vi "COD主界面（列队使用）.vi"() -> (8 "多列列表框":i32(listbox))   [LabVIEW 2016, in "斯坦道CODMn.lvlib"]
uses:
  <vilib>/Analysis/6fits.llb/Curve Fitting Criteria.ctl
  <vilib>/Utility/miscctls.llb/LVPointTypeDef.ctl
  <vilib>/Utility/config.llb/Read Key (I32).vi
  <vilib>/Utility/config.llb/Read Key (Double).vi
  <vilib>/Utility/config.llb/Read Key (Boolean).vi
  <vilib>/Utility/config.llb/Write Key (I32).vi
  <vilib>/Utility/config.llb/Read Key (String).vi
  <vilib>/Utility/config.llb/Write Key (Double).vi
  <vilib>/Utility/config.llb/Write Key (Boolean).vi
  <vilib>/Utility/config.llb/Write Key (String).vi
  <vilib>/Waveform/WDTFileIO.llb/Read Waveform from File.vi
  <vilib>/ptbypt/NI_PtbyPt.lvlib
  <vilib>/Utility/config.llb/NI_LVConfig.lvlib
  <vilib>/Analysis/NI_AALPro.lvlib
panel:
  in  "零点液自动补测":bool
  in  "跨度液自动补测":bool
  in  "标准液自动补测":bool
  in  "零点液偏差":dbl
  in  "跨度液偏差":dbl
  in  "标准液偏差":dbl
  in  "更换泵管":bool
  out "消解压力kPa":dbl format="%#.2f"
  out "权限等级":string
  in  "布尔":bool
  in  "屏蔽负值":bool
  in  "方程系数 2":cluster{"K":dbl, "b":dbl, "X^2":dbl} {"X^2" format="%#.6g"; "b" format="%#.6g"; "K" format="%#.6g"}
  out "r^2 2":dbl caption="r^2" format="%.8g"
  out "拟合公式 2":string
  in  "跨度值":dbl
  in  "公式切换阈值滴定数(0-9999)":u16
  out "公式系数":dbl[](array[numeric])
  in  "存校准信息":bool
  out "标液校准时间4":timestamp format="%<%Y/%m/%d %H:%M:%S>T"
  out "标液校准时间3":timestamp format="%<%Y/%m/%d %H:%M:%S>T"
  out "标液校准时间2":timestamp format="%<%Y/%m/%d %H:%M:%S>T"
  out "标液校准时间1":timestamp format="%<%Y/%m/%d %H:%M:%S>T"
  out "零点校准时间":timestamp format="%<%Y/%m/%d %H:%M:%S>T"
  in  "远程标样校准":enum16{"标液1", "标液2", "标液3", "标液4"}(ring)
  in  "远程校准量程":enum16{"低量程", "高量程"}(ring)
  in  "温度曲线":bool
  out "温度波形时间":timestamp
  in  "历史波形 2":bool
  out "时间-温度":u16[](array[numeric]) caption="数组"
  in  "关闭 4":bool
  out "时间温度曲线":u16[](graph)
  in  "加标回收量程：":enum32{"H", "L", "AUTO"}(ring)=enum."AUTO"
  in  "定时设置":cluster{"启动":bool, "控制命令":T1, "测量参数":T2}(xcontrol)
  out "氢氧化钠":dbl
  in  "序列号变更":bool
  out "模块版本号":string
  in  "更新程序":bool
  out "进样无液体告警":bool
  out "校准内容显示":string
  out "60分钟超时报警":bool
  in  "仪器参数":bool
  out "CODMn序列号":string
  out "CODMn软件版本：":string
  in  "标样核查量程选择":enum32{"H", "L", "AUTO"}(ring)=enum."AUTO"
  in  "标样浓度":dbl
  in  "零点核查量程选择":enum32{"H", "L", "AUTO"}(ring)=enum."AUTO"
  in  "零点核查浓度":dbl
  out "序列号":string
  in  "采水泵排液时间/s:":i32
  in  "采水泵润洗时间/s:":i32
  in  "采水泵沉淀时间/s:":i32
  in  "采水泵进样时间/s:":i32
  in  "常规版/认证版":enum16{"常规版-酸性", "常规版-碱性", "认证版", "浮台版"}(ring)
  in  "释放串口":bool
  in  "打开串口":bool
  in  "保存参数":dbl[](array[numeric])
  out "报警数字":i16
  out "CODMn工作状态":T3(ring)
  out "ORP-K":string
  out "ORP-B":string
  out "ORP-A":string
  out "稀释倍数解释":string
  in  "跨度量程选择":enum32{"H", "L", "AUTO"}(ring)=enum."AUTO"
  in  "跨度液浓度":dbl
  in  "水样：":dbl
  in  "蒸馏水：":dbl
  in  "标液：":dbl
  in  "零点核查样：":dbl
  in  "加标回收样：":dbl
  in  "草酸钠":dbl
  in  "高锰酸钾":dbl
  in  "硫酸":dbl
  out "量程解释说明":string
  in  "高切低阈值:":dbl
  in  "低切高阈值:":dbl
  in  "水样量程选择:":enum16{"L", "H", "自动切换测一次", "自动切换测两次"}(ring)
  in  "氢氧化钠：":dbl
  in  "标准液浓度":dbl
  in  "温度":dbl
  in  "恒温时间":dbl
  in  "当前量程：":enum16{"L", "H"}(ring)
  in  "CODMn零点核查选择":enum16{"零点核查走纯水管", "零点核查走零漂管"}(ring)
  in  "低量程稀释倍数:":i8=1
  in  "高量程稀释倍数:":i8=2
  out "基本量程(显示)":string
  out "测量模式(显示)":string
  out "数据时间":string
  out "断电排液标记":bool
  out "COM":string
  in  "启用5":bool
  in  "校准5":bool
  in  "泵滴定数5":dbl
  in  "浓度5":dbl
  in  "启用4":bool
  in  "校准4":bool
  in  "泵滴定数4":dbl
  in  "浓度4":dbl
  out "波形时间":timestamp
  in  "历史波形":bool
  out "滴定数-ORP值":u16[](array[numeric]) caption="数组"
  in  "关闭 3":bool
  in  "滴定曲线":bool
  out "ORP滴定曲线":u16[](graph)
  out "空白测试标记":bool
  out "跨度核查标记":bool
  in  "量程选择":enum16{"低量程", "高量程"}(ring)
  in  "手动控制":bool
  in  "选用水样":enum16{"葡萄糖", "草酸钠"}(ring)
  in  "方程系数":cluster{"K":dbl, "b":dbl, "X^2":dbl} {"X^2" format="%#.6g"; "b" format="%#.6g"; "K" format="%#.6g"}
  out "XY图":cluster{"X Values":dbl[], "Y Values":dbl[]}[](graph)
  in  "模型":enum32{"线性", "多项式", "折线"}(ring)
  out "启动时间":timestamp format="%<%Y/%m/%d %H:%M:%S>T"
  out "r^2":dbl format="%.8g"
  out "拟合公式":string
  in  "启用3":bool
  in  "启用2":bool
  in  "启用1":bool
  in  "校准3":bool
  in  "校准2":bool
  in  "校准1":bool
  in  "泵滴定数3":dbl
  in  "泵滴定数2":dbl
  in  "泵滴定数1":dbl
  in  "浓度3":dbl
  in  "浓度2":dbl
  in  "浓度1":dbl
  in  "写入":bool
  out "零点核查标记":bool
  out "排液故障":bool
  out "进水样超量程":bool
  out "标样核查标记":bool
  out "平行样测量":bool
  out "加标回收测量":bool
  out "质控样测量":bool
  out "待机":bool
  out "校标错误":bool
  out "校零错误":bool
  out "测量错误":bool
  out "草酸钠报警":bool
  out "高锰酸钾报警":bool
  out "加热故障":bool
  out "温控器故障":bool
  out "ORP故障":bool
  out "排液标记":bool
  out "故障标记":bool
  out "校标标记":bool
  out "校零标记":bool
  out "通讯状态":bool
  out "水样测量":bool
  in  "读取":bool
  in  "返回":bool
  in  "校准配置":bool
  in  "零点泵计量数 2":dbl
  in  "标度泵计量数 2":dbl
  out "标度滴定值":dbl
  out "零点滴定值":dbl
  in  "保存":bool
  in  "关闭":bool
  out "仪器时间":timestamp format="%<%Y/%m/%d %H:%M:%S>T"
  out "秒":u16
  out "分":u16
  out "COD浓度（mg/L)":dbl format="%.2g"
  out "进样管":dbl
  out "高锰酸钾":dbl
  out "草酸钠":dbl
  out "硫酸":dbl
  out "实时ORP":dbl
  out "消解温度℃":dbl
  out "加热":bool
  out "搅拌":bool
  out "进硫酸":bool
  out "进加标回收样":bool
  out "进零点核查样":bool
  out "进标液":bool
  out "进蒸馏水":bool
  out "进水样":bool
  out "进草酸钠":bool
  out "进高锰酸钾":bool
  in  "启动":bool
  in  "故障清除":bool
  in  "参数配置":bool
  in  "停止":bool
  in  "单步启动":bool
  out "系统时间":timestamp
  in  "时间校准":bool
  out "模式（受控）":u16
  # "测试时长："
  # "注：遇到加热故障和排液故障时仪器不能正常启动，\n必须排查故障并点击报警清除按钮方可运行。"
  # "mg/L"
  # "基本参数设置"
  # "校零校标结果"
  # "泵计量参数设置"
  # "校零结果："
  # "校零滴定值："
  # "高锰酸钾："
  # "加热恒温温度(℃):"
  # "草酸钠："
  # "校标结果："
  # "标度滴定值："
  # "恒温时间(分钟):"
  # "零点泵计量值："
  # "硫酸："
  # "标准液浓度(mg/L):"
  # "标度泵计量值："
  # "跨度核查浓度："
  # "跨度核查量程："
  # "日质控自动补测设置"
  # "标准液偏差±:"
  # "零点核查浓度："
  # "标样浓度："
  # "跨度液偏差%:"
  # "零点核查量程："
  # "标样核查量程："
  # "零点液偏差%:"
  # "跨度值:"
  # "校准配置界面"
  # "测量信号值"
  # "启用"
  # "校准时间"
  # "浓度"
  # "零点"
  # "标液1"
  # "标液2"
  # "标液3"
  # "标液4"
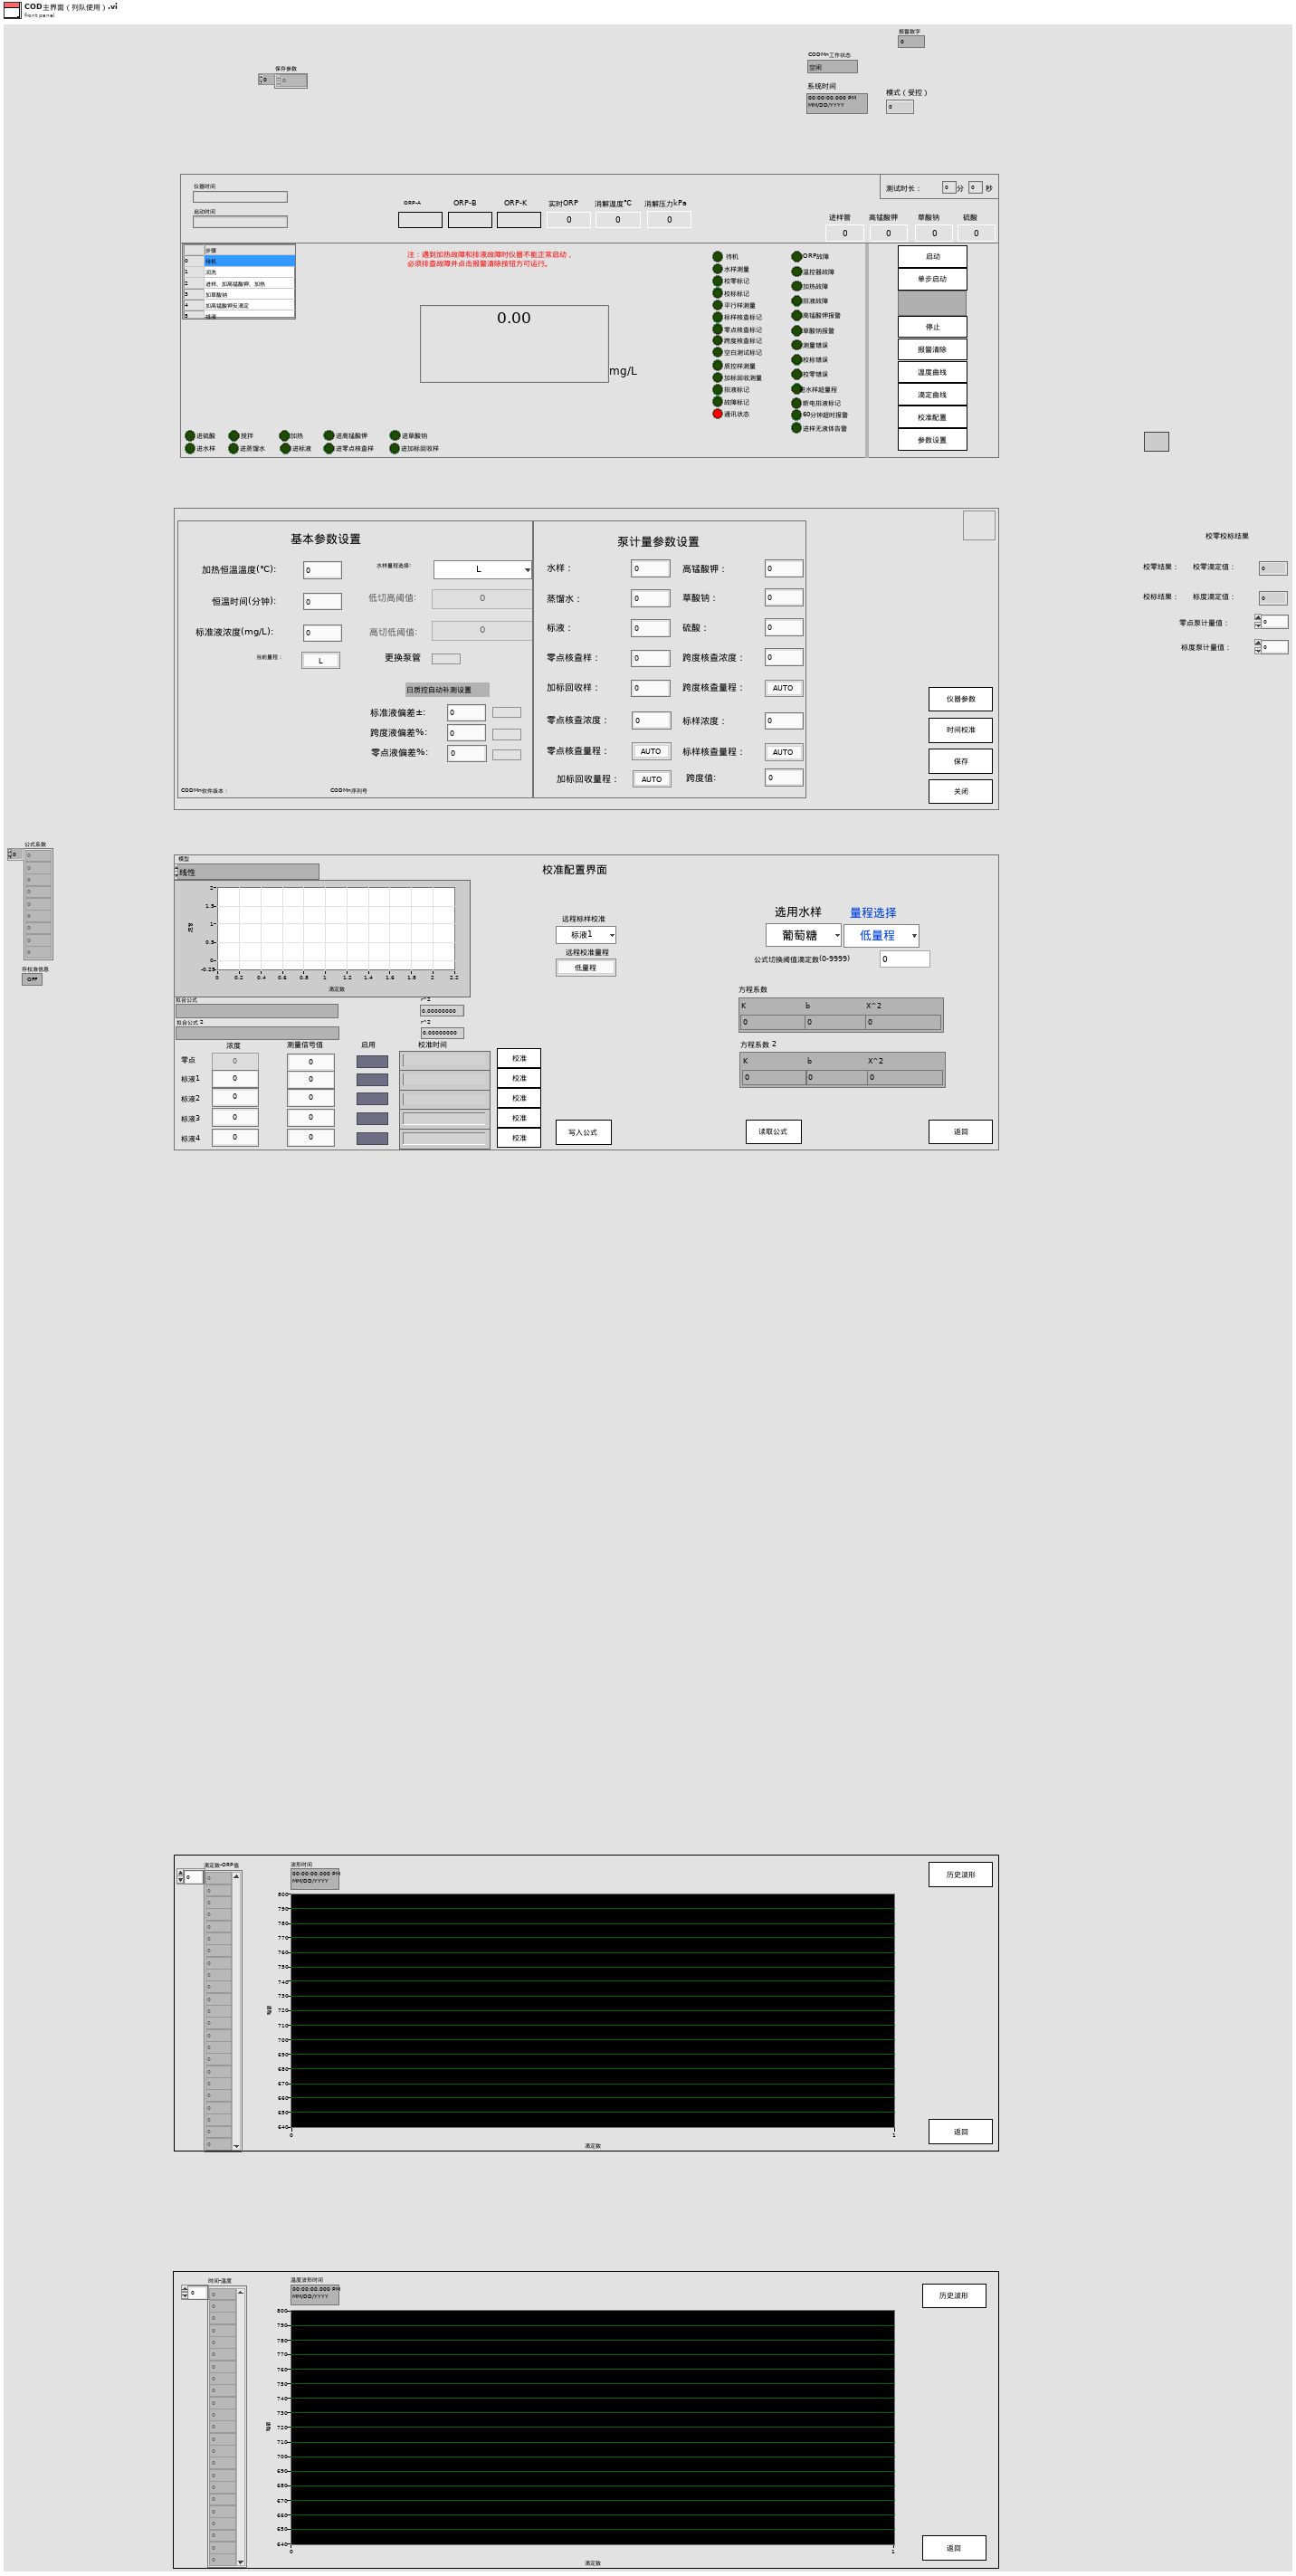
[diagram p1: front panel]
types:
  T1 = typedef "定时设置.xctl/国标控制命令.ctl" = enum16{"启动测量", "标样核查", "零点核查", "跨度核查", "空白测试", "平行样测试", "加标回收", "空白校准", "标样校准", "初始化（清洗）", "停止测试", "仪器重启", "校时", "模式设置", "测量间隔设置"}
  T2 = typedef "定时设置.xctl/测量参数.ctl" = u16
  T3 = enum16{"空闲", "水样测试", "标样核查", "零点核查", "跨度核查", "空白测试", "平行样测试", "质控样", "空白校准", "标样校准", "加标回收"}
  T4 = cluster{"运行模式":enum16{"维护模式", "常规模式", "应急模式", "质控模式"}, "质控频次":enum16{"关闭", "每天", "星期一", "星期二", "星期三", "星期四", "星期五", "星期六", "星期日"}, "空白核查时间":u16, "跨度核查时间":u16, "测量间隔":u16}
  T5 = cluster{"测量量程":dbl, "测量精度":dbl, "测量间隔":dbl, "消解温度":dbl, "消解时长":dbl, "空白校准时间":timestamp, "曲线截距":dbl, "曲线斜率":dbl, "测量检出限":dbl, "测量信号值":dbl, "线性相关系数":dbl, "二次多项式系数":dbl, "标样校准时间":timestamp, "稀释倍数":dbl, "三项式系数":dbl, "空白标定系数":dbl, "量程系数":dbl, "F0/ORPA":dbl, "F1/ORPB":dbl, "F2/ORPK":dbl, "F3":dbl, "F4":dbl, "F5":dbl, "F6":dbl, "F7":dbl, "X0/滴定数":dbl, "量程":dbl}
  T6 = typedef "LVPointTypeDef.ctl" = cluster{"Horizontal":i16, "Vertical":i16}
  T7 = cluster{"Major":u16, "Minor":u16, "Fix":u16, "Build":u16}
  T8 = typedef "NI_LVConfig.lvlib/Config Data RefNum.ctl" = refnum<k1>
  T9 = enum8{"Enabled", "Disabled", "Disabled and Grayed Out"}
  T10 = cluster{"时间":timestamp, "测量模式":string, "数据类型":string, "检测值":sgl, "单位":string, "数据标识":string, "因子编码":string, "标样参考值":sgl, "ORP-A":sgl, "ORP-B":sgl, "ORP-K":sgl, "COD滴定值":sgl, "高锰酸钾滴定数":sgl, "温度":sgl, "量程":sgl, "LastTime":timestamp, "序列号:":string, "跨度值":sgl, "高锰酸钾原始滴定数":sgl}
  T11 = cluster{"因子编码":u32, "单位":u16, "标样参考值":sgl, "水样数据时间":timestamp, "水样实测值":sgl, "水样数据标识":string, "标样数据时间":timestamp, "标样实测值":sgl, "标样数据标识":string, "空白数据时间":timestamp, "空白实测值":sgl, "空白数据标识":string, "零点核查数据时间":timestamp, "零点核查实测值":sgl, "零点核查数据标识":string, "跨度核查数据时间":timestamp, "跨度核查实测值":sgl, "跨度核查数据标识":string, "加标回收数据时间":timestamp, "加标回收实测值":sgl, "加标回收数据标识":string, "平行样数据时间":timestamp, "平行样实测值":sgl, "平行样数据标识":string}
  T12 = cluster{"数组 2[0]":sgl, "数组 2[1]":sgl, "数组 2[2]":sgl, "数组 2[3]":sgl, "数组 2[4]":sgl, "数组 2[5]":sgl, "数组 2[6]":sgl, "数组 2[7]":sgl, "数组 2[8]":sgl, "数组 2[9]":sgl, "数组 2[10]":sgl, "数组 2[11]":sgl, "数组 2[12]":sgl, "数组 2[13]":sgl, "数组 2[14]":sgl, "数组 2[15]":sgl, "数组 2[16]":sgl, "数组 2[17]":sgl, "数组 2[18]":sgl, "数组 2[19]":sgl, "数组 2[20]":sgl, "数组 2[21]":sgl, "数组 2[22]":sgl, "数组 2[23]":sgl, "数组 2[24]":sgl, "数组 2[25]":sgl, "数组 2[26]":sgl, "数组 2[27]":sgl, "数组 2[28]":sgl, "数组 2[29]":sgl, "数组 2[30]":sgl, "数组 2[31]":sgl, "数组 2[32]":sgl, "数组 2[33]":sgl, "数组 2[34]":sgl, "数组 2[35]":sgl, "数组 2[36]":sgl, "数组 2[37]":sgl, "数组 2[38]":sgl, "数组 2[39]":sgl, "数组 2[40]":sgl, "数组 2[41]":sgl}
  T13 = typedef "NI_AALPro.lvlib/Curve Fitting Criteria.ctl" = u16
  T14 = cluster{"ORP故障":bool, "温控器故障":bool, "加热故障":bool, "高锰酸钾报警":bool, "草酸钠报警":bool, "测量错误":bool, "校零错误":bool, "校标错误":bool, " 进水样超量程":bool, "排液阀故障":bool, "60分钟超时报警":bool, "进样无液体报警":bool}
  T15 = cluster{"时间":timestamp, "水样计量数":u16, "蒸馏水计量数":u16, "标液计量数":u16, "零点核查计量数":u16, "加标回收计量数":u16, "硫酸计量数":u16, "高锰酸钾计量数":u16, "草酸钠计量数":u16, "更换泵管":string}
  T16 = typedef "数据库类型.ctl" = enum16{"Access", "SQLite"}
  T17 = cluster{"确定":bool, "测量量程":dbl, "测量精度":dbl, "测量间隔":dbl, "消解温度":dbl, "消解时长":dbl, "空白校准时间":timestamp, "曲线截距":dbl, "曲线斜率":dbl, "测量检出限":dbl, "测量信号值":dbl, "线性相关系数":dbl, "二次多项式系数":dbl, "标样校准时间":timestamp, "稀释倍数":dbl, "三项式系数":dbl, "空白标定系数":dbl, "量程系数":dbl, "F0/ORPA":dbl, "F1/ORPB":dbl, "F2/ORPK":dbl, "F3":dbl, "F4":dbl, "F5":dbl, "F6":dbl, "F7":dbl, "X0/滴定数":dbl, "量程":dbl}
  T18 = cluster{"[0]":string, "[1]":string, "[2]":string}
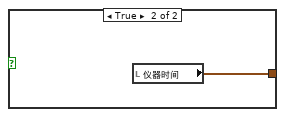
[diagram p6: hidden frame]
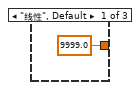
[diagram p10: hidden frame]
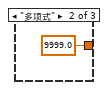
[diagram p11: hidden frame]
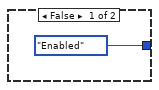
[diagram p12: hidden frame]
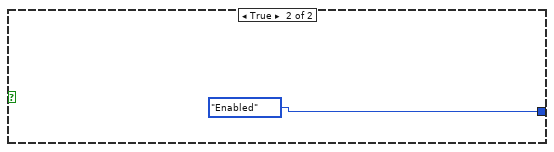
[diagram p13: hidden frame]
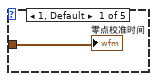
[diagram p18: hidden frame]
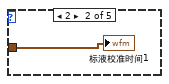
[diagram p19: hidden frame]
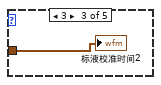
[diagram p20: hidden frame]
diagram:
  n1 = property on="定时设置" class="定时设置 (严格)"("调用模块名称写入"="CODMn" ("引用参数")) -> (error out=w3:errorcluster)  [unwired: 2 in, 1 out]
  n2 = flat-sequence {
    tunnel: w5 -> [_]
    frame #0 {
      n3 = vi-ref "斯坦道CODMn.lvlib:待机状态数据存储写入和切换量程(子VI).vi"() -> (w66:refnum<vi>)
      n4 = vi-ref "斯坦道CODMn.lvlib:日志报警状态存储 (子VI).vi"() -> (w59:refnum<vi>)
      n5 = vi-ref "斯坦道CODMn.lvlib:高锰酸钾-ORP滴定曲线(子VI).vi"() -> (w46:refnum<vi>)
      n6 = property class="VI"(reference=w59, error in=errorcluster {"status"=FALSE, "code"=0, "source"=""} ("错误输出")) -> ("Name"=w58:string)  [unwired: 2 out]
      n7 = property class="VI"(reference=w46, error in=errorcluster {"status"=FALSE, "code"=0, "source"=""} ("错误输出")) -> ("Name"=w47:string)  [unwired: 2 out]
      n8 = property class="VI"(reference=w66, error in=errorcluster {"status"=FALSE, "code"=0, "source"=""} ("错误输出")) -> ("Name"=w65:string)  [unwired: 2 out]
      n9 = Open VI Reference(type specifier VI Refnum (for type only)=refnum<vi> refnum, vi path=w58, options=128 ("选项")) -> (vi reference=w42:refnum<vi>, error out=w56:errorcluster)  [unwired: 3 in]
      n10 = Open VI Reference(type specifier VI Refnum (for type only)=refnum<vi> refnum, vi path=w47, options=128 ("选项")) -> (vi reference=w45:refnum<vi>, error out=w49:errorcluster)  [unwired: 3 in]
      n11 = call-by-ref "?"(reference=w42, error in=w56) -> (reference out=w54:refnum<vi>, error out=w55:errorcluster)  [unwired: 12 in]
      n12 = call-by-ref "?"(reference=w45, error in=w49) -> (reference out=w51:refnum<vi>, error out=w50:errorcluster)  [unwired: 12 in]
      n13 = Open VI Reference(type specifier VI Refnum (for type only)=refnum<vi> refnum, vi path=w65, options=128 ("选项")) -> (vi reference=w40:refnum<vi>, error out=w63:errorcluster)  [unwired: 3 in]
      n14 = Close Reference(reference=w54, error in (no error)=w55) -> ()  [unwired: 1 out]
      n15 = call-by-ref "?"(reference=w40, error in=w63) -> (reference out=w61:refnum<vi>, error out=w62:errorcluster)  [unwired: 12 in]
      n16 = Close Reference(reference=w51, error in (no error)=w50) -> ()  [unwired: 1 out]
      n17 = Close Reference(reference=w61, error in (no error)=w62) -> ()  [unwired: 1 out]
      n18 = vi-ref "斯坦道CODMn.lvlib:时间-温度曲线(子VI).vi"() -> (w28:refnum<vi>)
      n19 = vi-ref "斯坦道CODMn.lvlib:关键参数交互.vi"() -> (w37:refnum<vi>)
      n20 = property class="VI"(reference=w37, error in=errorcluster {"status"=FALSE, "code"=0, "source"=""} ("错误输出")) -> ("Name"=w36:string)  [unwired: 2 out]
      n21 = property class="VI"(reference=w28, error in=errorcluster {"status"=FALSE, "code"=0, "source"=""} ("错误输出")) -> ("Name"=w27:string)  [unwired: 2 out]
      n22 = Open VI Reference(type specifier VI Refnum (for type only)=refnum<vi> refnum, vi path=w36, options=128 ("选项")) -> (vi reference=w38:refnum<vi>, error out=w34:errorcluster)  [unwired: 3 in]
      n23 = call-by-ref "?"(reference=w38, error in=w34, "量程选择"=enum16{"低量程", "高量程"}."低量程", "模型"=enum32{"线性", "多项式", "折线"}."线性") -> (reference out=w32:refnum<vi>, error out=w33:errorcluster)  [unwired: 10 in]
      n24 = Open VI Reference(type specifier VI Refnum (for type only)=refnum<vi> refnum, vi path=w27, options=128 ("选项")) -> (vi reference=w29:refnum<vi>, error out=w25:errorcluster)  [unwired: 3 in]
      n25 = call-by-ref "?"(reference=w29, error in=w25) -> (reference out=w23:refnum<vi>, error out=w24:errorcluster)  [unwired: 12 in]
      n26 = Close Reference(reference=w32, error in (no error)=w33) -> ()  [unwired: 1 out]
      n27 = Close Reference(reference=w23, error in (no error)=w24) -> ()  [unwired: 1 out]
    }
  }
  n28 = call "taskqueue ref.vi"() -> ("队列输出"=w2:refnum<queue>)  [unwired: 10 in, 1 out]
  n29 = while {
    tunnel: w3 -> [_]
    tunnel: w2 -> [w79]
    shift-right: [w71] -> _
    shift-left: 0 -> [w70]
    stop <- FALSE stop-if-true
    n30 = Quotient & Remainder(x=w70, y=30) -> (x-y*floor(x/y)=w68:i32)  [unwired: 1 out]
    n31 = Wait (ms)(milliseconds to wait=u32 500 ("等待时间（毫秒）")) -> ()  [unwired: 1 out]
    n32 = global read "CODMn断电保存全局变量.vi" "运行周期"() -> (w81:T4)
    n33 = local read "通讯状态"() -> (w84:bool)
    n34 = Unbundle By Name("定时设置") -> ("启动"=w74:bool, "控制命令"=w78:T1)
    n35 = Equal To 0?(x=w68) -> (x = 0?=w75:bool)
    n36 = Increment(x=w70) -> (x+1=w73:i32)
    n37 = global read "CODMn断电保存全局变量.vi" "CODMn仪器参数"() -> (w83:T5)
    n38 = case shown="假" w84 {
      tunnel: [w97 w98] -> w67
      frame False {
        n39 = Get Date/Time In Seconds() -> (seconds since 1Jan1904=w97:timestamp)
      }
      frame True {
        n40 = local read "仪器时间"() -> (w98:timestamp)
      }
    }
    n41 = Unbundle By Name(w81) -> ("测量间隔"=w80:u16)
    n42 = And(x=w74, y=w75) -> (x .and. y?=w77:bool)
    n43 = Select(t=w73, s=w74, f=0) -> (s? t:f=w71:i32)
    n44 = Bundle By Name(cluster=w83, "测量间隔"=w80) -> (w82:T5)
    n45 = case shown="真" w77 {
      tunnel: w79 -> [_ w94]
      tunnel: w78 -> [_ w93]
      frame False {
      }
      frame True {
        n46 = Get Queue Status(queue=w94) -> (queue out=w92:refnum<queue>, # elements in queue=w91:i32)  [unwired: 2 in, 6 out]
        n47 = Equal To 0?(x=w91) -> (x = 0?=w90:bool)
        n48 = case shown="真" w90 {
          tunnel: w93 -> [_ w96]
          tunnel: w92 -> [_ w95]
          frame False {
          }
          frame True {
            n49 = Enqueue Element(queue=w95, element=w96) -> ()  [unwired: 2 in, 3 out]
          }
        }
      }
    }
    n50 = global write "CODMn断电保存全局变量.vi" "CODMn仪器参数"(w82) -> ()
    n51 = global read "COD测量模式全局.vi" "CODMn工作状态"() -> (w76:T3)
    n52 = Not Equal?(x=w76, y=T3."空闲") -> (x != y?=w85:bool)
    n53 = property on="定时设置" class="定时设置 (严格)"("仪器状态"=w85, "仪器时间写入"=w67) -> ()  [unwired: 2 in, 2 out]
  }
  n54 = flat-sequence {
    tunnel: [w102] -> w7
    tunnel: [errorcluster {"status"=FALSE, "code"=0, "source"=""} ("错误输出")] -> w5
    tunnel: [w104] -> w6
    frame #0 {
      w126 = "192.168.1.100" ("名称")
      n55 = global write "COD内部交互全局.vi" "量程切换次数"(u8 0 ("量程切换次数")) -> ()
      n56 = global write "COD内部交互全局.vi" "切换量程连续测两次"(FALSE ("切换量程连续测两次")) -> ()
      n57 = global read "COD内部交互全局.vi" "序列号:"() -> (w133:string)
      n58 = property on="窗格" class="Pane"("Origin"=T6 {"Horizontal"=0, "Vertical"=0} ("原点")) -> ()  [unwired: 2 in, 2 out]
      n59 = Empty String/Path?(string/path=w133) -> (empty?=w101:bool)
      n60 = case shown="真" w101 {
        tunnel: w133 -> [w147 _]
        tunnel: [w146 "data\\CODMnSet.ini" ("名称或相对路径")] -> w114
        frame False {
          # "与生产用上位机交互"
          n61 = Concatenate Strings("data\\" ("字符串"), "序列号" ("字符串"), w147, "Set.ini" ("名称或相对路径")) -> (w146:string)
        }
        frame True {
        }
      }
      n62 = String To IP(1:w126) -> (0:w119:u32)
      n63 = IP To String(2:w119) -> (0:w122:string)  [unwired: 1 in]
      n64 = Not Equal?(x=w126, y=w122) -> (x != y?=w127:bool)
      n65 = Concatenate Strings("\\\\" ("字符串"), w122) -> (w121:string)
      n66 = global write "CODMN外部API.vi" "ping"(w127) -> ()
      n67 = String To Path(string=w121) -> (path=w128:path)
      n68 = Build Path(base path=w128, name or relative path=w114) -> (appended path=w123:path)
      n69 = local write "量程选择"(enum16{"低量程", "高量程"}."低量程" ("量程选择")) -> ()
      n70 = local write "选用水样"(enum16{"葡萄糖", "草酸钠"}."葡萄糖" ("选用水样")) -> ()
      n71 = global write "COD内部交互全局.vi" "配置文件ini"(w114) -> ()
      n72 = case shown="真" w127 {
        tunnel: w123 -> [w137 w141]
        tunnel: [w137 w140] -> w124
        tunnel: [FALSE w139] -> w125
        frame False {
        }
        frame True {
          n73 = call <vilib>:"Check if File or Folder Exists.vi"("path"=w141) -> ("file or folder exists?"=w139:bool, "dup path"=w140:path)  [unwired: 8 in, 1 out]
        }
      }
      n74 = control-ref of="本VI"() -> (w113:refnum<vi>)
      n75 = case shown="假" w125 {
        tunnel: w124 -> [_ w145]
        tunnel: [w143 w145] -> w105
        tunnel: w114 -> [w142 _]
        frame False {
          # "本地文件地址"
          n76 = call <vilib>:"Application Directory.vi"() -> ("Application Directory"=w144:path)
          n77 = Build Path(base path=w144, name or relative path=w142) -> (appended path=w143:path)
        }
        frame True {
          # "网络共享地址"
        }
      }
      n78 = property class="VI"(reference=w113) -> ("Library.Version"=w112:T7)  [unwired: 1 in, 2 out]
      n79 = Unbundle By Name(w112) -> ("Major"=w110:u16, "Minor"=w109:u16, "Fix"=w108:u16, "Build"=w107:u16)
      n80 = Format Into String(format string="模块版本号：%d.%d.%d.%d" ("格式字符串"), w110, w109, w108, w107) -> (resulting string=→"模块版本号":string)  [unwired: 2 in, 1 out]
      n81 = global write "CODMN外部API.vi" "配置文件 path"(w105) -> ()
      n82 = call <vilib>:"Open Config Data.vi"("configuration file path"=w105) -> ("error out"=w115:errorcluster, "refnum"=w116:T8)  [unwired: 8 in, 1 out]
      n83 = vi-ref "斯坦道CODMn.lvlib:CODMn断电保存全局变量.vi"() -> (w129:refnum<vi>)
      n84 = call <userlib>:"Read Panel from INI__ogtk.vi"("error in (no error)"=w115, "VI ref"=w129, "refnum"=w116) -> ("error out"=w117:errorcluster, "refnum out"=w118:T8)  [unwired: 7 in]
      n85 = call <vilib>:"Close Config Data.vi"("error in (no error)"=w117, "refnum"=w118) -> ("error out"=w103:errorcluster)  [unwired: 8 in, 1 out]
      n86 = call <vilib>:"Clear Errors.vi"("error in (no error)"=w103) -> ("error out"=w100:errorcluster)  [unwired: 5 in, 1 out]
      n87 = Read from Text File(file (use dialog)=w105, error in=w100) -> (text=w104:string, error out=w102:errorcluster)  [unwired: 2 in, 2 out]
      "稀释倍数解释" <- "稀释倍数解释：\n稀释倍数选择1，表示不稀释\n默认低量程系数倍数1，高量程系数倍数2\n则低量程为0~8，高量程为0~16" ("稀释倍数解释")
    }
  }
  n88 = call "task.vi"() -> ()  [unwired: 12 in]
  n89 = Obtain Queue(name (unnamed)="CODMn" ("名称（未命名）"), element data type=cluster{"命令":string} {"命令"="启用模块"} ("元素")) -> (queue out=w17:refnum<queue>, error out=w16:errorcluster)  [unwired: 3 in, 1 out]
  n90 = while {
    tunnel: [w158] -> _
    shift-right: [w156] -> _
    shift-left: w6 -> [w155]
    tunnel: w7 -> [_]
    stop <- FALSE stop-if-true
    n91 = global read "CODMN外部API.vi" "配置文件 path"() -> (w152:path)
    n92 = Wait (ms)(milliseconds to wait=u32 1000 ("等待时间（毫秒）")) -> ()  [unwired: 1 out]
    n93 = Read from Text File(file (use dialog)=w152) -> (text=w156:string, error out=w153:errorcluster)  [unwired: 3 in, 2 out]
    n94 = Not Equal?(x=w156, y=w155) -> (x != y?=w154:bool)
    n95 = case shown="真" w154 {
      tunnel: [w160 w167] -> w158
      tunnel: w152 -> [_ w161]
      tunnel: w153 -> [w160 _]
      frame False {
      }
      frame True {
        # "文件发生改变进行更新，远端和本地都更新"
        n96 = vi-ref "斯坦道CODMn.lvlib:CODMn断电保存全局变量.vi"() -> (w162:refnum<vi>)
        n97 = call <vilib>:"Open Config Data.vi"("configuration file path"=w161) -> ("error out"=w166:errorcluster, "refnum"=w165:T8)  [unwired: 8 in, 1 out]
        n98 = call <userlib>:"Read Panel from INI__ogtk.vi"("error in (no error)"=w166, "VI ref"=w162, "refnum"=w165) -> ("error out"=w164:errorcluster, "refnum out"=w163:T8)  [unwired: 7 in]
        n99 = call <vilib>:"Close Config Data.vi"("error in (no error)"=w164, "refnum"=w163) -> ("error out"=w167:errorcluster)  [unwired: 8 in, 1 out]
      }
    }
  }
  n100 = vi-ref "CODMn通讯.vi"() -> (w8:refnum<vi>)
  n101 = while {
    stop <- FALSE stop-if-true
    n102 = global read "COD内部交互全局.vi" "待机"() -> (w169:bool)
    n103 = Wait (ms)(milliseconds to wait=u32 1000 ("等待时间（毫秒）")) -> ()  [unwired: 1 out]
    n104 = case shown="假" w169 {
      tunnel: [w186 T9."Enabled" ("禁用")] -> w171
      tunnel: [w185 _] -> w170
      frame False {
        # "运行中"
        n105 = local read "校标标记"() -> (w184:bool)
        n106 = local read "校零标记"() -> (w183:bool)
        n107 = Or(x=w184, y=w183) -> (x .or. y?=w187:bool)
        n108 = case shown="真" w187 {
          tunnel: [T9."Enabled" ("禁用") T9."Disabled and Grayed Out" ("禁用")] -> w186
          tunnel: [_ TRUE] -> w185
          frame False {
          }
          frame True {
          }
        }
      }
      frame True {
      }
    }
    n109 = control-ref of="量程选择"() -> (w177:refnum<vi>)
    n110 = property on="校准内容显示" class="Str"("Visible"=w170) -> ()  [unwired: 2 in, 2 out]
    n111 = control-ref of="选用水样"() -> (w178:refnum<vi>)
    n112 = control-ref of="校准5"() -> (w172:refnum<vi>)
    n113 = control-ref of="校准4"() -> (w173:refnum<vi>)
    n114 = control-ref of="校准3"() -> (w174:refnum<vi>)
    n115 = control-ref of="校准2"() -> (w175:refnum<vi>)
    n116 = control-ref of="校准1"() -> (w176:refnum<vi>)
    n117 = Build Array(w172, w173, w174, w175, w176, w178, w177) -> (w179:refnum<vi>[])
    n118 = for {
      tunnel: w179 -> [w182] mode=indexing
      tunnel: w171 -> [w181]
      n119 = property class="Ctl"(reference=w182, "DisabledEnum"=w181) -> ()  [unwired: 1 in, 2 out]
    }
  }
  n120 = while {
    tunnel: w7 -> [_]
    stop <- FALSE stop-if-true
    # "赋值循环"
    n121 = flat-sequence {
      frame #0 {
        # "测量数据区"
        n122 = global read "COD内部交互全局.vi" "data"() -> (w334:T10)
        n123 = global read "COD测量模式全局.vi" "测量模式文字实时"() -> (w320:string)
        "测量模式(显示)" <- w320
        n124 = global read "CODMn断电保存全局变量.vi" "测量数据区"() -> (w329:T11)
        n125 = Unbundle By Name(w334) -> ("时间"=w333:timestamp, "检测值"=w332:sgl, "数据标识"=w331:string)
        n126 = case shown="\"水样测试\"" w320 {
          tunnel: w329 -> [w335 w340 w345 w350 w355 w360 w365 w370 w375 w380]
          tunnel: [w335 w339 w344 w346 w354 w359 w364 w369 w371 w379] -> w330
          tunnel: w333 -> [_ w338 w343 w349 w353 w358 w363 w368 w374 w378]
          tunnel: w332 -> [_ w337 w342 w348 w352 w357 w362 w367 w373 w377]
          tunnel: w331 -> [_ w336 w341 w347 w351 w356 w361 w366 w372 w376]
          frame "", Default {
          }
          frame "水样测试" {
            n127 = Bundle By Name(cluster=w340, "水样数据时间"=w338, "水样实测值"=w337, "水样数据标识"=w336) -> (w339:T11)
          }
          frame "标样核查" {
            n128 = Bundle By Name(cluster=w345, "标样数据时间"=w343, "标样实测值"=w342, "标样数据标识"=w341) -> (w344:T11)
          }
          frame "跨度核查" {
            n129 = Bundle By Name(cluster=w350, "跨度核查数据时间"=w349, "跨度核查实测值"=w348, "跨度核查数据标识"=w347) -> (w346:T11)
          }
          frame "零点核查" {
            n130 = Bundle By Name(cluster=w355, "零点核查数据时间"=w353, "零点核查实测值"=w352, "零点核查数据标识"=w351) -> (w354:T11)
          }
          frame "空白测试" {
            n131 = Bundle By Name(cluster=w360, "空白数据时间"=w358, "空白实测值"=w357, "空白数据标识"=w356) -> (w359:T11)
          }
          frame "加标回收" {
            n132 = Bundle By Name(cluster=w365, "加标回收数据时间"=w363, "加标回收实测值"=w362, "加标回收数据标识"=w361) -> (w364:T11)
          }
          frame "平行样" {
            n133 = Bundle By Name(cluster=w370, "平行样数据时间"=w368, "平行样实测值"=w367, "平行样数据标识"=w366) -> (w369:T11)
          }
          frame "校零" {
            n134 = Bundle By Name(cluster=w375, "空白数据时间"=w374, "空白实测值"=w373, "空白数据标识"=w372) -> (w371:T11)
          }
          frame "校标" {
            n135 = Bundle By Name(cluster=w380, "标样数据时间"=w378, "标样实测值"=w377, "标样数据标识"=w376) -> (w379:T11)
          }
        }
        n136 = Unbundle By Name(w329) -> ("水样实测值"=w326:sgl)
        n137 = feedback-in #1(w329) -> ()
        n138 = feedback #1(w329) -> (w328:T11)
        n139 = global read "CODMn断电保存全局变量.vi" "水样测试量程"() -> (w322:enum16{"L", "H"})
        n140 = global read "CODMn断电保存全局变量.vi" "测量模式"() -> (w318:string)
        n141 = Unbundle By Name(w328) -> ("水样实测值"=w327:sgl)
        n142 = feedback #2(w322) -> (w323:enum16{"L", "H"})
        n143 = feedback-in #2(w322) -> ()
        n144 = feedback #3(w318) -> (w319:string)
        n145 = feedback-in #3(w318) -> ()
        n146 = Not Equal?(x=w323, y=w322) -> (x != y?=w321:bool)
        n147 = Not Equal?(x=w319, y=w318) -> (x != y?=w317:bool)
        n148 = Not Equal?(x=w326, y=w327) -> (x != y?=w325:bool)
        n149 = global write "CODMn断电保存全局变量.vi" "测量数据区"(w330) -> ()
        n150 = Compound Arithmetic op=OR ("复合运算")(w325, w321, w317) -> (w324:bool)
        n151 = case shown="真" w324 {
          frame False {
          }
          frame True {
            # "水样值发送改变存储本地"
            n152 = call "配置文件保存.vi"() -> ()  [unwired: 12 in]
          }
        }
      }
    }
    n153 = flat-sequence {
      frame #0 {
        # "局部变量给内部交互用全局变量"
        n154 = local read "COD浓度（mg/L)"() -> (w224:dbl)
        n155 = local read "CODMn工作状态"() -> (w227:T3)
        n156 = local read "多列列表框"() -> (w225:i32)
        n157 = local read "标准液浓度"() -> (w223:dbl)
        n158 = local read "消解温度℃"() -> (w218:dbl)
        n159 = local read "高锰酸钾报警"() -> (w221:bool)
        n160 = local read "断电排液标记"() -> (w220:bool)
        n161 = local read "实时ORP"() -> (w217:dbl)
        n162 = local read "故障标记"() -> (w226:bool)
        n163 = local read "高锰酸钾"() -> (w219:dbl)
        n164 = local read "待机"() -> (w222:bool)
        n165 = global write "COD内部交互全局.vi" "实时温度"(w218) -> ()
        n166 = global write "运行时序全局变量.vi" "多列列表框"(w225) -> ()
        n167 = global write "COD内部交互全局.vi" "故障标记"(w226) -> ()
        n168 = global write "COD内部交互全局.vi" "ORP显示"(w217) -> ()
        n169 = global write "COD浓度全局变量.vi" "标准液浓度"(w223) -> ()
        n170 = global write "COD内部交互全局.vi" "高锰酸钾"(w219) -> ()
        n171 = global write "COD内部交互全局.vi" "待机"(w222) -> ()
        n172 = global write "COD测量模式全局.vi" "CODMn工作状态"(w227) -> ()
        n173 = global write "COD内部交互全局.vi" "高锰酸钾报警"(w221) -> ()
        n174 = global write "COD内部交互全局.vi" "断电排液标记"(w220) -> ()
        n175 = global write "COD浓度全局变量.vi" "COD浓度（mg/L)"(w224) -> ()
      }
    }
    n176 = flat-sequence {
      frame #0 {
        # "断电保存全局给局部变量"
        n177 = global read "CODMn断电保存全局变量.vi" "高切低阈值:"() -> (w407:dbl)
        n178 = global read "CODMn断电保存全局变量.vi" "低切高阈值:"() -> (w406:dbl)
        n179 = global read "CODMn断电保存全局变量.vi" "跨度液浓度"() -> (w404:dbl)
        n180 = global read "COD内部交互全局.vi" "波形时间"() -> (→"波形时间":timestamp)
        n181 = global read "CODMn断电保存全局变量.vi" "启动时间"() -> (→"启动时间":timestamp)
        n182 = global read "CODMn断电保存全局变量.vi" "标样浓度"() -> (w402:dbl)
        n183 = global read "CODMn断电保存全局变量.vi" "CODMn跨度量程选择"() -> (w408:enum32{"H", "L", "AUTO"})
        n184 = global read "CODMn断电保存全局变量.vi" "标样核查量程选择"() -> (w399:enum32{"H", "L", "AUTO"})
        n185 = global read "CODMn断电保存全局变量.vi" "零点核查量程选择"() -> (w401:enum32{"H", "L", "AUTO"})
        n186 = global read "CODMn断电保存全局变量.vi" "加标回收量程选择"() -> (w394:enum32{"H", "L", "AUTO"})
        n187 = global read "COD内部交互全局.vi" "滴定数-ORP值"() -> (→"滴定数-ORP值":u16[])
        n188 = global read "CODMn断电保存全局变量.vi" "常规版/认证版"() -> (w403:enum16{"常规版-酸性", "常规版-碱性", "认证版", "浮台版"})
        n189 = global read "CODMn断电保存全局变量.vi" "自动切换量程:"() -> (w405:enum16{"L", "H", "自动切换测一次", "自动切换测两次"})
        n190 = global read "CODMn断电保存全局变量.vi" "零点核查浓度"() -> (w400:dbl)
        n191 = local write "高切低阈值:"(w407) -> ()
        n192 = global read "CODMn断电保存全局变量.vi" "跨度值"() -> (w388:dbl)
        n193 = local write "跨度液浓度"(w404) -> ()
        n194 = local write "低切高阈值:"(w406) -> ()
        n195 = global read "COD内部交互全局.vi" "ORP滴定曲线"() -> (→"ORP滴定曲线":u16[])
        n196 = local write "标样浓度"(w402) -> ()
        n197 = local write "标样核查量程选择"(w399) -> ()
        n198 = local write "水样量程选择:"(w405) -> ()
        n199 = local write "常规版/认证版"(w403) -> ()
        n200 = local write "零点核查浓度"(w400) -> ()
        n201 = local write "零点核查量程选择"(w401) -> ()
        n202 = local write "加标回收量程："(w394) -> ()
        n203 = local write "跨度量程选择"(w408) -> ()
        n204 = local write "跨度值"(w388) -> ()
        n205 = global read "CODMn断电保存全局变量.vi" "标样核查自动补测"() -> (w386:bool)
        n206 = global read "CODMn断电保存全局变量.vi" "零点核查自动补测"() -> (w385:bool)
        n207 = global read "CODMn断电保存全局变量.vi" "跨度核查自动补测"() -> (w384:bool)
        n208 = global read "CODMn断电保存全局变量.vi" "远程校准量程"() -> (w389:enum16{"低量程", "高量程"})
        n209 = global read "CODMn断电保存全局变量.vi" "远程标样校准"() -> (w390:enum16{"标液1", "标液2", "标液3", "标液4"})
        n210 = global read "CODMn断电保存全局变量.vi" "标准液标准偏差"() -> (w381:dbl)
        n211 = global read "CODMn断电保存全局变量.vi" "零点标准液偏差"() -> (w382:dbl)
        n212 = global read "CODMn断电保存全局变量.vi" "跨度标准液偏差"() -> (w383:dbl)
        n213 = global read "CODMn断电保存全局变量.vi" "屏蔽负值"() -> (w387:bool)
        n214 = global read "COD内部交互全局.vi" "温度波形时间"() -> (→"温度波形时间":timestamp)
        n215 = global read "COD内部交互全局.vi" "时间温度曲线"() -> (→"时间温度曲线":u16[])
        n216 = global read "COD内部交互全局.vi" "时间-温度"() -> (→"时间-温度":u16[])
        n217 = local write "远程标样校准"(w390) -> ()
        n218 = local write "远程校准量程"(w389) -> ()
        n219 = local write "标准液自动补测"(w386) -> ()
        n220 = local write "零点液自动补测"(w385) -> ()
        n221 = local write "跨度液自动补测"(w384) -> ()
        n222 = local write "标准液偏差"(w381) -> ()
        n223 = local write "零点液偏差"(w382) -> ()
        n224 = local write "跨度液偏差"(w383) -> ()
        n225 = local write "屏蔽负值"(w387) -> ()
      }
    }
    n226 = flat-sequence {
      frame #0 {
        # "保存参数赋值"
        n227 = Multiply(x="温度", y=10.0) -> (x*y=w202:dbl)
        n228 = Multiply(x="标准液浓度", y=100.0) -> (x*y=w199:dbl)
        n229 = Build Array(w202, "恒温时间", w199, "氢氧化钠：", "当前量程：", "水样：", "蒸馏水：", "标液：", "零点核查样：", "加标回收样：", "高锰酸钾", "草酸钠", "硫酸", "零点泵计量数 2", "标度泵计量数 2", "高量程稀释倍数:", "低量程稀释倍数:", "CODMn零点核查选择") -> (w196:dbl[])
        n230 = local write "保存参数"(w196) -> ()
      }
    }
    n231 = flat-sequence {
      frame #0 {
        # "显示量程说明"
        n232 = global read "COD内部交互全局.vi" "基本量程实时读取"() -> (w412:enum16{"L", "H", "AUTO"})
        n233 = global read "COD内部交互全局.vi" "通讯状态"() -> (→"通讯状态":bool)
        n234 = global read "CODMn断电保存全局变量.vi" "MB通信方式选择"() -> (w415:enum16{"串口", "TCP"})
        n235 = local read "低量程稀释倍数:"() -> (w427:i8)
        n236 = local read "高量程稀释倍数:"() -> (w418:i8)
        n237 = case shown="\"TCP\"" w415 {
          tunnel: [w432 w433] -> w419
          frame "串口", Default {
            n238 = global read "CODMn断电保存全局变量.vi" "VISA resource name"() -> (w432:refnum<visa-resource-name>)
          }
          frame "TCP" {
            n239 = global read "CODMn断电保存全局变量.vi" "IP"() -> (w433:string)
          }
        }
        "COM" <- w419
        n240 = Multiply(x=w427, y=i8 8) -> (x*y=w410:i8)
        n241 = Multiply(x=w418, y=i8 8) -> (x*y=w411:i8)
        n242 = case shown="\"L\", 默认" w412 {
          tunnel: w411 -> [_ w431]
          tunnel: [w430 w431] -> w409
          tunnel: w410 -> [w430 _]
          frame "L", Default {
          }
          frame "H" {
          }
        }
        n243 = Number To Decimal String(number=w410) -> (decimal integer string=w424:string)  [unwired: 1 in]
        n244 = Number To Decimal String(number=w411) -> (decimal integer string=w422:string)  [unwired: 1 in]
        n245 = global read "CODMn断电保存全局变量.vi" "CODMn仪器参数"() -> (w414:T5)
        n246 = Concatenate Strings("L低量程范围:0~" ("量程解释说明"), w424, "(mg/L)\n\nH高量程范围:" ("量程解释说明"), "0" ("字符串"), "~" ("量程解释说明"), w422, "(mg/L)" ("量程解释说明")) -> (→"量程解释说明":string)
        n247 = Bundle By Name(cluster=w414, "测量量程"=w409) -> (w413:T5)
        n248 = global write "CODMn断电保存全局变量.vi" "CODMn仪器参数"(w413) -> ()
      }
    }
    n249 = flat-sequence {
      frame #0 {
        # "参数赋值（只在读取参数时候改变一次）"
        n250 = global read "COD内部交互全局.vi" "读取浮台参数显示"() -> (w229:bool)
        n251 = global read "COD内部交互全局.vi" "读取浮台参数"() -> (w228:u16[])
        n252 = global read "COD内部交互全局.vi" "读取参数显示"() -> (w230:bool)
        n253 = global read "COD内部交互全局.vi" "读取参数"() -> (w231:u16[])
        n254 = case shown="真" w229 {
          tunnel: w228 -> [_ w237]
          frame False {
          }
          frame True {
            n255 = Index Array(array=w237) -> (element #1=w236:u16, element #2=w235:u16, element #3=w234:u16, element #4=w233:u16)  [unwired: 4 in]
            n256 = global write "COD内部交互全局.vi" "读取浮台参数显示"(FALSE ("读取参数显示")) -> ()
            n257 = local write "采水泵进样时间/s:"(w236) -> ()
            n258 = local write "采水泵润洗时间/s:"(w235) -> ()
            n259 = local write "采水泵沉淀时间/s:"(w234) -> ()
            n260 = local write "采水泵排液时间/s:"(w233) -> ()
          }
        }
        n261 = case shown="真" w230 {
          tunnel: w231 -> [_ w259]
          frame False {
          }
          frame True {
            n262 = Index Array(array=w259) -> (element #1=w268:u16, element #2=w238:u16, element #3=w264:u16, element #4=w242:u16, element #5=w267:u16, element #6=w266:u16, element #7=w278:u16, element #8=w277:u16, element #9=w276:u16, element #10=w275:u16, element #11=w274:u16, element #12=w273:u16, element #13=w272:u16, element #14=w271:u16, element #15=w270:u16, element #16=w262:u16, element #17=w261:u16, element #18=w260:u16, element #19=w257:u16, element #20=w256:u16, element #21=w255:u16, element #22=w254:u16, element #23=w253:u16, element #27=w249:u16, element #28=w248:u16, element #29=w247:u16, element #30=w246:u16, element #31=w245:u16)  [unwired: 31 in, 3 out]
            n263 = global write "COD内部交互全局.vi" "读取参数显示"(FALSE ("读取参数显示")) -> ()
            n264 = local write "水样："(w266) -> ()
            n265 = local write "标液："(w277) -> ()
            n266 = local write "硫酸"(w272) -> ()
            n267 = global read "CODMn断电保存全局变量.vi" "CODMn仪器参数"() -> (w241:T5)
            n268 = local write "零点核查样："(w276) -> ()
            n269 = local write "加标回收样："(w275) -> ()
            n270 = local write "当前量程："(w267) -> ()
            n271 = local write "蒸馏水："(w278) -> ()
            n272 = local write "恒温时间"(w238) -> ()
            n273 = local write "高锰酸钾"(w274) -> ()
            n274 = local write "草酸钠"(w273) -> ()
            n275 = local write "零点泵计量数 2"(w271) -> ()
            n276 = local write "标度泵计量数 2"(w270) -> ()
            n277 = local write "高量程稀释倍数:"(w262) -> ()
            n278 = local write "低量程稀释倍数:"(w261) -> ()
            n279 = local write "CODMn零点核查选择"(w260) -> ()
            n280 = Build Array(w257, w256, w255, w254, w253) -> (w252:u16[])
            n281 = Build Array(w249, w248, w247, w246, w245) -> (w244:u16[])
            n282 = Divide(x=w268, y=u16 10) -> (x/y=w239:dbl)
            n283 = Divide(x=w264, y=u16 100) -> (x/y=w263:dbl)
            n284 = local write "氢氧化钠："(w242) -> ()
            n285 = local write "温度"(w239) -> ()
            n286 = local write "标准液浓度"(w263) -> ()
            n287 = call "HexToString.vi"("数组"=w244) -> ("字符串"=w243:string)  [unwired: 10 in]
            "CODMn序列号" <- w243
            "序列号" <- w243
            n288 = call "FATEK_HexToString.vi"("数组"=w252) -> ("STRING"=w251:string[])  [unwired: 10 in]
            n289 = Bundle By Name(cluster=w241, "消解温度"=w239, "消解时长"=w238) -> (w240:T5)
            n290 = Index Array(array=w251) -> (element=→"CODMn软件版本：":string)  [unwired: 1 in]
            n291 = global write "CODMn断电保存全局变量.vi" "CODMn仪器参数"(w240) -> ()
            n292 = global write "COD内部交互全局.vi" "序列号:"(w243) -> ()
          }
        }
      }
    }
    n293 = flat-sequence {
      frame #0 {
        # "权限隐藏和显示功能"
        n294 = global read "CODMN外部API.vi" "权限等级"() -> (w437:enum16{"一级权限", "二级权限", "三级权限", "超级权限"})
        n295 = global read "CODMn断电保存全局变量.vi" "CODMn系统周期测试?"() -> (w440:bool)
        n296 = global read "CODMn断电保存全局变量.vi" "运行周期"() -> (w441:T4)
        n297 = case shown="\"二级权限\"" w437 {
          tunnel: [w460 FALSE w465 w467] -> w434
          tunnel: ["一级权限" "二级权限" "三级权限" "超级权限"] -> w436
          tunnel: [w460 TRUE w465 w467] -> w435
          frame "一级权限", Default {
            w460 = FALSE
          }
          frame "二级权限" {
          }
          frame "三级权限" {
            w465 = TRUE
          }
          frame "超级权限" {
            w467 = TRUE
          }
        }
        "权限等级" <- w436
        n298 = property on="更新程序" class="Bool (严格)"("Visible"=w434) -> ()  [unwired: 2 in, 2 out]
        n299 = property on="释放串口" class="Bool"("Visible"=w435) -> ()  [unwired: 2 in, 2 out]
        n300 = property on="打开串口" class="Bool"("Visible"=w435) -> ()  [unwired: 2 in, 2 out]
        n301 = property on="屏蔽负值" class="Bool (严格)"("Visible"=w434) -> ()  [unwired: 2 in, 2 out]
        n302 = case shown="假" w440 {
          tunnel: w441 -> [_ w472]
          tunnel: [T9."Enabled" ("禁用") w470] -> w439
          frame False {
          }
          frame True {
            n303 = Unbundle By Name(w472) -> ("运行模式"=w471:enum16{"维护模式", "常规模式", "应急模式", "质控模式"})
            n304 = case shown="\"维护模式\", 默认" w471 {
              tunnel: [T9."Enabled" ("禁用") T9."Disabled and Grayed Out" ("禁用") T9."Disabled and Grayed Out" ("禁用") T9."Disabled and Grayed Out" ("禁用")] -> w470
              frame "维护模式", Default {
              }
              frame "常规模式" {
              }
              frame "应急模式" {
              }
              frame "质控模式" {
              }
            }
          }
        }
        n305 = property on="序列号变更" class="Bool"("Visible"=w434) -> ()  [unwired: 2 in, 2 out]
        n306 = property on="常规版/认证版" class="Enum (严格)"("Visible"=w434) -> ()  [unwired: 2 in, 2 out]
        n307 = property on="CODMn零点核查选择" class="Enum (严格)"("Visible"=w434) -> ()  [unwired: 2 in, 2 out]
        n308 = property on="低量程稀释倍数:" class="DigNum (严格)"("Visible"=w434) -> ()  [unwired: 2 in, 2 out]
        n309 = property on="稀释倍数解释" class="Str"("Visible"=w434) -> ()  [unwired: 2 in, 2 out]
        n310 = property on="高量程稀释倍数:" class="DigNum (严格)"("Visible"=w434) -> ()  [unwired: 2 in, 2 out]
        n311 = control-ref of="水样："() -> (w452:refnum<vi>)
        n312 = control-ref of="蒸馏水："() -> (w451:refnum<vi>)
        n313 = control-ref of="标液："() -> (w450:refnum<vi>)
        n314 = control-ref of="零点核查样："() -> (w449:refnum<vi>)
        n315 = control-ref of="加标回收样："() -> (w448:refnum<vi>)
        n316 = local read "水样量程选择:"() -> (w456:enum16{"L", "H", "自动切换测一次", "自动切换测两次"})
        n317 = control-ref of="量程解释说明"() -> (w446:refnum<vi>)
        n318 = control-ref of="氢氧化钠："() -> (w447:refnum<vi>)
        n319 = property on="定时设置" class="定时设置 (严格)"("DisabledEnum"=w439) -> ()  [unwired: 2 in, 2 out]
        n320 = local read "常规版/认证版"() -> (w454:enum16{"常规版-酸性", "常规版-碱性", "认证版", "浮台版"})
        n321 = Not Equal To 0?(x=w456) -> (x != 0?=w455:bool)
        n322 = control-ref of="进样管"() -> (w444:refnum<vi>)
        n323 = case shown="\"认证版\"" w454 {
          tunnel: [T9."Enabled" ("禁用") T9."Enabled" ("禁用") T9."Disabled and Grayed Out" ("禁用") T9."Enabled" ("禁用")] -> _
          tunnel: [i32[] [2] ("禁用项[]") i32[] [2] ("禁用项[]") i32[] [] ("禁用项[]") i32[] [2] ("禁用项[]")] -> _
          tunnel: [w480 w485 T9."Disabled and Grayed Out" ("禁用") w496] -> _
          tunnel: [w479 FALSE FALSE TRUE] -> w453
          tunnel: [w480 w485 T9."Disabled and Grayed Out" ("禁用") w496] -> w443
          tunnel: [w479 TRUE FALSE FALSE] -> w442
          frame "常规版-酸性", Default {
            w479 = FALSE
            w480 = T9."Enabled" ("禁用")
          }
          frame "常规版-碱性" {
            w485 = T9."Enabled" ("禁用")
          }
          frame "认证版" {
            w491 = u16 1 items=["水样测试"=1, "标样核查"=2, "零点核查"=3, "跨度核查"=4, "空白测试"=5, "平行样"=6, "加标回收"=7] ("测量模式(公式)")
            n324 = global write "CODMn断电保存全局变量.vi" "测量模式(公式)"(w491) -> ()
          }
          frame "浮台版" {
            w496 = T9."Enabled" ("禁用")
          }
        }
        n325 = Build Array(w452, w451, w450, w449, w448, w446, w447, w444) -> (w445:refnum<vi>[])
        n326 = Select(t=T9."Enabled" ("禁用"), s=w455, f=T9."Disabled and Grayed Out" ("禁用")) -> (s? t:f=w457:T9)
        n327 = for {
          tunnel: w445 -> [w478] mode=indexing
          tunnel: w443 -> [w477]
          n328 = property class="Ctl"(reference=w478, "DisabledEnum"=w477) -> ()  [unwired: 1 in, 2 out]
        }
        n329 = property on="低切高阈值:" class="DigNum (严格)"("DisabledEnum"=w457) -> ()  [unwired: 2 in, 2 out]
        n330 = property on="高切低阈值:" class="DigNum (严格)"("DisabledEnum"=w457) -> ()  [unwired: 2 in, 2 out]
        n331 = property on="采水泵润洗时间/s:" class="DigNum (严格)"("Visible"=w453) -> ()  [unwired: 2 in, 2 out]
        n332 = property on="采水泵沉淀时间/s:" class="DigNum (严格)"("Visible"=w453) -> ()  [unwired: 2 in, 2 out]
        n333 = property on="采水泵排液时间/s:" class="DigNum (严格)"("Visible"=w453) -> ()  [unwired: 2 in, 2 out]
        n334 = property on="采水泵进样时间/s:" class="DigNum (严格)"("Visible"=w453) -> ()  [unwired: 2 in, 2 out]
        n335 = property on="氢氧化钠：" class="DigNum (严格)"("Visible"=w442) -> ()  [unwired: 2 in, 2 out]
        n336 = property on="氢氧化钠" class="DigNum (严格)"("Visible"=w442) -> ()  [unwired: 2 in, 2 out]
        n337 = property on="公式切换阈值滴定数(0-9999)" class="DigNum (严格)"("Visible"=TRUE) -> ()  [unwired: 2 in, 2 out]
      }
    }
    n338 = flat-sequence {
      frame #0 {
        # "公式读取显示（只在读取公式的时候改变一次）"
        n339 = global read "COD内部交互全局.vi" "读取公式显示"() -> (w279:bool)
        n340 = case shown="真" w279 {
          frame False {
          }
          frame True {
            n341 = global write "COD内部交互全局.vi" "读取公式显示"(FALSE ("读取参数显示")) -> ()
            n342 = global read "COD内部交互全局.vi" "读取公式"() -> (w300:u16[])
            n343 = Array Subset(array=w300, index=10 ("索引"), length=84 ("长度")) -> (w288:u16[])
            n344 = Index Array(array=w288, index #1=24 ("索引")) -> (element #1=w286:u16, element #2=w285:u16)  [unwired: 1 in]
            n345 = call "浮点CDAB转换COD.vi"("数组"=w288) -> ("数组 2"=w297:sgl[])  [unwired: 10 in]
            n346 = Array To Cluster(array=w297) -> (cluster=w299:T12)
            n347 = local read "量程选择"() -> (w290:enum16{"低量程", "高量程"})
            n348 = case shown="\"低量程\", 默认" w290 {
              tunnel: w299 -> [w308 w316]
              tunnel: [w307 w315] -> w293
              tunnel: [w306 w314] -> w292
              tunnel: [w305 w313] -> w291
              tunnel: w286 -> [w304 _]
              tunnel: w285 -> [_ w312]
              tunnel: [w303 w311] -> w282
              tunnel: [w302 w309] -> w281
              tunnel: [w301 w310] -> w280
              frame "低量程", Default {
                n349 = local write "公式切换阈值滴定数(0-9999)"(w304) -> ()
                n350 = Unbundle By Name(w308) -> ("数组 2[0]"=w307:sgl, "数组 2[1]"=w306:sgl, "数组 2[2]"=w305:sgl, "数组 2[3]"=w303:sgl, "数组 2[4]"=w302:sgl, "数组 2[5]"=w301:sgl)
              }
              frame "高量程" {
                n351 = local write "公式切换阈值滴定数(0-9999)"(w312) -> ()
                n352 = Unbundle By Name(w316) -> ("数组 2[6]"=w315:sgl, "数组 2[7]"=w314:sgl, "数组 2[8]"=w313:sgl, "数组 2[9]"=w311:sgl, "数组 2[10]"=w309:sgl, "数组 2[11]"=w310:sgl)
              }
            }
            n353 = Bundle By Name(cluster=cluster{"X":dbl, "b":dbl, "X^2":dbl} {"X"=0.0, "b"=0.0, "X^2"=0.0} ("方程系数"), "X"=w293, "b"=w292, "X^2"=w291) -> (w298:cluster{"X":dbl, "b":dbl, "X^2":dbl})
            n354 = Bundle By Name(cluster=cluster{"X":dbl, "b":dbl, "X^2":dbl} {"X"=0.0, "b"=0.0, "X^2"=0.0} ("方程系数"), "X"=w282, "b"=w281, "X^2"=w280) -> (w283:cluster{"X":dbl, "b":dbl, "X^2":dbl})
            n355 = local write "方程系数 2"(w283) -> ()
            n356 = local write "方程系数"(w298) -> ()
          }
        }
      }
    }
    n357 = Wait (ms)(milliseconds to wait=u32 1000 ("等待时间（毫秒）")) -> ()  [unwired: 1 out]
  }
  n358 = while {
    stop <- FALSE stop-if-true
    w534 = T13 0 items=["最小二乘", "最小绝对残差", "Bisquare"] ("method")
    # "计算线性、多项式公式、远程校准"
    n359 = local read "浓度1"() -> (w516:dbl)
    n360 = local read "浓度2"() -> (w535:dbl)
    n361 = local read "浓度3"() -> (w536:dbl)
    n362 = local read "浓度4"() -> (w530:dbl)
    n363 = local read "浓度5"() -> (w529:dbl)
    n364 = Build Array("泵滴定数1", "泵滴定数2", "泵滴定数3", "泵滴定数4", "泵滴定数5") -> (w501:dbl[])
    n365 = Build Array(w516, w535, w536, w530, w529) -> (w500:dbl[])
    n366 = Build Array("启用1", "启用2", "启用3", "启用4", "启用5") -> (w502:bool[])
    n367 = call "将启用的浓度作为新的浓度数组.vi"("启用布尔数组"=w502, "输入浓度数组"=w500) -> ("启用的浓度数组"=w515:dbl[])  [unwired: 13 in]
    n368 = global read "CODMN外部API.vi" "远程反控校准CODMn"() -> (w514:bool)
    n369 = call "CODMn线性公式.vi"("标液浓度"=w500, "滴定数"=w501, "启用"=w502, "method"=w534, "模型"="模型", "精度"=6) -> ("Polynomial Coefficients 2"=w505:dbl[], "拟合方程"=w522:string, "r^2"=w504:dbl, "拟合方程 2"=w510:string, "r^2 2"=→"r^2 2":dbl, "XY图"=→"XY图":cluster{"X Values":dbl[], "Y Values":dbl[]}[], "Polynomial Coefficients"=w531:dbl[])  [unwired: 7 in]
    "拟合公式" <- w522
    "r^2" <- w504
    "拟合公式 2" <- w510
    n370 = global write "COD内部交互全局.vi" "启用的浓度数组"(w515) -> ()
    n371 = feedback #4(w510) -> (w511:string)
    n372 = feedback-in #4(w510) -> ()
    n373 = feedback #5(w522) -> (w523:string)
    n374 = feedback-in #5(w522) -> ()
    n375 = Not Equal?(x=w510, y=w511) -> (x != y?=w508:bool)
    n376 = call <vilib>:"Boolean Crossing PtByPt.vi"("direction"=enum16{"either", "false-true", "true-false"}."false-true", "input"=w514) -> ("crossing"=w513:bool)  [unwired: 1 in]
    n377 = Not Equal?(x=w522, y=w523) -> (x != y?=w509:bool)
    n378 = Or(x=w509, y=w508) -> (x .or. y?=w507:bool)
    n379 = case shown="真" w507 {
      tunnel: w531 -> [_ w556]
      tunnel: w505 -> [_ w552]
      tunnel: w504 -> [_ w548]
      tunnel: "模型" -> [_ w546]
      tunnel: w502 -> [_ w545]
      tunnel: w501 -> [_ w544]
      tunnel: w500 -> [_ w543]
      frame False {
      }
      frame True {
        # "当公式发生改变时赋值到右侧公式"
        n380 = case shown="\"折线\"" w546 {
          tunnel: [9999.0 ("泵滴定数5") 9999.0 ("泵滴定数5") w561] -> w547
          tunnel: w544 -> [_ _ w567]
          tunnel: w545 -> [_ _ w568]
          tunnel: w543 -> [_ _ w566]
          frame "线性", Default {
          }
          frame "多项式" {
          }
          frame "折线" {
            n381 = call "监测浓度升序排列 (子VI).vi"("标液浓度"=w566, "滴定数"=w567, "启用"=w568) -> ("输出数组"=w562:dbl[][])  [unwired: 8 in]
            n382 = Index Array(array=w562, index (col)=0 ("禁用的索引 (列)")) -> (element=w564:dbl[])  [unwired: 1 in]
            n383 = Index Array(array=w564, index=1 ("索引")) -> (element=w561:dbl)
          }
        }
        n384 = Rotate 1D Array(1:w556, 2:-1 ("n")) -> (0:w557:dbl[])
        n385 = Rotate 1D Array(1:w552, 2:-1 ("n")) -> (0:w554:dbl[])
        n386 = global read "CODMn断电保存全局变量.vi" "CODMn仪器参数"() -> (w550:T5)
        n387 = Array To Cluster(array=w557) -> (cluster=w555:cluster{"[0]":dbl, "[1]":dbl, "[2]":dbl})
        n388 = Array To Cluster(array=w554) -> (cluster=w551:cluster{"[0]":dbl, "[1]":dbl, "[2]":dbl})
        n389 = Bundle By Name(cluster=w550, "线性相关系数"=w548) -> (w549:T5)
        n390 = global write "CODMn断电保存全局变量.vi" "CODMn仪器参数"(w549) -> ()
        n391 = local write "公式切换阈值滴定数(0-9999)"(w547) -> ()
        n392 = local write "方程系数"(w555) -> ()
        n393 = local write "方程系数 2"(w551) -> ()
      }
    }
    n394 = case shown="真" w513 {
      tunnel: w500 -> [_ _]
      frame False {
      }
      frame True {
        n395 = global read "CODMn断电保存全局变量.vi" "远程标样校准"() -> (w541:enum16{"标液1", "标液2", "标液3", "标液4"})
        n396 = local read "远程校准量程"() -> (w539:enum16{"低量程", "高量程"})
        n397 = Increment(x=w541) -> (x+1=w540:enum16{"标液1", "标液2", "标液3", "标液4"})
        n398 = property on="量程选择" class="Enum (严格)"("Val(Sgnl)"=w539) -> ()  [unwired: 2 in, 2 out]
        n399 = Increment(x=w540) -> (x+1=w542:enum16{"标液1", "标液2", "标液3", "标液4"})
        n400 = global write "COD内部交互全局.vi" "当前校准"(w542) -> ()
      }
    }
    n401 = Wait (ms)(milliseconds to wait=u32 1000 ("等待时间（毫秒）")) -> ()  [unwired: 1 out]
  }
  n402 = while {
    tunnel: w17 -> [w578]
    tunnel: w16 -> [w577]
    tunnel: w7 -> [_]
    stop <- FALSE stop-if-true
    # "主循环界面显示"
    n403 = flat-sequence {
      frame #0 {
        # "A，B，K"
        # "CODMn读取状态"
        n404 = global read "CODMn断电保存全局变量.vi" "屏蔽负值"() -> (w715:bool)
        n405 = global read "COD内部交互全局.vi" "ORP、时间"() -> (w717:u16[])
        n406 = To Word Integer(number=w717) -> (16bit integer=w735:i16[])
        n407 = Split 1D Array(array=w735, index=3 ("索引")) -> (first subarray=w719:i16[], second subarray=w734:i16[])
        n408 = Index Array(array=w719) -> (element #1=w723:i16, element #2=w722:i16, element #3=w721:i16)  [unwired: 3 in]
        n409 = Index Array(array=w734) -> (element #1=w714:i16, element #2=w733:i16, element #3=w732:i16, element #4=w731:i16)  [unwired: 4 in]
        n410 = case shown="真" w715 {
          selector: w715 -> [w737 _]
          tunnel: w714 -> [w739 w744]
          tunnel: [w738 w747] -> w713
          tunnel: [w737 w743] -> _
          frame False {
            n411 = To Single Precision Float(number=w739) -> (single precision float=w741:sgl)
            n412 = Divide(x=w741, y=sgl 100.0) -> (x/y=w738:sgl)
          }
          frame True {
            n413 = To Single Precision Float(number=w744) -> (single precision float=w745:sgl)
            n414 = Divide(x=w745, y=sgl 100.0) -> (x/y=w742:sgl)
            n415 = Less Or Equal To 0?(x=w742) -> (x <= 0?=w743:bool)
            n416 = case shown="真" w743 {
              tunnel: [w748 sgl 0.015] -> w747
              tunnel: w742 -> [w748 _]
              frame False {
              }
              frame True {
              }
            }
          }
        }
        "COD浓度（mg/L)" <- w713
        n417 = To Single Precision Float(number=w731) -> (single precision float=w725:sgl)
        n418 = Build Array(w723, w722, w721) -> (w720:i16[])
        n419 = To Single Precision Float(number=w733) -> (single precision float=w730:sgl)
        n420 = To Single Precision Float(number=w732) -> (single precision float=w726:sgl)
        n421 = call "HexToDate.vi"("数组"=w720) -> ("DATE"=w724:timestamp[])  [unwired: 10 in]
        n422 = Number To Decimal String(number=w730) -> (decimal integer string=→"ORP-A":string)  [unwired: 1 in]
        n423 = Number To Decimal String(number=w726) -> (decimal integer string=→"ORP-B":string)  [unwired: 1 in]
        n424 = Number To Decimal String(number=w725) -> (decimal integer string=→"ORP-K":string)  [unwired: 1 in]
        n425 = Index Array(array=w724) -> (element=w718:timestamp)  [unwired: 1 in]
        n426 = Format Date/Time String(seconds (now)=w718) -> (date/time string=→"数据时间":string)  [unwired: 2 in]
      }
    }
    n427 = flat-sequence {
      frame #0 {
        # "测量状态显示"
        n428 = global read "COD内部交互全局.vi" "测量状态"() -> (w629:u16[])
        n429 = To Word Integer(number=w629) -> (16bit integer=w639:i16[])
        n430 = Index Array(array=w639, index #1=0 ("索引"), index #4=3 ("索引"), index #14=13 ("索引"), index #15=14 ("索引"), index #21=20 ("索引"), index #32=31 ("索引")) -> (element #1=w643:i16, element #2=w642:i16, element #3=w641:i16, element #4=w625:i16, element #5=→"模式（受控）":i16, element #6=→"进样管":i16, element #7=→"高锰酸钾":i16, element #8=→"草酸钠":i16, element #9=→"硫酸":i16, element #10=w638:i16, element #11=w658:i16, element #12=w634:i16, element #13=→"报警数字":i16, element #14=w664:i16, element #15=w649:i16, element #16=→"多列列表框":i16, element #20=→"氢氧化钠":i16, element #21=w622:i16, element #33=→"分":i16, element #34=→"秒":i16)  [unwired: 28 in, 14 out]
        "CODMn工作状态" <- w625
        n431 = global write "COD内部交互全局.vi" "基本量程实时读取"(w622) -> ()
        n432 = Build Array(w643, w642, w641) -> (w644:i16[])
        n433 = To Single Precision Float(number=w638) -> (single precision float=→"实时ORP":sgl)
        n434 = Number To Decimal String(number=w622) -> (decimal integer string=→"基本量程(显示)":string)  [unwired: 1 in]
        n435 = Equal?(x=w634, y=u16 1) -> (x = y?=→"排液标记":bool)
        n436 = Equal?(x=w634, y=u16 2) -> (x = y?=→"断电排液标记":bool)
        n437 = Divide(x=w658, y=u16 10) -> (x/y=→"消解温度℃":dbl)
        n438 = Divide(x=w664, y=u16 1000) -> (x/y=→"零点滴定值":dbl)
        n439 = Divide(x=w649, y=u16 1000) -> (x/y=→"标度滴定值":dbl)
        n440 = Equal?(x=w625, y=T3."水样测试" ("CODMn工作状态")) -> (x = y?=w623:bool)
        n441 = call "HexToDate.vi"("数组"=w644) -> ("DATE"=w640:timestamp[])  [unwired: 10 in]
        n442 = case shown="真" w623 {
          tunnel: w622 -> [_ w667]
          frame False {
          }
          frame True {
            n443 = global write "CODMn断电保存全局变量.vi" "水样测试量程"(w667) -> ()
          }
        }
        n444 = Index Array(array=w640) -> (element=→"仪器时间":timestamp)  [unwired: 1 in]
      }
    }
    n445 = flat-sequence {
      frame #0 {
        # "报警状态显示"
        n446 = global read "COD内部交互全局.vi" "报警点位"() -> (w682:bool[])
        n447 = Index Array(array=w682, index #1=0 ("索引")) -> (element #1=w679:bool, element #2=w678:bool, element #3=w677:bool, element #4=w676:bool, element #5=w675:bool, element #6=w674:bool, element #7=w673:bool, element #8=w672:bool, element #9=w671:bool, element #11=w670:bool, element #13=w669:bool, element #14=w668:bool)  [unwired: 13 in, 2 out]
        "ORP故障" <- w679
        "温控器故障" <- w678
        "加热故障" <- w671
        "高锰酸钾报警" <- w673
        "草酸钠报警" <- w672
        "测量错误" <- w677
        "校零错误" <- w676
        "校标错误" <- w675
        "进水样超量程" <- w674
        "排液故障" <- w670
        "60分钟超时报警" <- w669
        "进样无液体告警" <- w668
        n448 = Compound Arithmetic op=OR ("复合运算")(w679, w678, w671, w673, w672, w677, w675, w676, w674, w670, w669) -> (→"故障标记":bool)
        n449 = Bundle By Name(cluster=T14 {"ORP故障"=FALSE, "温控器故障"=FALSE, "加热故障"=FALSE, "高锰酸钾报警"=FALSE, "草酸钠报警"=FALSE, "测量错误"=FALSE, "校零错误"=FALSE, "校标错误"=FALSE, " 进水样超量程"=FALSE, "排液阀故障"=FALSE, "60分钟超时报警"=FALSE, "进样无液体报警"=FALSE} ("报警簇"), "ORP故障"=w679, "温控器故障"=w678, "加热故障"=w671, "高锰酸钾报警"=w673, "草酸钠报警"=w672, "测量错误"=w677, "校零错误"=w676, "校标错误"=w675, "进水样超量程"=w674, "排液阀故障"=w670, "60分钟超时报警"=w669, "进样无液体报警"=w668) -> (w680:T14)
        n450 = global write "COD内部交互全局.vi" "报警簇"(w680) -> ()
      }
    }
    n451 = flat-sequence {
      frame #0 {
        # "CODMn读取状态"
        n452 = global read "COD内部交互全局.vi" "温度"() -> (w712:bool[])
        n453 = global read "COD内部交互全局.vi" "M输出点"() -> (w711:bool[])
        n454 = Index Array(array=w712) -> (element=→"加热":bool)  [unwired: 1 in]
        n455 = Index Array(array=w711) -> (element #1=→"搅拌":bool, element #4=→"进水样":bool, element #5=→"进蒸馏水":bool, element #6=→"进标液":bool, element #7=→"进零点核查样":bool, element #8=→"进加标回收样":bool, element #9=→"进高锰酸钾":bool, element #10=→"进草酸钠":bool, element #11=→"进硫酸":bool)  [unwired: 11 in, 2 out]
      }
    }
    n456 = flat-sequence {
      frame #0 {
        # "工作状态显示"
        n457 = local read "CODMn工作状态"() -> (w588:T3)
        n458 = Not Equal To 0?(x=w588) -> (x != 0?=w587:bool)
        n459 = Equal?(x=w588, y=u16 8) -> (x = y?=→"校零标记":bool)
        n460 = Equal?(x=w588, y=u16 4) -> (x = y?=→"跨度核查标记":bool)
        n461 = Equal?(x=w588, y=u16 0) -> (x = y?=→"待机":bool)
        n462 = Equal?(x=w588, y=u16 3) -> (x = y?=→"零点核查标记":bool)
        n463 = Equal?(x=w588, y=u16 7) -> (x = y?=→"质控样测量":bool)
        n464 = Equal?(x=w588, y=u16 1) -> (x = y?=→"水样测量":bool)
        n465 = Equal?(x=w588, y=u16 2) -> (x = y?=→"标样核查标记":bool)
        n466 = Equal?(x=w588, y=u16 6) -> (x = y?=→"平行样测量":bool)
        n467 = Equal?(x=w588, y=u16 9) -> (x = y?=→"校标标记":bool)
        n468 = Equal?(x=w588, y=u16 5) -> (x = y?=→"空白测试标记":bool)
        n469 = Equal?(x=w588, y=u16 10) -> (x = y?=→"加标回收测量":bool)
        n470 = case shown="真" w587 {
          tunnel: w588 -> [_ w612]
          frame False {
          }
          frame True {
            n471 = case shown="\"水样测试\"" w612 {
              tunnel: [_ u16 0 ("y") u16 1 ("y") u16 2 ("y") u16 3 ("y") u16 4 ("y") u16 6 ("y") _ u16 7 ("y") u16 8 ("y") u16 5 ("y")] -> w611
              frame "空闲", Default {
              }
              frame "水样测试" {
              }
              frame "标样核查" {
              }
              frame "零点核查" {
              }
              frame "跨度核查" {
              }
              frame "空白测试" {
              }
              frame "平行样测试" {
              }
              frame "质控样" {
              }
              frame "空白校准" {
              }
              frame "标样校准" {
              }
              frame "加标回收" {
              }
            }
            n472 = global write "COD内部交互全局.vi" "测量模式数字"(w611) -> ()
          }
        }
      }
    }
    n473 = Get Date/Time In Seconds() -> (seconds since 1Jan1904=→"系统时间":timestamp)
    n474 = First Call?() -> (First Call?: T/F=w576:bool)
    n475 = Wait (ms)(milliseconds to wait=u32 1000 ("等待时间（毫秒）")) -> ()  [unwired: 1 out]
    n476 = case shown="真" w576 {
      tunnel: w578 -> [w686 w697]
      tunnel: w577 -> [w685 w696]
      tunnel: [w686 w688] -> w574
      tunnel: [w685 w687] -> w573
      frame False {
      }
      frame True {
        n477 = Bundle By Name(cluster=cluster{"命令":string} {"命令"=""} ("元素"), "命令"="CODMn读取参数" ("名称（未命名）")) -> (w700:cluster{"命令":string})
        n478 = Enqueue Element(queue=w697, element=w700, timeout in ms (-1)=1000 ("超时毫秒(-1)"), error in (no error)=w696) -> (queue out=w690:refnum<queue>, error out=w689:errorcluster)  [unwired: 1 out]
        n479 = Bundle By Name(cluster=cluster{"命令":string} {"命令"=""} ("元素"), "命令"="CODMn读取公式" ("名称（未命名）")) -> (w691:cluster{"命令":string})
        n480 = Enqueue Element(queue=w690, element=w691, timeout in ms (-1)=1000 ("超时毫秒(-1)"), error in (no error)=w689) -> (queue out=w688:refnum<queue>, error out=w687:errorcluster)  [unwired: 1 out]
      }
    }
    n481 = Get Queue Status(queue=w574, error in (no error)=w573) -> (queue out=w570:refnum<queue>, error out=w569:errorcluster, # elements in queue=w572:i32)  [unwired: 1 in, 5 out]
    n482 = Equal To 0?(x=w572) -> (x = 0?=w571:bool)
    n483 = case shown="真" w571 {
      tunnel: w570 -> [_ w582]
      tunnel: w569 -> [_ w581]
      frame False {
      }
      frame True {
        n484 = Bundle By Name(cluster=cluster{"命令":string} {"命令"=""} ("元素"), "命令"="CODMn读取" ("名称（未命名）")) -> (w584:cluster{"命令":string})
        n485 = Enqueue Element(queue=w582, element=w584, timeout in ms (-1)=1000 ("超时毫秒(-1)"), error in (no error)=w581) -> ()  [unwired: 3 out]
      }
    }
  }
  n486 = while {
    tunnel: w17 -> [w751]
    tunnel: w16 -> [w750]
    stop <- FALSE stop-if-true
    # "主线事件"
    n487 = event shown="[21] \"浓度1\", \"浓度2\", \"浓度3\", \"泵滴定数1\", \"泵滴定数2\", \"泵滴定数3\", \"启用1\", \"启用2\", \"启用3\", \"浓度4\", \"浓度5\", \"泵滴定数4\", \"泵滴定数5\", \"启用4\", \"启用5\", \"标液校准时间1\", \"标液校准时间2\", \"标液校准时间3\", \"标液校准时间4\", \"零点校准时间\": 值改变" {
      selector: _ -> [_ _ _ _ _ _ _ _ _ _ _ _ _ _ _ _ _ _ _ _ _ _ _ _ _ _ _ _ _ _ _]
      dyn-events: _ -> [_ _ _ _ _ _ _ _ _ _ _ _ _ _ _ _ _ _ _ _ _ _ _ _ _ _ _ _ _ _ _]
      timeout: _ -> [_ _ _ _ _ _ _ _ _ _ _ _ _ _ _ _ _ _ _ _ _ _ _ _ _ _ _ _ _ _ _]
      tunnel: w751 -> [_ _ _ _ w829 _ _ _ w892 w1030 w1156 _ _ _ _ _ _ _ w1377 _ _ _ w1640 _ _ _ w1696 w1703 w1725 w1768 _]
      tunnel: w750 -> [_ _ _ _ w828 _ _ _ w891 w1029 w1155 _ _ _ _ _ _ _ w1374 _ _ _ w1639 _ _ _ w1695 w1702 w1724 w1767 _]
      event "单步启动": Value Change {
        n488 = event-data() -> ()  [unwired: 1 in, 6 out]
        n489 = call "CODMn手动控制框.vi"() -> ()  [unwired: 12 in]
      }
      event "启动": Mouse Down {
        n490 = event-data() -> ()  [unwired: 1 in, 8 out]
        n491 = global read "COD内部交互全局.vi" "基本量程实时读取"() -> (w755:enum16{"L", "H", "AUTO"})
        n492 = call "启动测量模式选择对话框.vi"("量程选择"=w755) -> ("标样浓度输出"=w753:dbl, "量程选择输出"=w754:enum16{"L", "H", "AUTO"}, "启动选择输出"=w759:u16)  [unwired: 8 in]
        n493 = Not Equal?(x=w759, y=u16 8) -> (x != y?=w756:bool)
        n494 = Not Equal?(x=w759, y=u16 7) -> (x != y?=w757:bool)
        n495 = And(x=w757, y=w756) -> (x .and. y?=w761:bool)
        n496 = case shown="真" w761 {
          tunnel: w759 -> [_ w776]
          tunnel: w754 -> [_ w767]
          tunnel: w753 -> [_ w766]
          frame False {
            n497 = One Button Dialog(message="请到校准配置里面进行校准操作！" ("消息")) -> ()  [unwired: 1 in, 1 out]
          }
          frame True {
            n498 = Not Equal?(x=w776, y=u16 9) -> (x != y?=w771:bool)
            n499 = case shown="\"H\"" w767 {
              tunnel: [w777 w781 errorcluster {"status"=FALSE, "code"=0, "source"=""} ("error out")] -> w765
              frame "L", Default {
                n500 = call "CODMnMB_api.vi"("STEP"=enum16{"open", "read", "write", "close"}."write", "values"=u16[] [0], "starting address"=u16 4276) -> ("error out"=w777:errorcluster)  [unwired: 6 in, 2 out]
              }
              frame "H" {
                n501 = call "CODMnMB_api.vi"("STEP"=enum16{"open", "read", "write", "close"}."write", "values"=u16[] [1], "starting address"=u16 4276) -> ("error out"=w781:errorcluster)  [unwired: 6 in, 2 out]
              }
              frame "AUTO" {
              }
            }
            n502 = global write "CODMN外部API.vi" "手动启动CODMn"(w771) -> ()
            n503 = call "单步测试一键复位.vi"("Error in"=w765) -> ("error out"=w764:errorcluster)  [unwired: 10 in]
            n504 = call <vilib>:"Clear Errors.vi"("error in (no error)"=w764) -> ("error out"=w763:errorcluster)  [unwired: 5 in, 1 out]
            n505 = case shown="0" w776 {
              tunnel: [u16 4608 ("address") u16 4608 ("address") u16 4608 ("address") u16 4608 ("address") u16 4608 ("address") u16 4608 ("address") u16 4608 ("address") u16 4608 ("address") u16 4608 ("address") u16 4608 ("address")] -> w769
              tunnel: [u16 1 ("address") u16 2 ("address") u16 3 ("address") u16 4 ("address") u16 5 ("address") u16 7 ("address") u16 6 ("address") u16 8 ("address") u16 9 ("address") u16 0 ("address")] -> w773
              tunnel: w766 -> [_ w789 _ _ _ _ _ _ _ _]
              frame 0 {
              }
              frame 1 {
                n506 = property on="标样浓度" class="DigNum (严格)"("Val(Sgnl)"=w789) -> ()  [unwired: 2 in, 2 out]
              }
              frame 2 {
              }
              frame 3 {
              }
              frame 4 {
              }
              frame 5 {
              }
              frame 6 {
              }
              frame 7 {
              }
              frame 8 {
              }
              frame 9, Default {
              }
            }
            n507 = Insert Into Array(array=u16[] [] ("values"), index=0 ("索引"), new element=w773) -> (w768:u16[])
            n508 = call "CODMnMB_api.vi"("STEP"=enum16{"open", "read", "write", "close"}."write", "Error in"=w763, "values"=w768, "starting address"=w769) -> ()  [unwired: 5 in, 3 out]
          }
        }
      }
      event "停止": Value Change {
        n509 = event-data() -> ()  [unwired: 1 in, 6 out]
        n510 = Two Button Dialog(message="确认是否停止？" ("消息"), 1:"否" ("F按钮名称（“取消”）"), 2:"是" ("T按钮名称（“确定”）")) -> (T button?=w809:bool)
        n511 = case shown="真" w809 {
          frame False {
          }
          frame True {
            n512 = Obtain Notifier(name (unnamed)="CODMn" ("名称（未命名）"), notification data type=FALSE) -> (notifier out=w815:refnum<notifier>, error out=w813:errorcluster)  [unwired: 2 in, 1 out]
            n513 = Send Notification(notification=TRUE ("通知"), notifier=w815, error in (no error)=w813) -> (notifier out=w812:refnum<notifier>, error out=w811:errorcluster)
            n514 = Release Notifier(notifier=w812, error in (no error)=w811) -> ()  [unwired: 1 in, 3 out]
            n515 = call "CODMnMB_api.vi"("STEP"=enum16{"open", "read", "write", "close"}."write", "values"=u16[] [11], "starting address"=u16 4608) -> ()  [unwired: 6 in, 3 out]
          }
        }
      }
      event "手动控制": Value Change {
        n516 = event-data() -> ()  [unwired: 1 in, 6 out]
        n517 = call "数字密码键盘.vi"() -> ("NewNumber"=w821:u32)  [unwired: 1 in]
        n518 = Equal?(x=w821, y=8.0) -> (x = y?=w822:bool)
        n519 = case shown="假" w822 {
          frame False {
            n520 = call "窗口弹出对话框(子VI).vi"("消息"="密码错误") -> ()  [unwired: 10 in, 1 out]
          }
          frame True {
          }
        }
      }
      event "参数配置": Value Change {
        (unwired) u16 20 ("number of holding registers")
        (unwired) u16 4272 ("starting address")
        n521 = event-data() -> ()  [unwired: 1 in, 6 out]
        n522 = global read "CODMN外部API.vi" "ping"() -> (w827:bool)
        n523 = property on="窗格" class="Pane"("Origin"=T6 {"Horizontal"=0, "Vertical"=650} ("原点")) -> ()  [unwired: 2 in, 2 out]
        n524 = case shown="假" w827 {
          tunnel: [w839 w842] -> w826
          frame False {
            n525 = global read "COD内部交互全局.vi" "配置文件ini"() -> (w841:string)
            n526 = call <vilib>:"Application Directory.vi"() -> ("Application Directory"=w840:path)
            n527 = Build Path(base path=w840, name or relative path=w841) -> (appended path=w839:path)
          }
          frame True {
            n528 = global read "CODMN外部API.vi" "配置文件 path"() -> (w842:path)
          }
        }
        n529 = Bundle By Name(cluster=cluster{"命令":string} {"命令"=""} ("元素"), "命令"="CODMn读取参数" ("名称（未命名）")) -> (w830:cluster{"命令":string})
        n530 = call <vilib>:"Open Config Data.vi"("configuration file path"=w826) -> ("error out"=w836:errorcluster, "refnum"=w833:T8)  [unwired: 8 in, 1 out]
        n531 = Enqueue Element(queue=w829, element=w830, error in (no error)=w828) -> ()  [unwired: 1 in, 3 out]
        n532 = vi-ref "斯坦道CODMn.lvlib:CODMn断电保存全局变量.vi"() -> (w834:refnum<vi>)
        n533 = call <userlib>:"Read Panel from INI__ogtk.vi"("error in (no error)"=w836, "VI ref"=w834, "refnum"=w833) -> ("error out"=w837:errorcluster, "refnum out"=w835:T8)  [unwired: 7 in]
        n534 = call <vilib>:"Close Config Data.vi"("error in (no error)"=w837, "refnum"=w835) -> ("error out"=w825:errorcluster)  [unwired: 8 in, 1 out]
        n535 = call <vilib>:"Clear Errors.vi"("error in (no error)"=w825) -> ()  [unwired: 5 in, 2 out]
      }
      event "布尔": Value Change {
        n536 = event-data() -> ("CtlRef"=w843:refnum<vi>, "NewVal"=w844:bool)  [unwired: 1 in, 4 out]
        n537 = case shown="真" w844 {
          tunnel: w843 -> [_ w847]
          frame False {
            n538 = global write "CODMN外部API.vi" "权限等级"(enum16{"一级权限", "二级权限", "三级权限", "超级权限"}."一级权限" ("权限等级")) -> ()
          }
          frame True {
            n539 = global read "CODMN外部API.vi" "权限等级"() -> (w850:enum16{"一级权限", "二级权限", "三级权限", "超级权限"})
            n540 = global read "CODMN外部API.vi" "权限密码"() -> (w848:u32[])
            n541 = call "密码权限设置.vi"("权限输入"=w850, "权限密码"=w848) -> ("权限输出"=w849:enum16{"一级权限", "二级权限", "三级权限", "超级权限"})  [unwired: 9 in]
            n542 = property class="Bool (严格)"(reference=w847, "Value"=FALSE ("值")) -> ()  [unwired: 1 in, 2 out]
            n543 = global write "CODMN外部API.vi" "权限等级"(w849) -> ()
          }
        }
      }
      event "保存": Mouse Down {
        n544 = event-data() -> ()  [unwired: 1 in, 8 out]
        n545 = local read "通讯状态"() -> (w851:bool)
        n546 = Two Button Dialog(message="确定保存参数，保存参数将会替换原有参数！" ("消息")) -> (T button?=w853:bool)  [unwired: 2 in]
        n547 = case shown="真" w853 {
          tunnel: w851 -> [_ w854]
          frame False {
          }
          frame True {
            n548 = case shown="真" w854 {
              frame False {
                n549 = One Button Dialog(message="保存失败，当前无通讯！" ("消息")) -> ()  [unwired: 1 in, 1 out]
              }
              frame True {
                n550 = One Button Dialog(message="参数保存成功！" ("消息")) -> ()  [unwired: 1 in, 1 out]
                n551 = Build Array("采水泵进样时间/s:", "采水泵润洗时间/s:", "采水泵沉淀时间/s:", "采水泵排液时间/s:") -> (w875:i32[])
                n552 = call "CODMnMB_api.vi"("STEP"=enum16{"open", "read", "write", "close"}."write", "values"="保存参数", "starting address"=u16 4272) -> ("error out"=w881:errorcluster)  [unwired: 6 in, 2 out]
                n553 = local read "加标回收样："() -> (w865:dbl)
                n554 = local read "零点核查样："() -> (w866:dbl)
                n555 = Get Date/Time In Seconds() -> (seconds since 1Jan1904=w871:timestamp)
                n556 = local read "高锰酸钾"() -> (w863:dbl)
                n557 = local read "蒸馏水："() -> (w868:dbl)
                n558 = local read "草酸钠"() -> (w862:dbl)
                n559 = call "CODMnMB_api.vi"("STEP"=enum16{"open", "read", "write", "close"}."write", "Error in"=w881, "values"=w875, "starting address"=u16 5596) -> ("error out"=w870:errorcluster)  [unwired: 5 in, 2 out]
                n560 = local read "硫酸"() -> (w864:dbl)
                n561 = local read "水样："() -> (w869:dbl)
                n562 = local read "标液："() -> (w867:dbl)
                n563 = case shown="真" "更换泵管" {
                  tunnel: ["false" "true"] -> w857
                  frame False {
                  }
                  frame True {
                  }
                }
                n564 = call <vilib>:"Clear Errors.vi"("error in (no error)"=w870) -> ("error out"=w856:errorcluster)  [unwired: 5 in, 1 out]
                n565 = Bundle By Name(cluster=T15 {"时间"=timestamp(0 s since 1904-01-01), "水样计量数"=0, "蒸馏水计量数"=0, "标液计量数"=0, "零点核查计量数"=0, "加标回收计量数"=0, "硫酸计量数"=0, "高锰酸钾计量数"=0, "草酸钠计量数"=0, "更换泵管"=""} ("data"), "时间"=w871, "水样计量数"=w869, "蒸馏水计量数"=w868, "标液计量数"=w867, "零点核查计量数"=w866, "加标回收计量数"=w865, "硫酸计量数"=w864, "高锰酸钾计量数"=w863, "草酸钠计量数"=w862, "更换泵管"=w857) -> (w858:T15)
                n566 = global read "CODMn断电保存全局变量.vi" "数据库类型"() -> (w873:T16)
                n567 = global read "CODMn断电保存全局变量.vi" "Password"() -> (w872:string)
                n568 = call "PLC版CODMn泵校准数据插入.vi"("data"=w858, "Password"=w872, "错误输入（无错误）"=w856, "数据库类型"=w873) -> ("错误输出"=w861:errorcluster)  [unwired: 6 in]
                n569 = flat-sequence {
                  tunnel: w861 -> [_]
                  frame #0 {
                    n570 = local write "更换泵管"(FALSE ("更换泵管")) -> ()
                  }
                }
              }
            }
          }
        }
      }
      event "常规版/认证版", "屏蔽负值": Value Change {
        n571 = event-data() -> ()  [unwired: 1 in, 6 out]
        n572 = flat-sequence {
          frame #0 {
            n573 = global write "CODMn断电保存全局变量.vi" "常规版/认证版"("常规版/认证版") -> ()
            n574 = global write "CODMn断电保存全局变量.vi" "屏蔽负值"("屏蔽负值") -> ()
          }
          frame #1 {
            n575 = call "配置文件保存.vi"() -> ()  [unwired: 12 in]
          }
        }
      }
      event "校准配置": Value Change {
        w905 = "量程选择" ("section")
        n576 = event-data() -> ()  [unwired: 1 in, 6 out]
        n577 = global read "CODMN外部API.vi" "ping"() -> (w909:bool)
        n578 = property on="窗格" class="Pane"("Origin"=T6 {"Horizontal"=0, "Vertical"=1300} ("原点")) -> ()  [unwired: 2 in, 2 out]
        n579 = case shown="假" w909 {
          tunnel: [w987 w990] -> w908
          frame False {
            n580 = global read "COD内部交互全局.vi" "配置文件ini"() -> (w989:string)
            n581 = call <vilib>:"Application Directory.vi"() -> ("Application Directory"=w988:path)
            n582 = Build Path(base path=w988, name or relative path=w989) -> (appended path=w987:path)
          }
          frame True {
            n583 = global read "CODMN外部API.vi" "配置文件 path"() -> (w990:path)
          }
        }
        n584 = Bundle By Name(cluster=cluster{"命令":string} {"命令"=""} ("元素"), "命令"="CODMn读取公式" ("名称（未命名）")) -> (w893:cluster{"命令":string})
        n585 = Enqueue Element(queue=w892, element=w893, error in (no error)=w891) -> ()  [unwired: 1 in, 3 out]
        n586 = call <vilib>:"Open Config Data.vi"("configuration file path"=w908) -> ("error out"=w926:errorcluster, "refnum"=w927:T8)  [unwired: 8 in, 1 out]
        n587 = call-poly <vilib>:"Read Key.vi"("section"="CODMn模型选择" ("key"), "error in (no error)"=w926, "key"="线性和多项式", "refnum"=w927) -> ("error out"=w923:errorcluster, "value"=w925:i32, "refnum out"=w924:T8)  [unwired: 4 in, 1 out]
        n588 = local write "模型"(w925) -> ()
        n589 = call-poly <vilib>:"Read Key.vi"("section"="标线选择", "error in (no error)"=w923, "key"="选用水样", "refnum"=w924) -> ("error out"=w906:errorcluster, "value"=w910:i32, "refnum out"=w907:T8)  [unwired: 4 in, 1 out]
        n590 = local write "选用水样"(w910) -> ()
        n591 = case shown="0, 默认" w910 {
          tunnel: ["葡萄糖标线" ("section") "草酸钠标线" ("section")] -> w932
          frame 0, Default {
          }
          frame 1 {
          }
        }
        n592 = call-poly <vilib>:"Read Key.vi"("section"=w905, "error in (no error)"=w906, "key"=w905, "refnum"=w907) -> ("error out"=w903:errorcluster, "value"=w902:i32, "refnum out"=w904:T8)  [unwired: 4 in, 1 out]
        n593 = local write "量程选择"(w902) -> ()
        n594 = case shown="2" w902 {
          tunnel: ["低量程" "高量程" "0-2量程"] -> w931
          frame 0, Default {
          }
          frame 1 {
          }
          frame 2 {
          }
        }
        n595 = Concatenate Strings(w932, w931) -> (w930:string)
        n596 = call-poly <vilib>:"Read Key.vi"("section"=w930, "error in (no error)"=w903, "key"="浓度1", "refnum"=w904) -> ("error out"=w957:errorcluster, "value"=w955:dbl, "refnum out"=w956:T8)  [unwired: 4 in, 1 out]
        n597 = local write "浓度1"(w955) -> ()
        n598 = call-poly <vilib>:"Read Key.vi"("section"=w930, "error in (no error)"=w957, "key"="浓度2", "refnum"=w956) -> ("error out"=w971:errorcluster, "value"=w958:dbl, "refnum out"=w970:T8)  [unwired: 4 in, 1 out]
        n599 = local write "浓度2"(w958) -> ()
        n600 = call-poly <vilib>:"Read Key.vi"("section"=w930, "error in (no error)"=w971, "key"="浓度3", "refnum"=w970) -> ("error out"=w972:errorcluster, "value"=w960:dbl, "refnum out"=w969:T8)  [unwired: 4 in, 1 out]
        n601 = local write "浓度3"(w960) -> ()
        n602 = call-poly <vilib>:"Read Key.vi"("section"=w930, "error in (no error)"=w972, "key"="泵滴定数1", "refnum"=w969) -> ("error out"=w973:errorcluster, "value"=w962:dbl, "refnum out"=w968:T8)  [unwired: 4 in, 1 out]
        n603 = local write "泵滴定数1"(w962) -> ()
        n604 = call-poly <vilib>:"Read Key.vi"("section"=w930, "error in (no error)"=w973, "key"="泵滴定数2", "refnum"=w968) -> ("error out"=w967:errorcluster, "value"=w965:dbl, "refnum out"=w974:T8)  [unwired: 4 in, 1 out]
        n605 = local write "泵滴定数2"(w965) -> ()
        n606 = call-poly <vilib>:"Read Key.vi"("section"=w930, "error in (no error)"=w967, "key"="泵滴定数3", "refnum"=w974) -> ("error out"=w979:errorcluster, "value"=w978:dbl, "refnum out"=w975:T8)  [unwired: 4 in, 1 out]
        n607 = local write "泵滴定数3"(w978) -> ()
        n608 = call-poly <vilib>:"Read Key.vi"("section"=w930, "error in (no error)"=w979, "key"="浓度4", "refnum"=w975) -> ("error out"=w980:errorcluster, "value"=w916:dbl, "refnum out"=w976:T8)  [unwired: 4 in, 1 out]
        n609 = local write "浓度4"(w916) -> ()
        n610 = call-poly <vilib>:"Read Key.vi"("section"=w930, "error in (no error)"=w980, "key"="浓度5", "refnum"=w976) -> ("error out"=w921:errorcluster, "value"=w915:dbl, "refnum out"=w922:T8)  [unwired: 4 in, 1 out]
        n611 = local write "浓度5"(w915) -> ()
        n612 = call-poly <vilib>:"Read Key.vi"("section"=w930, "error in (no error)"=w921, "key"="泵滴定数4", "refnum"=w922) -> ("error out"=w981:errorcluster, "value"=w914:dbl, "refnum out"=w977:T8)  [unwired: 4 in, 1 out]
        n613 = local write "泵滴定数4"(w914) -> ()
        n614 = call-poly <vilib>:"Read Key.vi"("section"=w930, "error in (no error)"=w981, "key"="泵滴定数5", "refnum"=w977) -> ("error out"=w919:errorcluster, "value"=w913:dbl, "refnum out"=w920:T8)  [unwired: 4 in, 1 out]
        n615 = local write "泵滴定数5"(w913) -> ()
        n616 = call-poly <vilib>:"Read Key.vi"("section"=w930, "error in (no error)"=w919, "key"="当前选用的校准", "refnum"=w920) -> ("error out"=w951:errorcluster, "refnum out"=w952:T8)  [unwired: 4 in, 2 out]
        n617 = call-poly <vilib>:"Read Key.vi"("section"=w930, "error in (no error)"=w951, "key"="启用1", "refnum"=w952) -> ("error out"=w948:errorcluster, "value"=w937:bool, "refnum out"=w949:T8)  [unwired: 4 in, 1 out]
        n618 = local write "启用1"(w937) -> ()
        n619 = call-poly <vilib>:"Read Key.vi"("section"=w930, "error in (no error)"=w948, "key"="启用2", "refnum"=w949) -> ("error out"=w946:errorcluster, "value"=w936:bool, "refnum out"=w947:T8)  [unwired: 4 in, 1 out]
        n620 = local write "启用2"(w936) -> ()
        n621 = call-poly <vilib>:"Read Key.vi"("section"=w930, "error in (no error)"=w946, "key"="启用3", "refnum"=w947) -> ("error out"=w944:errorcluster, "value"=w935:bool, "refnum out"=w945:T8)  [unwired: 4 in, 1 out]
        n622 = local write "启用3"(w935) -> ()
        n623 = call-poly <vilib>:"Read Key.vi"("section"=w930, "error in (no error)"=w944, "key"="启用4", "refnum"=w945) -> ("error out"=w942:errorcluster, "value"=w912:bool, "refnum out"=w943:T8)  [unwired: 4 in, 1 out]
        n624 = local write "启用4"(w912) -> ()
        n625 = call-poly <vilib>:"Read Key.vi"("section"=w930, "error in (no error)"=w942, "key"="启用5", "refnum"=w943) -> ("error out"=w917:errorcluster, "value"=w911:bool, "refnum out"=w918:T8)  [unwired: 4 in, 1 out]
        n626 = local write "启用5"(w911) -> ()
        n627 = call <vilib>:"Close Config Data.vi"("error in (no error)"=w917, "refnum"=w918) -> ("error out"=w896:errorcluster, "file path"=w897:path)  [unwired: 8 in]
        n628 = Open/Create/Replace File(file path (use dialog)=w897, error in=w896) -> (refnum out=w899:refnum<file>, error out=w898:errorcluster)  [unwired: 4 in, 1 out]
        n629 = Flush File(refnum=w899, error in=w898) -> (refnum out=w900:refnum<file>, error out=w901:errorcluster)
        n630 = Close File(refnum=w900, error in=w901) -> ()  [unwired: 2 out]
      }
      event "选用水样": Value Change {
        (unwired) "浓度6" ("key")
        n631 = event-data() -> ()  [unwired: 1 in, 6 out]
        n632 = local read "量程选择"() -> (w1059:enum16{"低量程", "高量程"})
        n633 = property on="窗格" class="Pane"("Origin"=T6 {"Horizontal"=0, "Vertical"=1300} ("原点")) -> ()  [unwired: 2 in, 2 out]
        n634 = case shown="\"葡萄糖\", 默认" "选用水样" {
          tunnel: ["葡萄糖标线" ("section") "草酸钠标线" ("section")] -> w1061
          frame "葡萄糖", Default {
          }
          frame "草酸钠" {
          }
        }
        n635 = global read "CODMN外部API.vi" "ping"() -> (w1048:bool)
        n636 = case shown="\"高量程\"" w1059 {
          tunnel: ["低量程" "高量程"] -> w1060
          frame "低量程", Default {
          }
          frame "高量程" {
          }
        }
        n637 = case shown="假" w1048 {
          tunnel: [w1114 w1117] -> w1047
          frame False {
            n638 = global read "COD内部交互全局.vi" "配置文件ini"() -> (w1116:string)
            n639 = call <vilib>:"Application Directory.vi"() -> ("Application Directory"=w1115:path)
            n640 = Build Path(base path=w1115, name or relative path=w1116) -> (appended path=w1114:path)
          }
          frame True {
            n641 = global read "CODMN外部API.vi" "配置文件 path"() -> (w1117:path)
          }
        }
        n642 = Concatenate Strings(w1061, w1060) -> (w1014:string)
        n643 = call <vilib>:"Open Config Data.vi"("configuration file path"=w1047) -> ("error out"=w1043:errorcluster, "refnum"=w1044:T8)  [unwired: 8 in, 1 out]
        n644 = Bundle By Name(cluster=cluster{"命令":string} {"命令"=""} ("元素"), "命令"="CODMn读取公式" ("名称（未命名）")) -> (w1031:cluster{"命令":string})
        n645 = call-poly <vilib>:"Write Key.vi"("section"="标线选择", "error in (no error)"=w1043, "value"="选用水样", "key"="选用水样", "refnum"=w1044) -> ("error out"=w1040:errorcluster, "refnum out"=w1041:T8)  [unwired: 4 in, 1 out]
        n646 = call-poly <vilib>:"Read Key.vi"("section"=w1014, "error in (no error)"=w1040, "key"="浓度1", "refnum"=w1041) -> ("error out"=w1084:errorcluster, "value"=w1082:dbl, "refnum out"=w1083:T8)  [unwired: 4 in, 1 out]
        n647 = Enqueue Element(queue=w1030, element=w1031, error in (no error)=w1029) -> ()  [unwired: 1 in, 3 out]
        n648 = local write "浓度1"(w1082) -> ()
        n649 = call-poly <vilib>:"Read Key.vi"("section"=w1014, "error in (no error)"=w1084, "key"="浓度2", "refnum"=w1083) -> ("error out"=w1098:errorcluster, "value"=w1085:dbl, "refnum out"=w1097:T8)  [unwired: 4 in, 1 out]
        n650 = local write "浓度2"(w1085) -> ()
        n651 = call-poly <vilib>:"Read Key.vi"("section"=w1014, "error in (no error)"=w1098, "key"="浓度3", "refnum"=w1097) -> ("error out"=w1099:errorcluster, "value"=w1087:dbl, "refnum out"=w1096:T8)  [unwired: 4 in, 1 out]
        n652 = local write "浓度3"(w1087) -> ()
        n653 = call-poly <vilib>:"Read Key.vi"("section"=w1014, "error in (no error)"=w1099, "key"="泵滴定数1", "refnum"=w1096) -> ("error out"=w1100:errorcluster, "value"=w1089:dbl, "refnum out"=w1095:T8)  [unwired: 4 in, 1 out]
        n654 = local write "泵滴定数1"(w1089) -> ()
        n655 = call-poly <vilib>:"Read Key.vi"("section"=w1014, "error in (no error)"=w1100, "key"="泵滴定数2", "refnum"=w1095) -> ("error out"=w1094:errorcluster, "value"=w1092:dbl, "refnum out"=w1101:T8)  [unwired: 4 in, 1 out]
        n656 = local write "泵滴定数2"(w1092) -> ()
        n657 = call-poly <vilib>:"Read Key.vi"("section"=w1014, "error in (no error)"=w1094, "key"="泵滴定数3", "refnum"=w1101) -> ("error out"=w1106:errorcluster, "value"=w1105:dbl, "refnum out"=w1102:T8)  [unwired: 4 in, 1 out]
        n658 = local write "泵滴定数3"(w1105) -> ()
        n659 = call-poly <vilib>:"Read Key.vi"("section"=w1014, "error in (no error)"=w1106, "key"="浓度4", "refnum"=w1102) -> ("error out"=w1107:errorcluster, "value"=w1054:dbl, "refnum out"=w1103:T8)  [unwired: 4 in, 1 out]
        n660 = local write "浓度4"(w1054) -> ()
        n661 = call-poly <vilib>:"Read Key.vi"("section"=w1014, "error in (no error)"=w1107, "key"="浓度5", "refnum"=w1103) -> ("error out"=w1057:errorcluster, "value"=w1053:dbl, "refnum out"=w1058:T8)  [unwired: 4 in, 1 out]
        n662 = local write "浓度5"(w1053) -> ()
        n663 = call-poly <vilib>:"Read Key.vi"("section"=w1014, "error in (no error)"=w1057, "key"="泵滴定数4", "refnum"=w1058) -> ("error out"=w1108:errorcluster, "value"=w1052:dbl, "refnum out"=w1104:T8)  [unwired: 4 in, 1 out]
        n664 = local write "泵滴定数4"(w1052) -> ()
        n665 = call-poly <vilib>:"Read Key.vi"("section"=w1014, "error in (no error)"=w1108, "key"="泵滴定数5", "refnum"=w1104) -> ("error out"=w1055:errorcluster, "value"=w1051:dbl, "refnum out"=w1056:T8)  [unwired: 4 in, 1 out]
        n666 = local write "泵滴定数5"(w1051) -> ()
        n667 = call-poly <vilib>:"Read Key.vi"("section"=w1014, "error in (no error)"=w1055, "key"="当前选用的校准", "refnum"=w1056) -> ("error out"=w1078:errorcluster, "refnum out"=w1079:T8)  [unwired: 4 in, 2 out]
        n668 = call-poly <vilib>:"Read Key.vi"("section"=w1014, "error in (no error)"=w1078, "key"="启用1", "refnum"=w1079) -> ("error out"=w1075:errorcluster, "value"=w1064:bool, "refnum out"=w1076:T8)  [unwired: 4 in, 1 out]
        n669 = local write "启用1"(w1064) -> ()
        n670 = call-poly <vilib>:"Read Key.vi"("section"=w1014, "error in (no error)"=w1075, "key"="启用2", "refnum"=w1076) -> ("error out"=w1073:errorcluster, "value"=w1063:bool, "refnum out"=w1074:T8)  [unwired: 4 in, 1 out]
        n671 = local write "启用2"(w1063) -> ()
        n672 = call-poly <vilib>:"Read Key.vi"("section"=w1014, "error in (no error)"=w1073, "key"="启用3", "refnum"=w1074) -> ("error out"=w1071:errorcluster, "value"=w1062:bool, "refnum out"=w1072:T8)  [unwired: 4 in, 1 out]
        n673 = local write "启用3"(w1062) -> ()
        n674 = call-poly <vilib>:"Read Key.vi"("section"=w1014, "error in (no error)"=w1071, "key"="启用4", "refnum"=w1072) -> ("error out"=w1069:errorcluster, "value"=w1050:bool, "refnum out"=w1070:T8)  [unwired: 4 in, 1 out]
        n675 = local write "启用4"(w1050) -> ()
        n676 = call-poly <vilib>:"Read Key.vi"("section"=w1014, "error in (no error)"=w1069, "key"="启用5", "refnum"=w1070) -> ("error out"=w1011:errorcluster, "value"=w1049:bool, "refnum out"=w1015:T8)  [unwired: 4 in, 1 out]
        n677 = call-poly <vilib>:"Read Key.vi"("section"=w1014, "error in (no error)"=w1011, "key"="零点校准时间", "refnum"=w1015) -> ("error out"=w1027:errorcluster, "value"=w996:string, "refnum out"=w1026:T8)  [unwired: 4 in, 1 out]
        n678 = Unflatten From String(type=timestamp(0 s since 1904-01-01), binary string=w996) -> (value=w997:timestamp)  [unwired: 3 in, 2 out]
        n679 = call-poly <vilib>:"Read Key.vi"("section"=w1014, "error in (no error)"=w1027, "key"="标液1校准时间", "refnum"=w1026) -> ("error out"=w1022:errorcluster, "value"=w999:string, "refnum out"=w1019:T8)  [unwired: 4 in, 1 out]
        n680 = local write "零点校准时间"(w997) -> ()
        n681 = Unflatten From String(type=timestamp(0 s since 1904-01-01), binary string=w999) -> (value=w998:timestamp)  [unwired: 3 in, 2 out]
        n682 = call-poly <vilib>:"Read Key.vi"("section"=w1014, "error in (no error)"=w1022, "key"="标液2校准时间", "refnum"=w1019) -> ("error out"=w1023:errorcluster, "value"=w1002:string, "refnum out"=w1017:T8)  [unwired: 4 in, 1 out]
        n683 = local write "标液校准时间1"(w998) -> ()
        n684 = local write "启用5"(w1049) -> ()
        n685 = Unflatten From String(type=timestamp(0 s since 1904-01-01), binary string=w1002) -> (value=w1001:timestamp)  [unwired: 3 in, 2 out]
        n686 = call-poly <vilib>:"Read Key.vi"("section"=w1014, "error in (no error)"=w1023, "key"="标液3校准时间", "refnum"=w1017) -> ("error out"=w1024:errorcluster, "value"=w1005:string, "refnum out"=w1025:T8)  [unwired: 4 in, 1 out]
        n687 = local write "标液校准时间2"(w1001) -> ()
        n688 = Unflatten From String(type=timestamp(0 s since 1904-01-01), binary string=w1005) -> (value=w1004:timestamp)  [unwired: 3 in, 2 out]
        n689 = call-poly <vilib>:"Read Key.vi"("section"=w1014, "error in (no error)"=w1024, "key"="标液4校准时间", "refnum"=w1025) -> ("error out"=w1012:errorcluster, "value"=w1008:string, "refnum out"=w1013:T8)  [unwired: 4 in, 1 out]
        n690 = call <vilib>:"Close Config Data.vi"("error in (no error)"=w1012, "refnum"=w1013) -> ("error out"=w1034:errorcluster, "file path"=w1035:path)  [unwired: 8 in]
        n691 = Open/Create/Replace File(file path (use dialog)=w1035, error in=w1034) -> (refnum out=w1037:refnum<file>, error out=w1036:errorcluster)  [unwired: 4 in, 1 out]
        n692 = Flush File(refnum=w1037, error in=w1036) -> (refnum out=w1038:refnum<file>, error out=w1039:errorcluster)
        n693 = Close File(refnum=w1038, error in=w1039) -> ()  [unwired: 2 out]
        n694 = local write "标液校准时间3"(w1004) -> ()
        n695 = Unflatten From String(type=timestamp(0 s since 1904-01-01), binary string=w1008) -> (value=w1007:timestamp)  [unwired: 3 in, 2 out]
        n696 = local write "标液校准时间4"(w1007) -> ()
      }
      event "量程选择": Value Change {
        w1171 = "量程选择" ("section")
        n697 = event-data() -> ()  [unwired: 1 in, 6 out]
        n698 = local read "选用水样"() -> (w1186:enum16{"葡萄糖", "草酸钠"})
        n699 = property on="窗格" class="Pane"("Origin"=T6 {"Horizontal"=0, "Vertical"=1300} ("原点")) -> ()  [unwired: 2 in, 2 out]
        n700 = Bundle By Name(cluster=cluster{"命令":string} {"命令"=""} ("元素"), "命令"="CODMn读取公式" ("名称（未命名）")) -> (w1157:cluster{"命令":string})
        n701 = case shown="\"葡萄糖\", 默认" w1186 {
          tunnel: ["葡萄糖标线" ("section") "草酸钠标线" ("section")] -> w1185
          frame "葡萄糖", Default {
          }
          frame "草酸钠" {
          }
        }
        n702 = global read "CODMN外部API.vi" "ping"() -> (w1173:bool)
        n703 = case shown="\"高量程\"" "量程选择" {
          tunnel: ["低量程" "高量程"] -> w1184
          frame "低量程", Default {
          }
          frame "高量程" {
          }
        }
        n704 = Enqueue Element(queue=w1156, element=w1157, error in (no error)=w1155) -> ()  [unwired: 1 in, 3 out]
        n705 = case shown="假" w1173 {
          tunnel: [w1239 w1242] -> w1172
          frame False {
            n706 = global read "COD内部交互全局.vi" "配置文件ini"() -> (w1241:string)
            n707 = call <vilib>:"Application Directory.vi"() -> ("Application Directory"=w1240:path)
            n708 = Build Path(base path=w1240, name or relative path=w1241) -> (appended path=w1239:path)
          }
          frame True {
            n709 = global read "CODMN外部API.vi" "配置文件 path"() -> (w1242:path)
          }
        }
        n710 = Concatenate Strings(w1185, w1184) -> (w1122:string)
        n711 = call <vilib>:"Open Config Data.vi"("configuration file path"=w1172) -> ("error out"=w1170:errorcluster, "refnum"=w1169:T8)  [unwired: 8 in, 1 out]
        n712 = call-poly <vilib>:"Write Key.vi"("section"=w1171, "error in (no error)"=w1170, "value"="量程选择", "key"=w1171, "refnum"=w1169) -> ("error out"=w1166:errorcluster, "refnum out"=w1168:T8)  [unwired: 4 in, 1 out]
        n713 = call-poly <vilib>:"Read Key.vi"("section"=w1122, "error in (no error)"=w1166, "key"="浓度1", "refnum"=w1168) -> ("error out"=w1209:errorcluster, "value"=w1207:dbl, "refnum out"=w1208:T8)  [unwired: 4 in, 1 out]
        n714 = local write "浓度1"(w1207) -> ()
        n715 = call-poly <vilib>:"Read Key.vi"("section"=w1122, "error in (no error)"=w1209, "key"="浓度2", "refnum"=w1208) -> ("error out"=w1223:errorcluster, "value"=w1210:dbl, "refnum out"=w1222:T8)  [unwired: 4 in, 1 out]
        n716 = local write "浓度2"(w1210) -> ()
        n717 = call-poly <vilib>:"Read Key.vi"("section"=w1122, "error in (no error)"=w1223, "key"="浓度3", "refnum"=w1222) -> ("error out"=w1224:errorcluster, "value"=w1212:dbl, "refnum out"=w1221:T8)  [unwired: 4 in, 1 out]
        n718 = local write "浓度3"(w1212) -> ()
        n719 = call-poly <vilib>:"Read Key.vi"("section"=w1122, "error in (no error)"=w1224, "key"="泵滴定数1", "refnum"=w1221) -> ("error out"=w1225:errorcluster, "value"=w1214:dbl, "refnum out"=w1220:T8)  [unwired: 4 in, 1 out]
        n720 = local write "泵滴定数1"(w1214) -> ()
        n721 = call-poly <vilib>:"Read Key.vi"("section"=w1122, "error in (no error)"=w1225, "key"="泵滴定数2", "refnum"=w1220) -> ("error out"=w1219:errorcluster, "value"=w1217:dbl, "refnum out"=w1226:T8)  [unwired: 4 in, 1 out]
        n722 = local write "泵滴定数2"(w1217) -> ()
        n723 = call-poly <vilib>:"Read Key.vi"("section"=w1122, "error in (no error)"=w1219, "key"="泵滴定数3", "refnum"=w1226) -> ("error out"=w1231:errorcluster, "value"=w1230:dbl, "refnum out"=w1227:T8)  [unwired: 4 in, 1 out]
        n724 = local write "泵滴定数3"(w1230) -> ()
        n725 = call-poly <vilib>:"Read Key.vi"("section"=w1122, "error in (no error)"=w1231, "key"="浓度4", "refnum"=w1227) -> ("error out"=w1232:errorcluster, "value"=w1177:dbl, "refnum out"=w1228:T8)  [unwired: 4 in, 1 out]
        n726 = local write "浓度4"(w1177) -> ()
        n727 = call-poly <vilib>:"Read Key.vi"("section"=w1122, "error in (no error)"=w1232, "key"="浓度5", "refnum"=w1228) -> ("error out"=w1182:errorcluster, "value"=w1176:dbl, "refnum out"=w1183:T8)  [unwired: 4 in, 1 out]
        n728 = local write "浓度5"(w1176) -> ()
        n729 = call-poly <vilib>:"Read Key.vi"("section"=w1122, "error in (no error)"=w1182, "key"="泵滴定数4", "refnum"=w1183) -> ("error out"=w1233:errorcluster, "value"=w1175:dbl, "refnum out"=w1229:T8)  [unwired: 4 in, 1 out]
        n730 = local write "泵滴定数4"(w1175) -> ()
        n731 = call-poly <vilib>:"Read Key.vi"("section"=w1122, "error in (no error)"=w1233, "key"="泵滴定数5", "refnum"=w1229) -> ("error out"=w1180:errorcluster, "value"=w1174:dbl, "refnum out"=w1181:T8)  [unwired: 4 in, 1 out]
        n732 = local write "泵滴定数5"(w1174) -> ()
        n733 = call-poly <vilib>:"Read Key.vi"("section"=w1122, "error in (no error)"=w1180, "key"="当前选用的校准", "refnum"=w1181) -> ("error out"=w1203:errorcluster, "refnum out"=w1204:T8)  [unwired: 4 in, 2 out]
        n734 = call-poly <vilib>:"Read Key.vi"("section"=w1122, "error in (no error)"=w1203, "key"="启用1", "refnum"=w1204) -> ("error out"=w1200:errorcluster, "value"=w1189:bool, "refnum out"=w1201:T8)  [unwired: 4 in, 1 out]
        n735 = local write "启用1"(w1189) -> ()
        n736 = call-poly <vilib>:"Read Key.vi"("section"=w1122, "error in (no error)"=w1200, "key"="启用2", "refnum"=w1201) -> ("error out"=w1198:errorcluster, "value"=w1188:bool, "refnum out"=w1199:T8)  [unwired: 4 in, 1 out]
        n737 = local write "启用2"(w1188) -> ()
        n738 = call-poly <vilib>:"Read Key.vi"("section"=w1122, "error in (no error)"=w1198, "key"="启用3", "refnum"=w1199) -> ("error out"=w1196:errorcluster, "value"=w1187:bool, "refnum out"=w1197:T8)  [unwired: 4 in, 1 out]
        n739 = local write "启用3"(w1187) -> ()
        n740 = call-poly <vilib>:"Read Key.vi"("section"=w1122, "error in (no error)"=w1196, "key"="启用4", "refnum"=w1197) -> ("error out"=w1194:errorcluster, "value"=w1179:bool, "refnum out"=w1195:T8)  [unwired: 4 in, 1 out]
        n741 = local write "启用4"(w1179) -> ()
        n742 = call-poly <vilib>:"Read Key.vi"("section"=w1122, "error in (no error)"=w1194, "key"="启用5", "refnum"=w1195) -> ("error out"=w1124:errorcluster, "value"=w1178:bool, "refnum out"=w1123:T8)  [unwired: 4 in, 1 out]
        n743 = call-poly <vilib>:"Read Key.vi"("section"=w1122, "error in (no error)"=w1124, "key"="零点校准时间", "refnum"=w1123) -> ("error out"=w1153:errorcluster, "value"=w1127:string, "refnum out"=w1152:T8)  [unwired: 4 in, 1 out]
        n744 = Unflatten From String(type=timestamp(0 s since 1904-01-01), binary string=w1127) -> (value=w1128:timestamp)  [unwired: 3 in, 2 out]
        n745 = call-poly <vilib>:"Read Key.vi"("section"=w1122, "error in (no error)"=w1153, "key"="标液1校准时间", "refnum"=w1152) -> ("error out"=w1148:errorcluster, "value"=w1130:string, "refnum out"=w1145:T8)  [unwired: 4 in, 1 out]
        n746 = local write "零点校准时间"(w1128) -> ()
        n747 = Unflatten From String(type=timestamp(0 s since 1904-01-01), binary string=w1130) -> (value=w1129:timestamp)  [unwired: 3 in, 2 out]
        n748 = call-poly <vilib>:"Read Key.vi"("section"=w1122, "error in (no error)"=w1148, "key"="标液2校准时间", "refnum"=w1145) -> ("error out"=w1149:errorcluster, "value"=w1133:string, "refnum out"=w1143:T8)  [unwired: 4 in, 1 out]
        n749 = local write "标液校准时间1"(w1129) -> ()
        n750 = local write "启用5"(w1178) -> ()
        n751 = Unflatten From String(type=timestamp(0 s since 1904-01-01), binary string=w1133) -> (value=w1132:timestamp)  [unwired: 3 in, 2 out]
        n752 = call-poly <vilib>:"Read Key.vi"("section"=w1122, "error in (no error)"=w1149, "key"="标液3校准时间", "refnum"=w1143) -> ("error out"=w1150:errorcluster, "value"=w1136:string, "refnum out"=w1151:T8)  [unwired: 4 in, 1 out]
        n753 = local write "标液校准时间2"(w1132) -> ()
        n754 = Unflatten From String(type=timestamp(0 s since 1904-01-01), binary string=w1136) -> (value=w1135:timestamp)  [unwired: 3 in, 2 out]
        n755 = call-poly <vilib>:"Read Key.vi"("section"=w1122, "error in (no error)"=w1150, "key"="标液4校准时间", "refnum"=w1151) -> ("error out"=w1125:errorcluster, "value"=w1139:string, "refnum out"=w1126:T8)  [unwired: 4 in, 1 out]
        n756 = call <vilib>:"Close Config Data.vi"("error in (no error)"=w1125, "refnum"=w1126) -> ("error out"=w1160:errorcluster, "file path"=w1161:path)  [unwired: 8 in]
        n757 = Open/Create/Replace File(file path (use dialog)=w1161, error in=w1160) -> (refnum out=w1163:refnum<file>, error out=w1162:errorcluster)  [unwired: 4 in, 1 out]
        n758 = Flush File(refnum=w1163, error in=w1162) -> (refnum out=w1164:refnum<file>, error out=w1165:errorcluster)
        n759 = Close File(refnum=w1164, error in=w1165) -> ()  [unwired: 2 out]
        n760 = local write "标液校准时间3"(w1135) -> ()
        n761 = Unflatten From String(type=timestamp(0 s since 1904-01-01), binary string=w1139) -> (value=w1138:timestamp)  [unwired: 3 in, 2 out]
        n762 = local write "标液校准时间4"(w1138) -> ()
      }
      event "返回": Value Change {
        w1268 = "CODMn" ("section")
        n763 = event-data() -> ()  [unwired: 1 in, 6 out]
        n764 = property on="窗格" class="Pane"("Origin"=T6 {"Horizontal"=0, "Vertical"=0} ("原点")) -> ()  [unwired: 2 in, 2 out]
        n765 = global read "CODMN外部API.vi" "ping"() -> (w1254:bool)
        n766 = case shown="假" w1254 {
          tunnel: [w1319 w1322] -> w1253
          frame False {
            n767 = global read "COD内部交互全局.vi" "配置文件ini"() -> (w1321:string)
            n768 = call <vilib>:"Application Directory.vi"() -> ("Application Directory"=w1320:path)
            n769 = Build Path(base path=w1320, name or relative path=w1321) -> (appended path=w1319:path)
          }
          frame True {
            n770 = global read "CODMN外部API.vi" "配置文件 path"() -> (w1322:path)
          }
        }
        n771 = call <vilib>:"Open Config Data.vi"("configuration file path"=w1253) -> ("error out"=w1317:errorcluster, "refnum"=w1318:T8)  [unwired: 8 in, 1 out]
        n772 = local read "浓度1"() -> (w1315:dbl)
        n773 = call-poly <vilib>:"Write Key.vi"("section"=w1268, "error in (no error)"=w1317, "value"=w1315, "key"="浓度1", "refnum"=w1318) -> ("error out"=w1314:errorcluster, "refnum out"=w1313:T8)  [unwired: 4 in, 1 out]
        n774 = local read "浓度2"() -> (w1299:dbl)
        n775 = call-poly <vilib>:"Write Key.vi"("section"=w1268, "error in (no error)"=w1314, "value"=w1299, "key"="浓度2", "refnum"=w1313) -> ("error out"=w1312:errorcluster, "refnum out"=w1311:T8)  [unwired: 4 in, 1 out]
        n776 = local read "浓度3"() -> (w1295:dbl)
        n777 = local read "泵滴定数1"() -> (w1293:dbl)
        n778 = call-poly <vilib>:"Write Key.vi"("section"=w1268, "error in (no error)"=w1312, "value"=w1295, "key"="浓度3", "refnum"=w1311) -> ("error out"=w1310:errorcluster, "refnum out"=w1309:T8)  [unwired: 4 in, 1 out]
        n779 = local read "泵滴定数2"() -> (w1291:dbl)
        n780 = call-poly <vilib>:"Write Key.vi"("section"=w1268, "error in (no error)"=w1310, "value"=w1293, "key"="泵滴定数1", "refnum"=w1309) -> ("error out"=w1308:errorcluster, "refnum out"=w1307:T8)  [unwired: 4 in, 1 out]
        n781 = local read "泵滴定数3"() -> (w1289:dbl)
        n782 = call-poly <vilib>:"Write Key.vi"("section"=w1268, "error in (no error)"=w1308, "value"=w1291, "key"="泵滴定数2", "refnum"=w1307) -> ("error out"=w1306:errorcluster, "refnum out"=w1305:T8)  [unwired: 4 in, 1 out]
        n783 = call-poly <vilib>:"Write Key.vi"("section"=w1268, "error in (no error)"=w1306, "value"=w1289, "key"="泵滴定数3", "refnum"=w1305) -> ("error out"=w1304:errorcluster, "refnum out"=w1303:T8)  [unwired: 4 in, 1 out]
        n784 = local read "浓度4"() -> (w1256:dbl)
        n785 = call-poly <vilib>:"Write Key.vi"("section"=w1268, "error in (no error)"=w1304, "value"=w1256, "key"="浓度4", "refnum"=w1303) -> ("error out"=w1297:errorcluster, "refnum out"=w1298:T8)  [unwired: 4 in, 1 out]
        n786 = local read "浓度5"() -> (w1255:dbl)
        n787 = local read "泵滴定数4"() -> (w1257:dbl)
        n788 = call-poly <vilib>:"Write Key.vi"("section"=w1268, "error in (no error)"=w1297, "value"=w1255, "key"="浓度5", "refnum"=w1298) -> ("error out"=w1265:errorcluster, "refnum out"=w1266:T8)  [unwired: 4 in, 1 out]
        n789 = local read "泵滴定数5"() -> (w1258:dbl)
        n790 = call-poly <vilib>:"Write Key.vi"("section"=w1268, "error in (no error)"=w1265, "value"=w1257, "key"="泵滴定数4", "refnum"=w1266) -> ("error out"=w1302:errorcluster, "refnum out"=w1301:T8)  [unwired: 4 in, 1 out]
        n791 = call-poly <vilib>:"Write Key.vi"("section"=w1268, "error in (no error)"=w1302, "value"=w1258, "key"="泵滴定数5", "refnum"=w1301) -> ("error out"=w1263:errorcluster, "refnum out"=w1264:T8)  [unwired: 4 in, 1 out]
        n792 = local read "启用1"() -> (w1277:bool)
        n793 = call-poly <vilib>:"Write Key.vi"("section"=w1268, "error in (no error)"=w1263, "value"=w1277, "key"="启用1", "refnum"=w1264) -> ("error out"=w1273:errorcluster, "refnum out"=w1276:T8)  [unwired: 4 in, 1 out]
        n794 = local read "启用2"() -> (w1274:bool)
        n795 = call-poly <vilib>:"Write Key.vi"("section"=w1268, "error in (no error)"=w1273, "value"=w1274, "key"="启用2", "refnum"=w1276) -> ("error out"=w1284:errorcluster, "refnum out"=w1283:T8)  [unwired: 4 in, 1 out]
        n796 = local read "启用3"() -> (w1272:bool)
        n797 = call-poly <vilib>:"Write Key.vi"("section"=w1268, "error in (no error)"=w1284, "value"=w1272, "key"="启用3", "refnum"=w1283) -> ("error out"=w1282:errorcluster, "refnum out"=w1281:T8)  [unwired: 4 in, 1 out]
        n798 = local read "启用4"() -> (w1260:bool)
        n799 = call-poly <vilib>:"Write Key.vi"("section"=w1268, "error in (no error)"=w1282, "value"=w1260, "key"="启用4", "refnum"=w1281) -> ("error out"=w1280:errorcluster, "refnum out"=w1279:T8)  [unwired: 4 in, 1 out]
        n800 = local read "启用5"() -> (w1259:bool)
        n801 = call-poly <vilib>:"Write Key.vi"("section"=w1268, "error in (no error)"=w1280, "value"=w1259, "key"="启用5", "refnum"=w1279) -> ("error out"=w1261:errorcluster, "refnum out"=w1262:T8)  [unwired: 4 in, 1 out]
        n802 = call <vilib>:"Close Config Data.vi"("error in (no error)"=w1261, "refnum"=w1262) -> ("error out"=w1247:errorcluster, "file path"=w1248:path)  [unwired: 8 in]
        n803 = Open/Create/Replace File(file path (use dialog)=w1248, error in=w1247) -> (refnum out=w1250:refnum<file>, error out=w1249:errorcluster)  [unwired: 4 in, 1 out]
        n804 = Flush File(refnum=w1250, error in=w1249) -> (refnum out=w1251:refnum<file>, error out=w1252:errorcluster)
        n805 = Close File(refnum=w1251, error in=w1252) -> ()  [unwired: 2 out]
      }
      event "关闭", "关闭 3", "关闭 4": Value Change {
        n806 = event-data() -> ()  [unwired: 1 in, 6 out]
        n807 = property on="窗格" class="Pane"("Origin"=T6 {"Horizontal"=0, "Vertical"=0} ("原点")) -> ()  [unwired: 2 in, 2 out]
      }
      event Application Instance Close {
        n808 = event-data() -> ()  [unwired: 1 in, 4 out]
      }
      event "时间校准": Value Change {
        n809 = event-data() -> ()  [unwired: 1 in, 6 out]
        n810 = Get Date/Time In Seconds() -> (seconds since 1Jan1904=w1332:timestamp)
        n811 = Build Array(w1332) -> (w1331:timestamp[])
        n812 = call "DateToHex.vi"("DATE"=w1331) -> ("数组"=w1329:u16[])  [unwired: 10 in]
        n813 = Insert Into Array(array=u16[] [1] ("values"), index=1 ("索引"), new element=w1329) -> (w1325:u16[])
        n814 = call "CODMnMB_api.vi"("STEP"=enum16{"open", "read", "write", "close"}."write", "values"=w1325, "starting address"=u16 4612) -> ("error out"=w1324:errorcluster)  [unwired: 6 in, 2 out]
        n815 = call <vilib>:"Clear Errors.vi"("error in (no error)"=w1324) -> ()  [unwired: 5 in, 2 out]
      }
      event "故障清除": Value Change {
        n816 = event-data() -> ()  [unwired: 1 in, 6 out]
        n817 = call "CODMnMB_api.vi"("STEP"=enum16{"open", "read", "write", "close"}."write", "values"=u16[] [1], "starting address"=u16 4611) -> ()  [unwired: 6 in, 3 out]
      }
      event "仪器参数": Value Change {
        n818 = event-data() -> ()  [unwired: 1 in, 6 out]
        n819 = global read "CODMn断电保存全局变量.vi" "CODMn仪器参数"() -> (w1336:T5)
        n820 = call "仪器参数设置.vi"("氨氮仪器参数"=w1336) -> ("仪器参数设置输出"=w1337:T17)  [unwired: 10 in]
        n821 = Unbundle By Name(w1337) -> ("确定"=w1338:bool)
        n822 = case shown="真" w1338 {
          tunnel: w1337 -> [_ w1340]
          tunnel: w1336 -> [_ w1339]
          frame False {
          }
          frame True {
            n823 = flat-sequence {
              tunnel: w1340 -> [w1359]
              tunnel: w1339 -> [w1358]
              frame #0 {
                n824 = Unbundle By Name(w1359) -> ("测量量程"=w1357:dbl, "测量精度"=w1356:dbl, "测量间隔"=w1342:dbl, "消解温度"=w1355:dbl, "消解时长"=w1354:dbl, "空白校准时间"=w1353:timestamp, "曲线截距"=w1352:dbl, "曲线斜率"=w1351:dbl, "测量检出限"=w1350:dbl, "测量信号值"=w1349:dbl, "线性相关系数"=w1348:dbl, "二次多项式系数"=w1347:dbl, "标样校准时间"=w1346:timestamp, "稀释倍数"=w1345:dbl)
                n825 = Bundle By Name(cluster=w1358, "测量量程"=w1357, "测量精度"=w1356, "测量间隔"=w1342, "消解温度"=w1355, "消解时长"=w1354, "空白校准时间"=w1353, "曲线截距"=w1352, "曲线斜率"=w1351, "测量检出限"=w1350, "测量信号值"=w1349, "线性相关系数"=w1348, "二次多项式系数"=w1347, "标样校准时间"=w1346, "稀释倍数"=w1345) -> (w1344:T5)
                n826 = global read "CODMn断电保存全局变量.vi" "运行周期"() -> (w1343:T4)
                n827 = global write "CODMn断电保存全局变量.vi" "CODMn仪器参数"(w1344) -> ()
                n828 = Bundle By Name(cluster=w1343, "测量间隔"=w1342) -> (w1341:T4)
                n829 = global write "CODMn断电保存全局变量.vi" "运行周期"(w1341) -> ()
              }
              frame #1 {
                n830 = call "配置文件保存.vi"() -> ()  [unwired: 12 in]
              }
            }
          }
        }
      }
      event "跨度量程选择", "跨度液浓度", "零点核查量程选择", "零点核查浓度", "标样浓度", "标样核查量程选择", "加标回收量程：", "跨度值", "标准液偏差", "跨度液偏差", "零点液偏差", "标准液自动补测", "跨度液自动补测", "零点液自动补测": Value Change {
        n831 = event-data() -> ()  [unwired: 1 in, 6 out]
        n832 = flat-sequence {
          frame #0 {
            n833 = global write "CODMn断电保存全局变量.vi" "标样浓度"("标样浓度") -> ()
            n834 = global write "CODMn断电保存全局变量.vi" "零点核查浓度"("零点核查浓度") -> ()
            n835 = global write "CODMn断电保存全局变量.vi" "跨度液浓度"("跨度液浓度") -> ()
            n836 = global write "CODMn断电保存全局变量.vi" "CODMn跨度量程选择"("跨度量程选择") -> ()
            n837 = global write "CODMn断电保存全局变量.vi" "加标回收量程选择"("加标回收量程：") -> ()
            n838 = global write "CODMn断电保存全局变量.vi" "跨度值"("跨度值") -> ()
            n839 = global write "CODMn断电保存全局变量.vi" "标样核查量程选择"("标样核查量程选择") -> ()
            n840 = global write "CODMn断电保存全局变量.vi" "零点核查量程选择"("零点核查量程选择") -> ()
            n841 = global write "CODMn断电保存全局变量.vi" "零点核查自动补测"("零点液自动补测") -> ()
            n842 = global write "CODMn断电保存全局变量.vi" "跨度核查自动补测"("跨度液自动补测") -> ()
            n843 = global write "CODMn断电保存全局变量.vi" "标样核查自动补测"("标准液自动补测") -> ()
            n844 = global write "CODMn断电保存全局变量.vi" "标准液标准偏差"("标准液偏差") -> ()
            n845 = global write "CODMn断电保存全局变量.vi" "跨度标准液偏差"("跨度液偏差") -> ()
            n846 = global write "CODMn断电保存全局变量.vi" "零点标准液偏差"("零点液偏差") -> ()
          }
          frame #1 {
            n847 = call "配置文件保存.vi"() -> ()  [unwired: 12 in]
          }
        }
      }
      event "校准1", "校准2", "校准3", "校准4", "校准5": Value Change {
        n848 = event-data() -> ()  [unwired: 1 in, 6 out]
        n849 = flat-sequence {
          tunnel: w1377 -> [w1386]
          tunnel: [w1386] -> w1379
          tunnel: w1374 -> [w1385]
          tunnel: [w1385] -> w1376
          tunnel: w1379 -> [w1421]
          tunnel: [w1421] -> w1378
          tunnel: w1376 -> [w1420]
          tunnel: [w1420] -> w1375
          tunnel: w1378 -> [w1448]
          tunnel: w1375 -> [w1447]
          frame #0 {
            n850 = Build Array("校准1", "校准2", "校准3", "校准4", "校准5") -> (w1389:bool[])
            n851 = for {
              tunnel: w1389 -> [w1403] mode=indexing
              tunnel: [w1395] -> w1380
              i -> [w1396]
              n852 = case shown="4" w1396 {
                tunnel: ["浓度1" "浓度2" "浓度3" "浓度4" "浓度5"] -> w1399
                frame 0, Default {
                }
                frame 1 {
                }
                frame 2 {
                }
                frame 3 {
                }
                frame 4 {
                }
              }
              n853 = Multiply(x=w1399, y=100.0) -> (x*y=w1397:dbl)
              n854 = Insert Into Array(array=u16[] [] ("values"), index=0 ("索引"), new element=w1397) -> (w1400:u16[])
              n855 = case shown="真" w1403 {
                tunnel: w1400 -> [_ w1412]
                tunnel: w1396 -> [_ w1414]
                tunnel: [_ w1409] -> w1395
                frame False {
                }
                frame True {
                  n856 = Increment(x=w1414) -> (x+1=w1410:i32)
                  n857 = global write "COD内部交互全局.vi" "当前校准"(w1410) -> ()
                  n858 = call "CODMnMB_api.vi"("STEP"=enum16{"open", "read", "write", "close"}."write", "values"=w1412, "starting address"=u16 4274) -> ("error out"=w1409:errorcluster)  [unwired: 6 in, 2 out]
                }
              }
            }
            n859 = local read "量程选择"() -> (w1382:enum16{"低量程", "高量程"})
            n860 = case shown="\"高量程\"" w1382 {
              tunnel: [u16[] [0] ("values") u16[] [1] ("values")] -> w1381
              frame "低量程", Default {
              }
              frame "高量程" {
              }
            }
            n861 = call "CODMnMB_api.vi"("STEP"=enum16{"open", "read", "write", "close"}."write", "Error in"=w1380, "values"=w1381, "starting address"=u16 4276) -> ()  [unwired: 5 in, 3 out]
          }
          frame #1 {
            n862 = global read "COD内部交互全局.vi" "当前校准"() -> (w1422:i32)
            n863 = case shown="5" w1422 {
              tunnel: [w1430 w1431 w1432 w1433 w1434] -> w1418
              frame 1, Default {
                n864 = local read "浓度1"() -> (w1430:dbl)
              }
              frame 2 {
                n865 = local read "浓度2"() -> (w1431:dbl)
              }
              frame 3 {
                n866 = local read "浓度3"() -> (w1432:dbl)
              }
              frame 4 {
                n867 = local read "浓度4"() -> (w1433:dbl)
              }
              frame 5 {
                n868 = local read "浓度5"() -> (w1434:dbl)
              }
            }
            n869 = Number To Decimal String(number=w1418) -> (decimal integer string=w1417:string)  [unwired: 1 in]
            n870 = Concatenate Strings("仪器校准中!\n当前校准浓度为:", w1417, "mg/L" ("字符串")) -> (w1415:string)
            n871 = Not Equal To 0?(x=w1418) -> (x != 0?=w1426:bool)
            n872 = global write "COD内部交互全局.vi" "校准内容显示"(w1415) -> ()
            n873 = case shown="真" w1426 {
              tunnel: [u16 8 ("address") u16 9 ("address")] -> w1429
              tunnel: ["校零" ("测量模式") "校标" ("测量模式")] -> _
              frame False {
              }
              frame True {
              }
            }
            n874 = Insert Into Array(array=u16[] [] ("values"), index=0 ("索引"), new element=w1429) -> (w1423:u16[])
            n875 = call "CODMnMB_api.vi"("STEP"=enum16{"open", "read", "write", "close"}."write", "values"=w1423, "starting address"=u16 4608 ("address")) -> ()  [unwired: 6 in, 3 out]
          }
          frame #2 {
            n876 = local read "选用水样"() -> (w1456:enum16{"葡萄糖", "草酸钠"})
            n877 = global read "CODMN外部API.vi" "ping"() -> (w1446:bool)
            n878 = case shown="假" w1446 {
              tunnel: [w1464 w1467] -> w1445
              frame False {
                n879 = global read "COD内部交互全局.vi" "配置文件ini"() -> (w1466:string)
                n880 = call <vilib>:"Application Directory.vi"() -> ("Application Directory"=w1465:path)
                n881 = Build Path(base path=w1465, name or relative path=w1466) -> (appended path=w1464:path)
              }
              frame True {
                n882 = global read "CODMN外部API.vi" "配置文件 path"() -> (w1467:path)
              }
            }
            n883 = local read "量程选择"() -> (w1455:enum16{"低量程", "高量程"})
            n884 = case shown="\"葡萄糖\", 默认" w1456 {
              tunnel: ["葡萄糖标线" ("section") "草酸钠标线" ("section")] -> w1457
              frame "葡萄糖", Default {
              }
              frame "草酸钠" {
              }
            }
            n885 = Bundle By Name(cluster=cluster{"命令":string} {"命令"=""} ("元素"), "命令"="CODMn读取参数" ("名称（未命名）")) -> (w1452:cluster{"命令":string})
            n886 = case shown="\"低量程\", 默认" w1455 {
              tunnel: ["低量程" "高量程"] -> w1458
              frame "低量程", Default {
              }
              frame "高量程" {
              }
            }
            n887 = global read "COD内部交互全局.vi" "当前校准"() -> (w1453:i32)
            n888 = Enqueue Element(queue=w1448, element=w1452, timeout in ms (-1)=1000 ("超时毫秒(-1)"), error in (no error)=w1447) -> ()  [unwired: 3 out]
            n889 = Concatenate Strings(w1457, w1458) -> (w1454:string)
            n890 = call <vilib>:"Open Config Data.vi"("configuration file path"=w1445) -> ("error out"=w1462:errorcluster, "refnum"=w1463:T8)  [unwired: 8 in, 1 out]
            n891 = call-poly <vilib>:"Write Key.vi"("section"=w1454, "error in (no error)"=w1462, "value"=w1453, "key"="当前选用的校准" ("section"), "refnum"=w1463) -> ("error out"=w1459:errorcluster, "refnum out"=w1460:T8)  [unwired: 4 in, 1 out]
            n892 = call <vilib>:"Close Config Data.vi"("error in (no error)"=w1459, "refnum"=w1460) -> ("error out"=w1439:errorcluster, "file path"=w1440:path)  [unwired: 8 in]
            n893 = Open/Create/Replace File(file path (use dialog)=w1440, error in=w1439) -> (refnum out=w1442:refnum<file>, error out=w1441:errorcluster)  [unwired: 4 in, 1 out]
            n894 = Flush File(refnum=w1442, error in=w1441) -> (refnum out=w1443:refnum<file>, error out=w1444:errorcluster)
            n895 = Close File(refnum=w1443, error in=w1444) -> ()  [unwired: 2 out]
          }
        }
      }
      event "水样量程选择:", "低切高阈值:", "高切低阈值:": Value Change {
        n896 = event-data() -> ()  [unwired: 1 in, 6 out]
        n897 = flat-sequence {
          frame #0 {
            n898 = global write "CODMn断电保存全局变量.vi" "高切低阈值:"("高切低阈值:") -> ()
            n899 = global write "CODMn断电保存全局变量.vi" "自动切换量程:"("水样量程选择:") -> ()
            n900 = global write "CODMn断电保存全局变量.vi" "低切高阈值:"("低切高阈值:") -> ()
          }
          frame #1 {
            n901 = call "配置文件保存.vi"() -> ()  [unwired: 12 in]
          }
        }
      }
      event "模型": Value Change {
        n902 = event-data() -> ()  [unwired: 1 in, 6 out]
        n903 = global read "CODMN外部API.vi" "ping"() -> (w1482:bool)
        n904 = case shown="假" w1482 {
          tunnel: [w1490 w1493] -> w1481
          frame False {
            n905 = global read "COD内部交互全局.vi" "配置文件ini"() -> (w1492:string)
            n906 = call <vilib>:"Application Directory.vi"() -> ("Application Directory"=w1491:path)
            n907 = Build Path(base path=w1491, name or relative path=w1492) -> (appended path=w1490:path)
          }
          frame True {
            n908 = global read "CODMN外部API.vi" "配置文件 path"() -> (w1493:path)
          }
        }
        n909 = call <vilib>:"Open Config Data.vi"("configuration file path"=w1481) -> ("error out"=w1488:errorcluster, "refnum"=w1489:T8)  [unwired: 8 in, 1 out]
        n910 = local read "模型"() -> (w1483:enum32{"线性", "多项式", "折线"})
        n911 = call-poly <vilib>:"Write Key.vi"("section"="CODMn模型选择" ("key"), "error in (no error)"=w1488, "value"=w1483, "key"="线性和多项式", "refnum"=w1489) -> ("error out"=w1484:errorcluster, "refnum out"=w1485:T8)  [unwired: 4 in, 1 out]
        n912 = call <vilib>:"Close Config Data.vi"("error in (no error)"=w1484, "refnum"=w1485) -> ("error out"=w1475:errorcluster, "file path"=w1476:path)  [unwired: 8 in]
        n913 = Open/Create/Replace File(file path (use dialog)=w1476, error in=w1475) -> (refnum out=w1478:refnum<file>, error out=w1477:errorcluster)  [unwired: 4 in, 1 out]
        n914 = Flush File(refnum=w1478, error in=w1477) -> (refnum out=w1479:refnum<file>, error out=w1480:errorcluster)
        n915 = Close File(refnum=w1479, error in=w1480) -> ()  [unwired: 2 out]
      }
      event "浓度1", "浓度2", "浓度3", "泵滴定数1", "泵滴定数2", "泵滴定数3", "启用1", "启用2", "启用3", "浓度4", "浓度5", "泵滴定数4", "泵滴定数5", "启用4", "启用5", "标液校准时间1", "标液校准时间2", "标液校准时间3", "标液校准时间4", "零点校准时间": Value Change {
        n916 = event-data() -> ()  [unwired: 1 in, 6 out]
        n917 = local read "选用水样"() -> (w1546:enum16{"葡萄糖", "草酸钠"})
        n918 = local read "量程选择"() -> (w1545:enum16{"低量程", "高量程"})
        n919 = case shown="\"葡萄糖\", 默认" w1546 {
          tunnel: ["葡萄糖标线" ("section") "草酸钠标线" ("section")] -> w1550
          frame "葡萄糖", Default {
          }
          frame "草酸钠" {
          }
        }
        n920 = case shown="\"高量程\"" w1545 {
          tunnel: ["低量程" "高量程"] -> w1544
          frame "低量程", Default {
          }
          frame "高量程" {
          }
        }
        n921 = global read "CODMN外部API.vi" "ping"() -> (w1531:bool)
        n922 = case shown="假" w1531 {
          tunnel: [w1628 w1631] -> w1530
          frame False {
            n923 = global read "COD内部交互全局.vi" "配置文件ini"() -> (w1630:string)
            n924 = call <vilib>:"Application Directory.vi"() -> ("Application Directory"=w1629:path)
            n925 = Build Path(base path=w1629, name or relative path=w1630) -> (appended path=w1628:path)
          }
          frame True {
            n926 = global read "CODMN外部API.vi" "配置文件 path"() -> (w1631:path)
          }
        }
        n927 = Concatenate Strings(w1550, w1544) -> (w1508:string)
        n928 = call <vilib>:"Open Config Data.vi"("configuration file path"=w1530) -> ("error out"=w1599:errorcluster, "refnum"=w1600:T8)  [unwired: 8 in, 1 out]
        n929 = local read "模型"() -> (w1495:enum32{"线性", "多项式", "折线"})
        n930 = case shown="\"折线\"" w1495 {
          tunnel: [9999.0 ("泵滴定数5") 9999.0 ("泵滴定数5") w1603] -> w1494
          frame "线性", Default {
          }
          frame "多项式" {
          }
          frame "折线" {
            n931 = local read "泵滴定数5"() -> (w1610:dbl)
            n932 = local read "泵滴定数3"() -> (w1612:dbl)
            n933 = local read "泵滴定数2"() -> (w1613:dbl)
            n934 = local read "泵滴定数4"() -> (w1611:dbl)
            n935 = local read "泵滴定数1"() -> (w1614:dbl)
            n936 = Build Array(w1614, w1613, w1612, w1611, w1610) -> (w1609:dbl[])
            n937 = local read "启用5"() -> (w1615:bool)
            n938 = local read "启用1"() -> (w1619:bool)
            n939 = local read "启用2"() -> (w1618:bool)
            n940 = local read "启用3"() -> (w1617:bool)
            n941 = local read "启用4"() -> (w1616:bool)
            n942 = Build Array(w1619, w1618, w1617, w1616, w1615) -> (w1608:bool[])
            n943 = for {
              tunnel: w1609 -> [w1622] mode=indexing
              tunnel: w1608 -> [w1623] mode=indexing
              shift-right: [w1621] -> w1606
              shift-left: dbl[] [] -> [w1620]
              n944 = case shown="假" w1623 {
                tunnel: w1622 -> [_ w1627]
                tunnel: w1620 -> [w1624 w1626]
                tunnel: [w1624 w1625] -> w1621
                frame False {
                }
                frame True {
                  n945 = Build Array (concatenate)(w1626, w1627) -> (w1625:dbl[])
                }
              }
            }
            n946 = Sort 1D Array(array=w1606) -> (sorted array=w1605:dbl[])
            n947 = Index Array(array=w1605, index=1 ("索引")) -> (element=w1603:dbl)
          }
        }
        n948 = local read "浓度1"() -> (w1597:dbl)
        n949 = call-poly <vilib>:"Write Key.vi"("section"=w1508, "error in (no error)"=w1599, "value"=w1597, "key"="浓度1", "refnum"=w1600) -> ("error out"=w1596:errorcluster, "refnum out"=w1595:T8)  [unwired: 4 in, 1 out]
        n950 = local read "浓度2"() -> (w1581:dbl)
        n951 = call-poly <vilib>:"Write Key.vi"("section"=w1508, "error in (no error)"=w1596, "value"=w1581, "key"="浓度2", "refnum"=w1595) -> ("error out"=w1594:errorcluster, "refnum out"=w1593:T8)  [unwired: 4 in, 1 out]
        n952 = local read "浓度3"() -> (w1577:dbl)
        n953 = local read "泵滴定数1"() -> (w1575:dbl)
        n954 = call-poly <vilib>:"Write Key.vi"("section"=w1508, "error in (no error)"=w1594, "value"=w1577, "key"="浓度3", "refnum"=w1593) -> ("error out"=w1592:errorcluster, "refnum out"=w1591:T8)  [unwired: 4 in, 1 out]
        n955 = local read "泵滴定数2"() -> (w1573:dbl)
        n956 = call-poly <vilib>:"Write Key.vi"("section"=w1508, "error in (no error)"=w1592, "value"=w1575, "key"="泵滴定数1", "refnum"=w1591) -> ("error out"=w1590:errorcluster, "refnum out"=w1589:T8)  [unwired: 4 in, 1 out]
        n957 = local read "泵滴定数3"() -> (w1571:dbl)
        n958 = call-poly <vilib>:"Write Key.vi"("section"=w1508, "error in (no error)"=w1590, "value"=w1573, "key"="泵滴定数2", "refnum"=w1589) -> ("error out"=w1588:errorcluster, "refnum out"=w1587:T8)  [unwired: 4 in, 1 out]
        n959 = call-poly <vilib>:"Write Key.vi"("section"=w1508, "error in (no error)"=w1588, "value"=w1571, "key"="泵滴定数3", "refnum"=w1587) -> ("error out"=w1586:errorcluster, "refnum out"=w1585:T8)  [unwired: 4 in, 1 out]
        n960 = local read "浓度4"() -> (w1543:dbl)
        n961 = local write "公式切换阈值滴定数(0-9999)"(w1494) -> ()
        n962 = call-poly <vilib>:"Write Key.vi"("section"=w1508, "error in (no error)"=w1586, "value"=w1543, "key"="浓度4", "refnum"=w1585) -> ("error out"=w1579:errorcluster, "refnum out"=w1580:T8)  [unwired: 4 in, 1 out]
        n963 = local read "浓度5"() -> (w1542:dbl)
        n964 = local read "泵滴定数4"() -> (w1539:dbl)
        n965 = call-poly <vilib>:"Write Key.vi"("section"=w1508, "error in (no error)"=w1579, "value"=w1542, "key"="浓度5", "refnum"=w1580) -> ("error out"=w1540:errorcluster, "refnum out"=w1541:T8)  [unwired: 4 in, 1 out]
        n966 = local read "泵滴定数5"() -> (w1538:dbl)
        n967 = call-poly <vilib>:"Write Key.vi"("section"=w1508, "error in (no error)"=w1540, "value"=w1539, "key"="泵滴定数4", "refnum"=w1541) -> ("error out"=w1584:errorcluster, "refnum out"=w1583:T8)  [unwired: 4 in, 1 out]
        n968 = local read "零点校准时间"() -> (w1505:timestamp)
        n969 = call-poly <vilib>:"Write Key.vi"("section"=w1508, "error in (no error)"=w1584, "value"=w1538, "key"="泵滴定数5", "refnum"=w1583) -> ("error out"=w1536:errorcluster, "refnum out"=w1537:T8)  [unwired: 4 in, 1 out]
        n970 = local read "启用1"() -> (w1559:bool)
        n971 = local read "标液校准时间1"() -> (w1503:timestamp)
        n972 = Flatten To String(anything=w1505) -> (data string=w1504:string)  [unwired: 3 in, 2 out]
        n973 = call-poly <vilib>:"Write Key.vi"("section"=w1508, "error in (no error)"=w1536, "value"=w1559, "key"="启用1", "refnum"=w1537) -> ("error out"=w1555:errorcluster, "refnum out"=w1558:T8)  [unwired: 4 in, 1 out]
        n974 = Flatten To String(anything=w1503) -> (data string=w1502:string)  [unwired: 3 in, 2 out]
        n975 = local read "启用2"() -> (w1556:bool)
        n976 = local read "标液校准时间2"() -> (w1500:timestamp)
        n977 = call-poly <vilib>:"Write Key.vi"("section"=w1508, "error in (no error)"=w1555, "value"=w1556, "key"="启用2", "refnum"=w1558) -> ("error out"=w1566:errorcluster, "refnum out"=w1565:T8)  [unwired: 4 in, 1 out]
        n978 = Flatten To String(anything=w1500) -> (data string=w1501:string)  [unwired: 3 in, 2 out]
        n979 = local read "启用3"() -> (w1554:bool)
        n980 = local read "标液校准时间3"() -> (w1497:timestamp)
        n981 = call-poly <vilib>:"Write Key.vi"("section"=w1508, "error in (no error)"=w1566, "value"=w1554, "key"="启用3", "refnum"=w1565) -> ("error out"=w1564:errorcluster, "refnum out"=w1563:T8)  [unwired: 4 in, 1 out]
        n982 = local read "启用4"() -> (w1532:bool)
        n983 = Flatten To String(anything=w1497) -> (data string=w1496:string)  [unwired: 3 in, 2 out]
        n984 = call-poly <vilib>:"Write Key.vi"("section"=w1508, "error in (no error)"=w1564, "value"=w1532, "key"="启用4", "refnum"=w1563) -> ("error out"=w1562:errorcluster, "refnum out"=w1561:T8)  [unwired: 4 in, 1 out]
        n985 = local read "标液校准时间4"() -> (w1499:timestamp)
        n986 = local read "启用5"() -> (w1533:bool)
        n987 = Flatten To String(anything=w1499) -> (data string=w1498:string)  [unwired: 3 in, 2 out]
        n988 = local read "选用水样"() -> (w1549:enum16{"葡萄糖", "草酸钠"})
        n989 = call-poly <vilib>:"Write Key.vi"("section"=w1508, "error in (no error)"=w1562, "value"=w1533, "key"="启用5", "refnum"=w1561) -> ("error out"=w1534:errorcluster, "refnum out"=w1535:T8)  [unwired: 4 in, 1 out]
        n990 = call-poly <vilib>:"Write Key.vi"("section"="标线选择", "error in (no error)"=w1534, "value"=w1549, "key"="选用水样", "refnum"=w1535) -> ("error out"=w1514:errorcluster, "refnum out"=w1515:T8)  [unwired: 4 in, 1 out]
        n991 = call-poly <vilib>:"Write Key.vi"("section"=w1508, "error in (no error)"=w1514, "value"=w1504, "key"="零点校准时间", "refnum"=w1515) -> ("error out"=w1522:errorcluster, "refnum out"=w1521:T8)  [unwired: 4 in, 1 out]
        n992 = call-poly <vilib>:"Write Key.vi"("section"=w1508, "error in (no error)"=w1522, "value"=w1502, "key"="标液1校准时间", "refnum"=w1521) -> ("error out"=w1517:errorcluster, "refnum out"=w1510:T8)  [unwired: 4 in, 1 out]
        n993 = call-poly <vilib>:"Write Key.vi"("section"=w1508, "error in (no error)"=w1517, "value"=w1501, "key"="标液2校准时间", "refnum"=w1510) -> ("error out"=w1518:errorcluster, "refnum out"=w1507:T8)  [unwired: 4 in, 1 out]
        n994 = call-poly <vilib>:"Write Key.vi"("section"=w1508, "error in (no error)"=w1518, "value"=w1496, "key"="标液3校准时间", "refnum"=w1507) -> ("error out"=w1519:errorcluster, "refnum out"=w1520:T8)  [unwired: 4 in, 1 out]
        n995 = call-poly <vilib>:"Write Key.vi"("section"=w1508, "error in (no error)"=w1519, "value"=w1498, "key"="标液4校准时间", "refnum"=w1520) -> ("error out"=w1512:errorcluster, "refnum out"=w1513:T8)  [unwired: 4 in, 1 out]
        n996 = call <vilib>:"Close Config Data.vi"("error in (no error)"=w1512, "refnum"=w1513) -> ("error out"=w1524:errorcluster, "file path"=w1525:path)  [unwired: 8 in]
        n997 = Open/Create/Replace File(file path (use dialog)=w1525, error in=w1524) -> (refnum out=w1527:refnum<file>, error out=w1526:errorcluster)  [unwired: 4 in, 1 out]
        n998 = Flush File(refnum=w1527, error in=w1526) -> (refnum out=w1528:refnum<file>, error out=w1529:errorcluster)
        n999 = Close File(refnum=w1528, error in=w1529) -> ()  [unwired: 2 out]
      }
      event "读取": Value Change {
        (unwired) u16 94 ("number of holding registers")
        (unwired) u16 4616 ("starting address")
        n1000 = event-data() -> ()  [unwired: 1 in, 6 out]
        n1001 = Bundle By Name(cluster=cluster{"命令":string} {"命令"=""} ("元素"), "命令"="CODMn读取公式" ("名称（未命名）")) -> (w1636:cluster{"命令":string})
        n1002 = Enqueue Element(queue=w1640, element=w1636, error in (no error)=w1639) -> ()  [unwired: 1 in, 3 out]
      }
      event "写入": Mouse Down {
        n1003 = event-data() -> ()  [unwired: 1 in, 8 out]
        n1004 = Two Button Dialog(message="即将将左侧拟合公式写入仪器当前量程\n请选择是否写入？" ("消息"), 2:"确定" ("T按钮名称（“确定”）")) -> (T button?=w1641:bool)  [unwired: 1 in]
        n1005 = case shown="真" w1641 {
          frame True {
            n1006 = local read "量程选择"() -> (w1647:enum16{"低量程", "高量程"})
            n1007 = local read "公式切换阈值滴定数(0-9999)"() -> (w1646:u16)
            n1008 = Cluster To Array(cluster="方程系数") -> (array=w1650:dbl[])
            "公式系数" <- w1650
            n1009 = local read "模型"() -> (w1648:enum32{"线性", "多项式", "折线"})
            n1010 = call "公式写入.vi"("公式 2"="方程系数 2", "公式切换阈值滴定数(0-9999)"=w1646, "公式"="方程系数", "量程选择"=w1647, "模型"=w1648) -> ("error out"=w1649:errorcluster)  [unwired: 6 in]
            n1011 = Index Array(array=w1650) -> (element #1=w1653:dbl, element #2=w1651:dbl, element #3=w1652:dbl)  [unwired: 3 in]
            n1012 = case shown="无错误" w1649 {
              tunnel: ["写入成功！" "写入失败！"] -> w1654
              tunnel: w1651 -> [w1660 _]
              tunnel: w1653 -> [w1661 _]
              tunnel: w1652 -> [w1662 _]
              tunnel: w1647 -> [_ _]
              frame No Error {
                n1013 = Number To Fractional String(number=w1660) -> (F-format string=w1664:string)  [unwired: 3 in]
                n1014 = Number To Fractional String(number=w1661) -> (F-format string=w1665:string)  [unwired: 3 in]
                n1015 = Number To Fractional String(number=w1662) -> (F-format string=w1663:string)  [unwired: 3 in]
                n1016 = property on="模型" class="Enum (严格)"() -> ("RingText.Text"=w1658:string)  [unwired: 2 in, 2 out]
                n1017 = property on="量程选择" class="Enum (严格)"() -> ("RingText.Text"=w1671:string)  [unwired: 2 in, 2 out]
                n1018 = Concatenate Strings("变更后:" ("table输入"), "K:" ("字符串"), w1665, "B:" ("字符串"), w1664, "X^2:" ("字符串"), w1663) -> (w1657:string)
                n1019 = Concatenate Strings(w1658, w1671, "公式改变" ("日志信息")) -> (w1655:string)
                n1020 = local write "存校准信息"(TRUE ("存校准信息")) -> ()
                n1021 = call "CODMn日志存储 (子VI).vi"("流程参数"=w1657, "参数"="CODMn" ("table输入"), "日志信息"=w1655) -> ()  [unwired: 9 in]
              }
              frame Error {
              }
            }
            n1022 = One Button Dialog(message=w1654) -> ()  [unwired: 1 in, 1 out]
          }
          frame False {
          }
        }
      }
      event "滴定曲线", "温度曲线": Value Change {
        n1023 = event-data() -> ("CtlRef"=w1675:refnum<vi>)  [unwired: 1 in, 5 out]
        n1024 = property class="Bool"(reference=w1675) -> ("Label.Text"=w1674:string)  [unwired: 1 in, 2 out]
        n1025 = case shown="\"温度曲线\", 默认" w1674 {
          tunnel: [T6 {"Horizontal"=0, "Vertical"=4000} ("原点") T6 {"Horizontal"=0, "Vertical"=3200} ("原点")] -> w1676
          frame "温度曲线", Default {
          }
          frame "滴定曲线" {
          }
        }
        n1026 = property on="窗格" class="Pane"("Origin"=w1676) -> ()  [unwired: 2 in, 2 out]
      }
      event "历史波形", "历史波形 2": Value Change {
        n1027 = event-data() -> ("CtlRef"=w1680:refnum<vi>)  [unwired: 1 in, 5 out]
        n1028 = property class="Bool (严格)"(reference=w1680) -> ("Label.Text"=w1679:string)  [unwired: 1 in, 2 out]
        n1029 = case shown="\"历史波形2\"" w1679 {
          frame "历史波形2" {
            n1030 = call-poly <vilib>:"Read Waveforms from File.vi"() -> ("error out"=w1681:errorcluster, "first waveform in record"=w1682:waveform(dbl))  [unwired: 6 in, 2 out]
            n1031 = case shown="无错误" w1681 {
              tunnel: w1682 -> [w1685 _]
              frame No Error {
                n1032 = Unbundle By Name(w1685) -> ("t0"=w1683:timestamp, "Y"=w1684:dbl[])  [unwired: 2 out]
                n1033 = global write "COD内部交互全局.vi" "温度波形时间"(w1683) -> ()
                n1034 = global write "COD内部交互全局.vi" "时间温度曲线"(w1684) -> ()
                n1035 = global write "COD内部交互全局.vi" "时间-温度"(w1684) -> ()
              }
              frame Error {
                n1036 = One Button Dialog(message="打开失败" ("消息")) -> ()  [unwired: 1 in, 1 out]
              }
            }
          }
          frame "历史波形", Default {
            n1037 = call-poly <vilib>:"Read Waveforms from File.vi"() -> ("error out"=w1687:errorcluster, "first waveform in record"=w1688:waveform(dbl))  [unwired: 6 in, 2 out]
            n1038 = case shown="无错误" w1687 {
              tunnel: w1688 -> [w1691 _]
              frame No Error {
                n1039 = Unbundle By Name(w1691) -> ("t0"=w1689:timestamp, "Y"=w1690:dbl[])  [unwired: 2 out]
                n1040 = global write "COD内部交互全局.vi" "波形时间"(w1689) -> ()
                n1041 = global write "COD内部交互全局.vi" "ORP滴定曲线"(w1690) -> ()
                n1042 = global write "COD内部交互全局.vi" "滴定数-ORP值"(w1690) -> ()
              }
              frame Error {
                n1043 = One Button Dialog(message="打开失败" ("消息")) -> ()  [unwired: 1 in, 1 out]
              }
            }
          }
        }
      }
      event "释放串口": Value Change {
        n1044 = event-data() -> ()  [unwired: 1 in, 6 out]
        n1045 = Two Button Dialog(message="确认是否释放串口，释放串口将导致通信失败！" ("消息")) -> (T button?=w1693:bool)  [unwired: 2 in]
        n1046 = case shown="真" w1693 {
          tunnel: w1696 -> [_ w1698]
          tunnel: w1695 -> [_ w1697]
          frame False {
          }
          frame True {
            n1047 = Bundle By Name(cluster=cluster{"命令":string} {"命令"=""} ("元素"), "命令"="停用模块" ("名称（未命名）")) -> (w1699:cluster{"命令":string})
            n1048 = Enqueue Element(queue=w1698, element=w1699, error in (no error)=w1697) -> ()  [unwired: 1 in, 3 out]
          }
        }
      }
      event "打开串口": Value Change {
        n1049 = event-data() -> ()  [unwired: 1 in, 6 out]
        n1050 = flat-sequence {
          tunnel: w1703 -> [w1711]
          tunnel: w1702 -> [w1710]
          frame #0 {
            n1051 = global read "CODMn断电保存全局变量.vi" "VISA resource name"() -> (w1714:refnum<visa-resource-name>)
            n1052 = global read "CODMn断电保存全局变量.vi" "MB通信方式选择"() -> (w1707:enum16{"串口", "TCP"})
            n1053 = global read "CODMn断电保存全局变量.vi" "PORT"() -> (w1705:string)
            n1054 = global read "CODMn断电保存全局变量.vi" "IP"() -> (w1706:string)
            n1055 = call "串口配置.vi"("PORT"=w1705, "IP"=w1706, "MB通信方式选择"=w1707, "请选择串口:"=w1714) -> ("PORT 2"=w1708:string, "IP 2"=w1709:string, "确认 2"=w1712:bool, "VISA资源名称 2"=w1713:refnum<visa-resource-name>, "MB通信方式选择 2"=w1704:enum16{"串口", "TCP"})  [unwired: 3 in]
            n1056 = case shown="真" w1712 {
              tunnel: w1713 -> [_ w1723]
              tunnel: w1711 -> [_ w1719]
              tunnel: w1710 -> [_ w1718]
              tunnel: w1709 -> [_ w1717]
              tunnel: w1708 -> [_ w1716]
              tunnel: w1704 -> [_ w1715]
              frame False {
              }
              frame True {
                n1057 = global write "CODMn断电保存全局变量.vi" "IP"(w1717) -> ()
                n1058 = global write "CODMn断电保存全局变量.vi" "PORT"(w1716) -> ()
                n1059 = global write "CODMn断电保存全局变量.vi" "VISA resource name"(w1723) -> ()
                n1060 = global write "CODMn断电保存全局变量.vi" "MB通信方式选择"(w1715) -> ()
                n1061 = Bundle By Name(cluster=cluster{"命令":string} {"命令"=""} ("元素"), "命令"="启用模块" ("名称（未命名）")) -> (w1720:cluster{"命令":string})
                n1062 = Enqueue Element(queue=w1719, element=w1720, error in (no error)=w1718) -> ()  [unwired: 1 in, 3 out]
              }
            }
          }
          frame #1 {
            n1063 = call "配置文件保存.vi"() -> ()  [unwired: 12 in]
          }
        }
      }
      event "更新程序": Value Change {
        n1064 = event-data() -> ("CtlRef"=w1726:refnum<vi>, "NewVal"=w1727:bool)  [unwired: 1 in, 4 out]
        n1065 = case shown="真" w1727 {
          tunnel: w1726 -> [_ w1736]
          tunnel: w1725 -> [w1729 w1735]
          tunnel: w1724 -> [w1728 w1734]
          frame False {
            n1066 = Bundle By Name(cluster=cluster{"命令":string} {"命令"=""} ("元素"), "命令"="启用模块" ("名称（未命名）")) -> (w1730:cluster{"命令":string})
            n1067 = Enqueue Element(queue=w1729, element=w1730, error in (no error)=w1728) -> ()  [unwired: 1 in, 3 out]
          }
          frame True {
            n1068 = Two Button Dialog(message="警告，非专业人士请勿进行此操作！！！\n请确认是否继续？" ("消息")) -> (T button?=w1738:bool)  [unwired: 2 in]
            n1069 = case shown="真" w1738 {
              tunnel: w1736 -> [w1754 _]
              tunnel: w1735 -> [_ w1762]
              tunnel: w1734 -> [_ w1761]
              tunnel: [errorcluster {"status"=TRUE, "code"=0, "source"=""} ("error out") w1755] -> w1733
              frame False {
                n1070 = property class="Bool (严格)"(reference=w1754, "Value"=FALSE ("释放串口")) -> ()  [unwired: 1 in, 2 out]
              }
              frame True {
                n1071 = Bundle By Name(cluster=cluster{"命令":string} {"命令"=""} ("元素"), "命令"="CODMn程序更新" ("名称（未命名）")) -> (w1765:cluster{"命令":string})
                n1072 = Enqueue Element(queue=w1762, element=w1765, error in (no error)=w1761) -> (queue out=w1760:refnum<queue>, error out=w1759:errorcluster)  [unwired: 1 in, 1 out]
                n1073 = Bundle By Name(cluster=cluster{"命令":string} {"命令"=""} ("元素"), "命令"="停用模块" ("名称（未命名）")) -> (w1756:cluster{"命令":string})
                n1074 = Enqueue Element(queue=w1760, element=w1756, error in (no error)=w1759) -> (error out=w1755:errorcluster)  [unwired: 1 in, 2 out]
              }
            }
            n1075 = case shown="无错误" w1733 {
              frame No Error {
                n1076 = call "文件对话框"("start path"=path "D:/SRC") -> ("selected path"=w1741:path, "cancelled"=w1739:bool)  [unwired: 11 in, 2 out]
                n1077 = case shown="假" w1739 {
                  tunnel: w1741 -> [w1746 _]
                  frame False {
                    n1078 = Path To String(path=w1746) -> (string=w1743:string)
                    n1079 = Format Into String(format string="  - \"%s\"" ("格式字符串"), initial string="\"C:\\Program Files\\Fatek\\WinProladder\\WProlad.exe\"" ("command line"), w1743) -> (resulting string=w1744:string)  [unwired: 1 in, 1 out]
                    n1080 = call <vilib>:"System Exec.vi"("command line"=w1744) -> ("error out"=w1747:errorcluster)  [unwired: 7 in, 3 out]
                    n1081 = case shown="错误" w1747 {
                      tunnel: w1743 -> [_ w1750]
                      frame No Error {
                      }
                      frame Error {
                        n1082 = Format Into String(format string="  - \"%s\"" ("格式字符串"), initial string="\"C:\\Program Files (x86)\\Fatek\\WinProladder\\WProlad.exe\"" ("command line"), w1750) -> (resulting string=w1748:string)  [unwired: 1 in, 1 out]
                        n1083 = call <vilib>:"System Exec.vi"("command line"=w1748) -> ()  [unwired: 7 in, 4 out]
                      }
                    }
                  }
                  frame True {
                  }
                }
              }
              frame Error {
              }
            }
          }
        }
      }
      event "序列号变更": Value Change {
        n1084 = event-data() -> ()  [unwired: 1 in, 6 out]
        n1085 = local read "CODMn序列号"() -> (w1769:string)
        n1086 = call "序列号写入.vi"("序列号:"=w1769) -> ("确认 2"=w1766:bool, "序列号输出"=w1770:string)  [unwired: 9 in]
        n1087 = case shown="真" w1766 {
          tunnel: w1770 -> [_ w1776]
          tunnel: w1768 -> [_ w1772]
          tunnel: w1767 -> [_ w1771]
          frame False {
          }
          frame True {
            n1088 = global write "COD内部交互全局.vi" "序列号:"(w1776) -> ()
            n1089 = Bundle By Name(cluster=cluster{"命令":string} {"命令"=""} ("元素"), "命令"="CODMn序列号写入" ("名称（未命名）")) -> (w1773:cluster{"命令":string})
            n1090 = Enqueue Element(queue=w1772, element=w1773, error in (no error)=w1771) -> ()  [unwired: 1 in, 3 out]
          }
        }
      }
      event Timeout {
        n1091 = event-data() -> ()  [unwired: 1 in, 3 out]
      }
    }
  }
  n1092 = while {
    stop <- FALSE stop-if-true
    # "数字键盘输入"
    n1093 = event shown="[22] \"跨度液浓度\", \"零点核查浓度\", \"标样浓度\", \"标准液偏差\", \"跨度液偏差\", \"零点液偏差\": 鼠标按下" {
      selector: _ -> [_ _ _ _ _ _ _ _ _ _ _ _ _ _ _ _ _ _ _ _ _ _ _ _ _ _ _ _ _ _ _]
      dyn-events: _ -> [_ _ _ _ _ _ _ _ _ _ _ _ _ _ _ _ _ _ _ _ _ _ _ _ _ _ _ _ _ _ _]
      timeout: _ -> [_ _ _ _ _ _ _ _ _ _ _ _ _ _ _ _ _ _ _ _ _ _ _ _ _ _ _ _ _ _ _]
      event Timeout {
        n1094 = event-data() -> ()  [unwired: 1 in, 3 out]
      }
      event "温度": Mouse Down {
        n1095 = event-data() -> ()  [unwired: 1 in, 8 out]
        n1096 = local read "温度"() -> (w1779:dbl)
        n1097 = call "数字键盘.vi"("OldNumber"=w1779) -> ("NewNumber"=w1778:sgl)
        n1098 = local write "温度"(w1778) -> ()
      }
      event "恒温时间": Mouse Down {
        n1099 = event-data() -> ()  [unwired: 1 in, 8 out]
        n1100 = local read "恒温时间"() -> (w1780:dbl)
        n1101 = call "数字键盘.vi"("OldNumber"=w1780) -> ("NewNumber"=w1781:sgl)
        n1102 = local write "恒温时间"(w1781) -> ()
      }
      event "标准液浓度": Mouse Down {
        n1103 = event-data() -> ()  [unwired: 1 in, 8 out]
        n1104 = local read "标准液浓度"() -> (w1783:dbl)
        n1105 = call "数字键盘.vi"("OldNumber"=w1783) -> ("NewNumber"=w1782:sgl)
        n1106 = local write "标准液浓度"(w1782) -> ()
      }
      event "氢氧化钠：": Mouse Down {
        n1107 = event-data() -> ()  [unwired: 1 in, 8 out]
        n1108 = local read "氢氧化钠："() -> (w1784:dbl)
        n1109 = call "数字键盘.vi"("OldNumber"=w1784) -> ("NewNumber"=w1785:sgl)
        n1110 = local write "氢氧化钠："(w1785) -> ()
      }
      event "水样：": Mouse Down {
        n1111 = event-data() -> ()  [unwired: 1 in, 8 out]
        n1112 = local read "水样："() -> (w1786:dbl)
        n1113 = call "数字键盘.vi"("OldNumber"=w1786) -> ("NewNumber"=w1787:sgl)
        n1114 = local write "水样："(w1787) -> ()
      }
      event "蒸馏水：": Mouse Down {
        n1115 = event-data() -> ()  [unwired: 1 in, 8 out]
        n1116 = local read "蒸馏水："() -> (w1788:dbl)
        n1117 = call "数字键盘.vi"("OldNumber"=w1788) -> ("NewNumber"=w1789:sgl)
        n1118 = local write "蒸馏水："(w1789) -> ()
      }
      event "标液：": Mouse Down {
        n1119 = event-data() -> ()  [unwired: 1 in, 8 out]
        n1120 = local read "标液："() -> (w1790:dbl)
        n1121 = call "数字键盘.vi"("OldNumber"=w1790) -> ("NewNumber"=w1791:sgl)
        n1122 = local write "标液："(w1791) -> ()
      }
      event "零点核查样：": Mouse Down {
        n1123 = event-data() -> ()  [unwired: 1 in, 8 out]
        n1124 = local read "零点核查样："() -> (w1792:dbl)
        n1125 = call "数字键盘.vi"("OldNumber"=w1792) -> ("NewNumber"=w1793:sgl)
        n1126 = local write "零点核查样："(w1793) -> ()
      }
      event "加标回收样：": Mouse Down {
        n1127 = event-data() -> ()  [unwired: 1 in, 8 out]
        n1128 = local read "加标回收样："() -> (w1794:dbl)
        n1129 = call "数字键盘.vi"("OldNumber"=w1794) -> ("NewNumber"=w1795:sgl)
        n1130 = local write "加标回收样："(w1795) -> ()
      }
      event "草酸钠": Mouse Down {
        n1131 = event-data() -> ()  [unwired: 1 in, 8 out]
        n1132 = local read "草酸钠"() -> (w1796:dbl)
        n1133 = call "数字键盘.vi"("OldNumber"=w1796) -> ("NewNumber"=w1797:sgl)
        n1134 = local write "草酸钠"(w1797) -> ()
      }
      event "高锰酸钾": Mouse Down {
        n1135 = event-data() -> ()  [unwired: 1 in, 8 out]
        n1136 = local read "高锰酸钾"() -> (w1798:dbl)
        n1137 = call "数字键盘.vi"("OldNumber"=w1798) -> ("NewNumber"=w1799:sgl)
        n1138 = local write "高锰酸钾"(w1799) -> ()
      }
      event "硫酸": Mouse Down {
        n1139 = event-data() -> ()  [unwired: 1 in, 8 out]
        n1140 = local read "硫酸"() -> (w1800:dbl)
        n1141 = call "数字键盘.vi"("OldNumber"=w1800) -> ("NewNumber"=w1801:sgl)
        n1142 = local write "硫酸"(w1801) -> ()
      }
      event "零点泵计量数 2": Mouse Down {
        n1143 = event-data() -> ()  [unwired: 1 in, 8 out]
        n1144 = local read "零点泵计量数 2"() -> (w1802:dbl)
        n1145 = call "数字键盘.vi"("OldNumber"=w1802) -> ("NewNumber"=w1803:sgl)
        n1146 = local write "零点泵计量数 2"(w1803) -> ()
      }
      event "标度泵计量数 2": Mouse Down {
        n1147 = event-data() -> ()  [unwired: 1 in, 8 out]
        n1148 = local read "标度泵计量数 2"() -> (w1804:dbl)
        n1149 = call "数字键盘.vi"("OldNumber"=w1804) -> ("NewNumber"=w1805:sgl)
        n1150 = local write "标度泵计量数 2"(w1805) -> ()
      }
      event "高量程稀释倍数:": Mouse Down {
        n1151 = event-data() -> ()  [unwired: 1 in, 8 out]
        n1152 = local read "高量程稀释倍数:"() -> (w1807:i8)
        n1153 = call "数字键盘.vi"("OldNumber"=w1807) -> ("NewNumber"=w1806:sgl)
        n1154 = local write "高量程稀释倍数:"(w1806) -> ()
      }
      event "低量程稀释倍数:": Mouse Down {
        n1155 = event-data() -> ()  [unwired: 1 in, 8 out]
        n1156 = local read "低量程稀释倍数:"() -> (w1809:i8)
        n1157 = call "数字键盘.vi"("OldNumber"=w1809) -> ("NewNumber"=w1808:sgl)
        n1158 = local write "低量程稀释倍数:"(w1808) -> ()
      }
      event "浓度1": Mouse Down {
        n1159 = event-data() -> ()  [unwired: 1 in, 8 out]
        n1160 = local read "浓度1"() -> (w1811:dbl)
        n1161 = call "数字键盘.vi"("OldNumber"=w1811) -> ("NewNumber"=w1810:sgl)
        n1162 = property on="浓度1" class="DigNum (严格)"("Val(Sgnl)"=w1810) -> ()  [unwired: 2 in, 2 out]
      }
      event "浓度2": Mouse Down {
        n1163 = event-data() -> ()  [unwired: 1 in, 8 out]
        n1164 = local read "浓度2"() -> (w1813:dbl)
        n1165 = call "数字键盘.vi"("OldNumber"=w1813) -> ("NewNumber"=w1812:sgl)
        n1166 = property on="浓度2" class="DigNum (严格)"("Val(Sgnl)"=w1812) -> ()  [unwired: 2 in, 2 out]
      }
      event "浓度3": Mouse Down {
        n1167 = event-data() -> ()  [unwired: 1 in, 8 out]
        n1168 = local read "浓度3"() -> (w1815:dbl)
        n1169 = call "数字键盘.vi"("OldNumber"=w1815) -> ("NewNumber"=w1814:sgl)
        n1170 = property on="浓度3" class="DigNum (严格)"("Val(Sgnl)"=w1814) -> ()  [unwired: 2 in, 2 out]
      }
      event "浓度4": Mouse Down {
        n1171 = event-data() -> ()  [unwired: 1 in, 8 out]
        n1172 = local read "浓度4"() -> (w1817:dbl)
        n1173 = call "数字键盘.vi"("OldNumber"=w1817) -> ("NewNumber"=w1816:sgl)
        n1174 = property on="浓度4" class="DigNum (严格)"("Val(Sgnl)"=w1816) -> ()  [unwired: 2 in, 2 out]
      }
      event "浓度5": Mouse Down {
        n1175 = event-data() -> ()  [unwired: 1 in, 8 out]
        n1176 = local read "浓度5"() -> (w1819:dbl)
        n1177 = call "数字键盘.vi"("OldNumber"=w1819) -> ("NewNumber"=w1818:sgl)
        n1178 = property on="浓度5" class="DigNum (严格)"("Val(Sgnl)"=w1818) -> ()  [unwired: 2 in, 2 out]
      }
      event "跨度液浓度", "零点核查浓度", "标样浓度", "标准液偏差", "跨度液偏差", "零点液偏差": Mouse Down {
        n1179 = event-data() -> ("CtlRef"=w1823:refnum<vi>)  [unwired: 1 in, 7 out]
        n1180 = property class="DigNum (严格)"(reference=w1823) -> (reference out=w1820:refnum<vi>, "Value"=w1822:dbl)  [unwired: 1 in, 1 out]
        n1181 = call "数字键盘.vi"("OldNumber"=w1822) -> ("NewNumber"=w1821:sgl)
        n1182 = property class="DigNum (严格)"(reference=w1820, "Val(Sgnl)"=w1821) -> ()  [unwired: 1 in, 2 out]
      }
      event "泵滴定数1": Mouse Down {
        n1183 = event-data() -> ()  [unwired: 1 in, 8 out]
        n1184 = local read "泵滴定数1"() -> (w1825:dbl)
        n1185 = call "数字键盘.vi"("OldNumber"=w1825) -> ("NewNumber"=w1824:sgl)
        n1186 = property on="泵滴定数1" class="DigNum (严格)"("Val(Sgnl)"=w1824) -> ()  [unwired: 2 in, 2 out]
      }
      event "泵滴定数2": Mouse Down {
        n1187 = event-data() -> ()  [unwired: 1 in, 8 out]
        n1188 = local read "泵滴定数2"() -> (w1827:dbl)
        n1189 = call "数字键盘.vi"("OldNumber"=w1827) -> ("NewNumber"=w1826:sgl)
        n1190 = property on="泵滴定数2" class="DigNum (严格)"("Val(Sgnl)"=w1826) -> ()  [unwired: 2 in, 2 out]
      }
      event "泵滴定数3": Mouse Down {
        n1191 = event-data() -> ()  [unwired: 1 in, 8 out]
        n1192 = local read "泵滴定数3"() -> (w1829:dbl)
        n1193 = call "数字键盘.vi"("OldNumber"=w1829) -> ("NewNumber"=w1828:sgl)
        n1194 = property on="泵滴定数3" class="DigNum (严格)"("Val(Sgnl)"=w1828) -> ()  [unwired: 2 in, 2 out]
      }
      event "泵滴定数4": Mouse Down {
        n1195 = event-data() -> ()  [unwired: 1 in, 8 out]
        n1196 = local read "泵滴定数4"() -> (w1831:dbl)
        n1197 = call "数字键盘.vi"("OldNumber"=w1831) -> ("NewNumber"=w1830:sgl)
        n1198 = property on="泵滴定数4" class="DigNum (严格)"("Val(Sgnl)"=w1830) -> ()  [unwired: 2 in, 2 out]
      }
      event "泵滴定数5": Mouse Down {
        n1199 = event-data() -> ()  [unwired: 1 in, 8 out]
        n1200 = local read "泵滴定数5"() -> (w1833:dbl)
        n1201 = call "数字键盘.vi"("OldNumber"=w1833) -> ("NewNumber"=w1832:sgl)
        n1202 = property on="泵滴定数5" class="DigNum (严格)"("Val(Sgnl)"=w1832) -> ()  [unwired: 2 in, 2 out]
      }
      event "低切高阈值:", "高切低阈值:": Mouse Down {
        n1203 = event-data() -> ("CtlRef"=w1837:refnum<vi>)  [unwired: 1 in, 7 out]
        n1204 = property class="DigNum (严格)"(reference=w1837) -> (reference out=w1836:refnum<vi>, "Value"=w1835:dbl)  [unwired: 1 in, 1 out]
        n1205 = call "数字键盘.vi"("OldNumber"=w1835) -> ("NewNumber"=w1834:sgl)
        n1206 = property class="DigNum (严格)"(reference=w1836, "Val(Sgnl)"=w1834) -> ()  [unwired: 1 in, 2 out]
      }
      event "公式切换阈值滴定数(0-9999)": Mouse Down {
        n1207 = event-data() -> ("CtlRef"=w1838:refnum<vi>)  [unwired: 1 in, 7 out]
        n1208 = property class="DigNum (严格)"(reference=w1838) -> (reference out=w1841:refnum<vi>, "Value"=w1840:u16)  [unwired: 1 in, 1 out]
        n1209 = call "数字键盘.vi"("OldNumber"=w1840) -> ("NewNumber"=w1839:sgl)
        n1210 = property class="DigNum (严格)"(reference=w1841, "Value"=w1839) -> ()  [unwired: 1 in, 2 out]
      }
      event "远程校准量程", "远程标样校准": Value Change {
        n1211 = event-data() -> ()  [unwired: 1 in, 6 out]
        n1212 = flat-sequence {
          frame #0 {
            n1213 = global write "CODMn断电保存全局变量.vi" "远程校准量程"("远程校准量程") -> ()
            n1214 = global write "CODMn断电保存全局变量.vi" "远程标样校准"("远程标样校准") -> ()
          }
          frame #1 {
            n1215 = call "配置文件保存.vi"() -> ()  [unwired: 12 in]
          }
        }
      }
    }
  }
  n1216 = while {
    stop <- FALSE stop-if-true
    # "滚动显示"
    n1217 = global read "COD内部交互全局.vi" "待机"() -> (w1844:bool)
    n1218 = case shown="假" w1844 {
      frame False {
        # "运行中"
        n1219 = global read "COD内部交互全局.vi" "校准内容显示"() -> (w1847:string)
        n1220 = while {
          shift-right: [w1849] -> _
          shift-left: w1847 -> [w1854]
          stop <- w1848 stop-if-true
          (unwired) "仪器校准中!\n当前校准浓度为:3mg/L" ("校准内容显示")
          n1221 = Wait (ms)(milliseconds to wait=u32 500 ("等待时间（毫秒）")) -> ()  [unwired: 1 out]
          n1222 = Spreadsheet String To Array(delimiter (Tab)="\n" ("分隔符(Tab)"), format string="" ("格式字符串"), spreadsheet string=w1854, array type (2D Dbl)=string[] []) -> (array=w1857:string[])
          n1223 = for {
            tunnel: w1857 -> [w1865] mode=indexing
            tunnel: [w1863] -> _ mode=indexing
            shift-right: [w1861] -> w1852
            shift-left: "" ("格式字符串") -> [w1862]
            n1224 = call "字符串移位显示.vi"("字符框大小"=36, "字符串输入"=w1865) -> ("移位后字符串"=w1863:string)  [unwired: 8 in, 1 out]
            n1225 = Concatenate Strings(w1862, w1863, "\n" ("分隔符(Tab)")) -> (w1861:string)
          }
          n1226 = String Length(string=w1852) -> (length=w1851:i32)
          n1227 = Decrement(x=w1851) -> (x-1=w1850:i32)
          n1228 = String Subset(string=w1852, length (rest)=w1850) -> (substring=w1849:string)  [unwired: 1 in]
          "校准内容显示" <- w1849
          n1229 = global read "COD内部交互全局.vi" "待机"() -> (w1848:bool)
        }
      }
      frame True {
      }
    }
    n1230 = Wait (ms)(milliseconds to wait=u32 1000 ("等待时间（毫秒）")) -> ()  [unwired: 1 out]
  }
  n1231 = property class="VI"(reference=w8, error in=w5) -> ("Name"=w9:string)  [unwired: 2 out]
  n1232 = while {
    stop <- FALSE stop-if-true
    # "相差60秒自动校时"
    n1233 = global read "运行时序全局变量.vi" "多列列表框"() -> (w1869:i32)
    n1234 = local read "仪器时间"() -> (w1876:timestamp)
    n1235 = local read "系统时间"() -> (w1877:timestamp)
    n1236 = local read "消解温度℃"() -> (w1866:dbl)
    n1237 = Wait (ms)(milliseconds to wait=u32 1000 ("等待时间（毫秒）")) -> ()  [unwired: 1 out]
    n1238 = Build Array(w1876) -> (w1875:timestamp[])
    n1239 = Build Array(w1877) -> (w1894:timestamp[])
    n1240 = Equal?(x=w1869, y=u16 5) -> (x = y?=w1871:bool)
    n1241 = call "消解压力计算.vi"("当前消解温度"=w1866) -> ("消解压力"=→"消解压力kPa":dbl)  [unwired: 10 in]
    n1242 = call <vilib>:"Boolean Crossing PtByPt.vi"("direction"=enum16{"either", "false-true", "true-false"}."false-true", "input"=w1871) -> ("crossing"=w1868:bool)  [unwired: 1 in]
    n1243 = call "DateToHex.vi"("DATE"=w1875) -> ("数组"=w1888:u16[])  [unwired: 10 in]
    n1244 = call "DateToHex.vi"("DATE"=w1894) -> ("数组"=w1893:u16[])  [unwired: 10 in]
    n1245 = case shown="真" w1868 {
      frame False {
      }
      frame True {
        # "校准结束后自动更新曲线泵滴定数"
        n1246 = global read "COD测量模式全局.vi" "测量模式文字实时"() -> (w1895:string)
        n1247 = global read "COD测量模式全局.vi" "测量模式文字实时"() -> (w1900:string)
        n1248 = global read "CODMN外部API.vi" "远程反控校准CODMn"() -> (w1899:bool)
        n1249 = global read "COD内部交互全局.vi" "高锰酸钾"() -> (w1903:dbl)
        n1250 = Equal?(x=w1895, y="校零") -> (x = y?=w1896:bool)
        n1251 = Equal?(x=w1900, y="校标") -> (x = y?=w1902:bool)
        n1252 = Or(x=w1896, y=w1902) -> (x .or. y?=w1898:bool)
        n1253 = case shown="真" w1898 {
          tunnel: w1903 -> [_ w1908]
          tunnel: w1895 -> [_ w1907]
          frame False {
          }
          frame True {
            w1916 = "量程选择" ("section")
            n1254 = global read "COD内部交互全局.vi" "数据存储时间戳"() -> (w1905:timestamp)
            n1255 = global read "CODMN外部API.vi" "ping"() -> (w1927:bool)
            n1256 = case shown="\"校零\"" w1907 {
              tunnel: ["标样校准时间：" "空白校准时间："] -> _
              frame "校标", Default {
              }
              frame "校零" {
              }
            }
            n1257 = case shown="假" w1927 {
              tunnel: [w1936 w1939] -> w1928
              frame False {
                n1258 = global read "COD内部交互全局.vi" "配置文件ini"() -> (w1938:string)
                n1259 = call <vilib>:"Application Directory.vi"() -> ("Application Directory"=w1937:path)
                n1260 = Build Path(base path=w1937, name or relative path=w1938) -> (appended path=w1936:path)
              }
              frame True {
                n1261 = global read "CODMN外部API.vi" "配置文件 path"() -> (w1939:path)
              }
            }
            n1262 = Format Date/Time String(time format string (%c)="%Y/%m/%d %H:%M:%S" ("时间格式字符串(%c)"), seconds (now)=w1905) -> ()  [unwired: 1 in, 1 out]
            n1263 = call <vilib>:"Open Config Data.vi"("configuration file path"=w1928) -> ("error out"=w1915:errorcluster, "refnum"=w1914:T8)  [unwired: 8 in, 1 out]
            n1264 = call-poly <vilib>:"Read Key.vi"("section"="标线选择", "error in (no error)"=w1915, "key"="选用水样", "refnum"=w1914) -> ("error out"=w1917:errorcluster, "value"=w1910:i32, "refnum out"=w1918:T8)  [unwired: 4 in, 1 out]
            n1265 = local write "选用水样"(w1910) -> ()
            n1266 = call-poly <vilib>:"Read Key.vi"("section"=w1916, "error in (no error)"=w1917, "key"=w1916, "refnum"=w1918) -> ("error out"=w1911:errorcluster, "value"=w1913:i32, "refnum out"=w1912:T8)  [unwired: 4 in, 1 out]
            n1267 = case shown="1" w1910 {
              tunnel: ["葡萄糖标线" ("section") "草酸钠标线" ("section")] -> w1925
              frame 0, Default {
              }
              frame 1 {
              }
            }
            n1268 = local write "量程选择"(w1913) -> ()
            n1269 = case shown="2" w1913 {
              tunnel: ["低量程" "高量程" "0-2量程"] -> w1924
              frame 0, Default {
              }
              frame 1 {
              }
              frame 2 {
              }
            }
            n1270 = Concatenate Strings(w1925, w1924) -> (w1926:string)
            n1271 = call-poly <vilib>:"Read Key.vi"("section"=w1926, "error in (no error)"=w1911, "key"="当前选用的校准" ("section"), "refnum"=w1912) -> ("error out"=w1923:errorcluster, "value"=w1906:i32, "refnum out"=w1922:T8)  [unwired: 4 in, 1 out]
            n1272 = case shown="5" w1906 {
              tunnel: w1905 -> [w1929 w1930 w1931 w1932 w1933]
              frame 1, Default {
                "零点校准时间" <- w1929
              }
              frame 2 {
                "标液校准时间1" <- w1930
              }
              frame 3 {
                "标液校准时间2" <- w1931
              }
              frame 4 {
                "标液校准时间3" <- w1932
              }
              frame 5 {
                "标液校准时间4" <- w1933
              }
            }
            n1273 = call <vilib>:"Close Config Data.vi"("error in (no error)"=w1923, "refnum"=w1922) -> ()  [unwired: 8 in, 2 out]
            n1274 = global write "COD内部交互全局.vi" "当前校准"(w1906) -> ()
            n1275 = case shown="5" w1906 {
              tunnel: w1908 -> [w1945 w1946 w1947 w1948 w1949]
              frame 1, Default {
                n1276 = property on="泵滴定数1" class="DigNum (严格)"("Val(Sgnl)"=w1945) -> ()  [unwired: 2 in, 2 out]
              }
              frame 2 {
                n1277 = property on="泵滴定数2" class="DigNum (严格)"("Val(Sgnl)"=w1946) -> ()  [unwired: 2 in, 2 out]
              }
              frame 3 {
                n1278 = property on="泵滴定数3" class="DigNum (严格)"("Val(Sgnl)"=w1947) -> ()  [unwired: 2 in, 2 out]
              }
              frame 4 {
                n1279 = property on="泵滴定数4" class="DigNum (严格)"("Val(Sgnl)"=w1948) -> ()  [unwired: 2 in, 2 out]
              }
              frame 5 {
                n1280 = property on="泵滴定数5" class="DigNum (严格)"("Val(Sgnl)"=w1949) -> ()  [unwired: 2 in, 2 out]
              }
            }
          }
        }
        n1281 = case shown="真" w1899 {
          frame False {
          }
          frame True {
            # "校准完自动写入公式"
            n1282 = global write "CODMN外部API.vi" "远程反控校准CODMn"(FALSE ("远程反控校准CODMn")) -> ()
          }
        }
      }
    }
    n1283 = Index Array(array=w1888, index=2 ("索引")) -> (element=w1890:u16)
    n1284 = Index Array(array=w1893, index=2 ("索引")) -> (element=w1891:u16)
    n1285 = Split Number(x=w1890) -> (hi(x)=w1884:u8)  [unwired: 1 out]
    n1286 = Split Number(x=w1891) -> (hi(x)=w1887:u8)  [unwired: 1 out]
    n1287 = To Byte Integer(number=w1884) -> (8bit integer=w1883:i8)
    n1288 = To Byte Integer(number=w1887) -> (8bit integer=w1886:i8)
    n1289 = Subtract(x=w1883, y=w1886) -> (x-y=w1885:i8)
    n1290 = Absolute Value(x=w1885) -> (abs(x)=w1882:i8)
    n1291 = local read "通讯状态"() -> (w1879:bool)
    n1292 = Greater Or Equal?(x=w1882, y=i8 5) -> (x >= y?=w1880:bool)
    n1293 = And(x=w1880, y=w1879) -> (x .and. y?=w1878:bool)
    n1294 = case shown="真" w1878 {
      frame False {
      }
      frame True {
        # "相差60秒时间自动校准"
        n1295 = flat-sequence {
          frame #0 {
            n1296 = property on="时间校准" class="Bool (严格)"("Val(Sgnl)"=TRUE ("值(信号)")) -> ()  [unwired: 2 in, 2 out]
          }
          frame #1 {
            n1297 = Wait (ms)(milliseconds to wait=u32 500 ("等待时间（毫秒）")) -> ()  [unwired: 1 out]
          }
          frame #2 {
            n1298 = property on="时间校准" class="Bool (严格)"("Val(Sgnl)"=FALSE ("值(信号)")) -> ()  [unwired: 2 in, 2 out]
          }
        }
      }
    }
  }
  n1299 = Open VI Reference(type specifier VI Refnum (for type only)=refnum<vi> refnum, vi path=w9, options=128 ("选项")) -> (vi reference=w11:refnum<vi>, error out=w13:errorcluster)  [unwired: 3 in]
  n1300 = call-by-ref "?"(reference=w11, error in=w13) -> (reference out=w15:refnum<vi>, error out=w14:errorcluster)  [unwired: 12 in]
  n1301 = Close Reference(reference=w15, error in (no error)=w14) -> ()  [unwired: 1 out]
  n1302 = while {
    stop <- FALSE stop-if-true
    n1303 = Wait (ms)(milliseconds to wait=u32 1000 ("等待时间（毫秒）")) -> ()  [unwired: 1 out]
    n1304 = case shown="真" "存校准信息" {
      frame False {
      }
      frame True {
        n1305 = local read "公式系数"() -> (w1958:dbl[])
        n1306 = local read "泵滴定数2"() -> (w1980:dbl)
        n1307 = local read "泵滴定数4"() -> (w1978:dbl)
        n1308 = local read "泵滴定数3"() -> (w1979:dbl)
        n1309 = local read "泵滴定数5"() -> (w1977:dbl)
        n1310 = local read "泵滴定数1"() -> (w1981:dbl)
        n1311 = local read "浓度1"() -> (w1987:dbl)
        n1312 = local read "浓度2"() -> (w1983:dbl)
        n1313 = local read "浓度3"() -> (w1984:dbl)
        n1314 = local read "浓度4"() -> (w1985:dbl)
        n1315 = local read "浓度5"() -> (w1986:dbl)
        n1316 = local read "标液校准时间1"() -> (w1966:timestamp)
        n1317 = local read "标液校准时间2"() -> (w1965:timestamp)
        n1318 = local read "标液校准时间3"() -> (w1964:timestamp)
        n1319 = local read "零点校准时间"() -> (w1967:timestamp)
        n1320 = local read "标液校准时间4"() -> (w1963:timestamp)
        n1321 = Build Array(w1981, w1980, w1979, w1978, w1977) -> (w1976:dbl[])
        n1322 = Build Array(w1987, w1983, w1984, w1985, w1986) -> (w1982:dbl[])
        n1323 = local write "存校准信息"(FALSE ("存校准信息")) -> ()
        n1324 = for {
          tunnel: w1958 -> [w1990] mode=indexing
          tunnel: [w1989] -> w1957 mode=indexing
          n1325 = Number To Fractional String(number=w1990, precision (6)=i16 6 ("宽度(-)")) -> (F-format string=w1989:string)  [unwired: 2 in]
        }
        n1326 = for {
          tunnel: w1982 -> [w1999] mode=indexing
          tunnel: w1976 -> [w1996] mode=indexing
          tunnel: [w1995] -> w1970 mode=indexing
          tunnel: [w1994] -> w1969 mode=indexing
          n1327 = Number To Decimal String(number=w1999, width (-)=i16 0 ("宽度(-)")) -> (decimal integer string=w1995:string)
          n1328 = Number To Decimal String(number=w1996, width (-)=i16 0 ("宽度(-)")) -> (decimal integer string=w1994:string)
        }
        n1329 = Build Array(w1967, w1966, w1965, w1964, w1963) -> (w1962:timestamp[])
        n1330 = local read "启用3"() -> (w1973:bool)
        n1331 = local read "启用5"() -> (w1971:bool)
        n1332 = local read "启用4"() -> (w1972:bool)
        n1333 = local read "启用2"() -> (w1974:bool)
        n1334 = local read "启用1"() -> (w1975:bool)
        n1335 = for {
          tunnel: w1962 -> [w1992] mode=indexing
          tunnel: [w1991] -> w1961 mode=indexing
          n1336 = Format Date/Time String(time format string (%c)="%Y/%m/%d %H:%M:%S" ("时间格式字符串(%c)"), seconds (now)=w1992) -> (date/time string=w1991:string)  [unwired: 1 in]
        }
        n1337 = Build Array(w1975, w1974, w1973, w1972, w1971) -> (w1968:bool[])
        n1338 = local read "量程选择"() -> (w1960:enum16{"低量程", "高量程"})
        n1339 = Array To Cluster(array=w1957) -> (cluster=w1956:T18)
        n1340 = call "生成校准信息.vi"("量程选择"=w1960, "公式系数"=w1956, "启用"=w1968, "校准时间"=w1961, "信号值"=w1969, "校准浓度"=w1970) -> ()  [unwired: 6 in]
      }
    }
  }
  n1341 = while {
    stop <- FALSE stop-if-true
    n1342 = property on="多列列表框" class="MCListbox (严格)"() -> ("Value"=w2004:i32)  [unwired: 2 in, 2 out]
    n1343 = Not Equal To 0?(x=w2004) -> (x != 0?=w2003:bool)
    n1344 = call <vilib>:"Boolean Crossing PtByPt.vi"("direction"=enum16{"either", "false-true", "true-false"}."false-true", "input"=w2003) -> ("crossing"=w2001:bool)  [unwired: 1 in]
    n1345 = Wait (ms)(milliseconds to wait=u32 1000 ("等待时间（毫秒）")) -> ()  [unwired: 1 out]
    n1346 = case shown="真" w2001 {
      frame False {
      }
      frame True {
        n1347 = property on="读取" class="Bool (严格)"("Val(Sgnl)"=TRUE ("值(信号)")) -> ()  [unwired: 2 in, 2 out]
      }
    }
  }
